vi "Text control 2 v5.5_pump-specific.vi"() -> ()   [LabVIEW 2016]
panel:
  in  "Tab Control":enum32{"Main", "Other parameters"}(tab)
  out "Line running":i32
  out "Total lines":i32
  out "Path":path=path "C:/users/rlp38/09Apr2009LTtesting/test2.txt"
  out "I vs Vg":cluster{"Y data in":dbl[], "X data in":dbl[]}[](graph)
  out "Is max":dbl format="%.2e"
  out "Id max":dbl format="%.2e"
  out "Ig max":dbl format="%.2e"
  out "Imax vs time":cluster{"Y data in":dbl[], "X data in":dbl[]}[](graph)
  out "Imin vs time":cluster{"Y data in":dbl[], "X data in":dbl[]}[](graph)
  out "I vs Vd":cluster{"Y data in":dbl[], "X data in":dbl[]}[](graph)
  in  "Script":string="#-------------------------------------------------------\n# SPM pump cleaning script\n#\n# Version 0.5\n# Author: Dimitrios Simatos\n# Last updated: 2018-01-05\n#-------------------------------------------------------\n# Description\n#\n# This script is designed to run the cleaning sequence of the SPM OEM pump.\n# This script needs to be run 4 times!\n#-------------------------------------------------------\n# Changes\n#\n# Placed initialization and hard stop commands in the beginning.\n#-------------------------------------------------------\n# Important points\n#\n# Never leave any liquid in the pump to dry after the experiments. If they dry, the residue may block the valve.\n# Always run the cleaning cycle after the experiments.\n# Use clockwise rotation when going up in valve port numbers and vice versa.\n#-------------------------------------------------------\n# Things to do before running the script\n#\n# Set time units to minutes.\n# Set filenames.\n# Replace the tubing, if necessary.\n#-------------------------------------------------------\n# Port connections\n#\n# Port 1: Waste\n# Port 2: Waste\n# Port 3: Various cleaning liquids\n# Port 4: Waste\n# Port 5: Waste\n# Port 6: Waste\n#\n# Between each of the 4 runs, the settings of Port 3 will change, according to the cleaning protocol.\n# The settings for Port 3 are:\n# 1st run: 1% v/v solution of sodium hypochlorite in ultrapure water\n# 2nd run: 0.1% w/v solution of sodium dodecyl sulfate in ultrapure water\n# 3rd run: Ultrapure water\n# 4th run: Waste (in air, not immersed in liquid)\n#-------------------------------------------------------\n# Cleaning protocol for the SPM OEM pump (from the manual)\n#\n# A cleaning procedure should be performed at the end of each day or in between two different experiments.\n# An effective cleaning can be performed in the following manner:\n# • Bleach solution to kill microorganisms\n# 1. Prepare a solution of 1% chlorine bleach and deionized water\n#    NOTE: Prepare a 1% v/v solution of sodium hypochlorite in deionized water\n# 2. Prepare a reservoir and place 1 tubing in the bleach solution and 5 tubings in a waste recipient\n# 3. Pick up the bleach solution through 1 port to entirely fill the syringe\n# 4. Sequentially output the syringe content through the remaining ports and throw it to the waste\n# 5. Repeat operation at least 2 times\n# • Detergent solution to remove debris\n# 1. Prepare a solution of 0.1% detergent and deionized water\n#    NOTE: Prepare a 0.1% w/v solution of sodium dodecyl sulfate in deionized water\n# 2. Move the tubing from the bleach solution reservoir and place it into a reservoir of detergent solution\n# 3. Pick up the detergent solution through 1 port to entirely fill the syringe\n# 4. Sequentially output the detergent solution through the remaining ports into the waste recipient\n# 5. Repeat operation at least 2 times\n# • Rinsing water to prepare the pump for your next experiment\n# 1. Move the tubing from the detergent solution reservoir and place it into a reservoir of deionized water\n# 2. Pick up the rinsing solution through 1 port to entirely fill the syringe\n# 3. Sequentially output the rinse water through the remaining ports into the waste recipient\n# 4. Repeat operation at least 2 times\n# • Replace the tubing, if necessary\n#-------------------------------------------------------\n# Pumping cycles and execution time\n#\n# Execution time for a single cycle: 6 x (1 min + 10 sec) = 7 minutes\n# Total execution time: 4 x 7 = 28 minutes\n# Since the script has to run 4 times, the cleaning lasts for: 4 x 28 = 112 minutes\n# Air must be the last to be pumped through the valve, to remove all liquids.\n# There are 4 pumping cycles. Each one draws a different liquid through port 3 and pumps it sequentially through ports 1,2,4,5,6.\n# During the sequential pumping, each port receives 200 ml of liquid (20% of the total syringe volume = 600 \"plunger units\")\n# The device must be disconnected from the port during the cleaning procedure.\n# All cycles are similar, except cycle 1 has the initialization command uncommented and the first report valve command commented.\n#-------------------------------------------------------\n# Volume of liquid needed\n#\n# Volume of liquid needed per cycle: 1 ml\n# Total volume of liquid needed per script run: 4 x 1 = 4 ml\n# Since the script has to run 4 times, the first 3 with different liquids, I need:\n# 4 ml of 1% v/v solution of sodium hypochlorite in ultrapure water\n# 4 ml of 0.1% w/v solution of sodium dodecyl sulfate in ultrapure water\n# 4 ml of ultrapure water\n#-------------------------------------------------------\n# Parameters\n#\n# Syringe size: 1 ml\n# Step resolution N = 0.01 mm\n# Drawing flow V = 300 pulses/second (6000 ul/min)\n# Pumping flow V = 300 pulses/second (6000 ul/min)\n#-------------------------------------------------------\n# Pump initialization\npump /1T #hard stop pump\npump /1ZR #initialize pump\n#-------------------------------------------------------\n# Cycle 1\n# Fill the syringe\npump /1Q #query pump\npump /1? #report absolute plunger position\n#pump /1?6 #report valve position\nwait-min 1 #wait 1 minute\npump /1N0R #set step resolution: 0.01 mm\npump /1Q #query pump\npump /1? #report absolute plunger position (the plunger should be at 0)\npump /1?6 #report valve position\nwait 1000 #wait 1 second\npump /1V300R #choose speed: 300 steps/s (6000 ul/min)\npump /1Q #query pump\nwait 1000 #wait 1 second\npump /1I3R #go to port 3, clockwise rotation\npump /1Q #query pump\npump /1?6 #report valve position\nwait 1000 #wait 1 second\npump /1A3000R #go to absolute position 3000 (= draw 1 ml)\nwait 30000 #wait 30 seconds\npump /1Q #query pump\npump /1? #report absolute plunger position (the plunger should have finished moving)\n#pump /1?6 #report valve position\n# The sequential pumping begins\n# Port 1\npump /1O1R #switch to port 1, counterclockwise rotation\npump /1Q #query pump\npump /1?6 #report valve position\npump /1A2400R #go to absolute position 2400 (= pump 200 ul)\npump /1Q #query pump\npump /1? #report absolute plunger position (the plunger should be moving to 0)\nwait-min 1 #wait 1 minute\npump /1? #report absolute plunger position (the plunger should have finished moving)\n# Port 2\npump /1I2R #switch to port 2, clockwise rotation\npump /1Q #query pump\npump /1?6 #report valve position\npump /1A1800R #go to absolute position 1800 (= pump 200 ul)\npump /1Q #query pump\npump /1? #report absolute plunger position (the plunger should be moving to 0)\nwait-min 1 #wait 1 minute\npump /1? #report absolute plunger position (the plunger should have finished moving)\n# Port 4\npump /1I4R #switch to port 4, clockwise rotation\npump /1Q #query pump\npump /1?6 #report valve position\npump /1A1200R #go to absolute position 1200 (= pump 200 ul)\npump /1Q #query pump\npump /1? #report absolute plunger position (the plunger should be moving to 0)\nwait-min 1 #wait 1 minute\npump /1? #report absolute plunger position (the plunger should have finished moving)\n# Port 5\npump /1I5R #switch to port 5, clockwise rotation\npump /1Q #query pump\npump /1?6 #report valve position\npump /1A600R #go to absolute position 600 (= pump 200 ul)\npump /1Q #query pump\npump /1? #report absolute plunger position (the plunger should be moving to 0)\nwait-min 1 #wait 1 minute\npump /1? #report absolute plunger position (the plunger should have finished moving)\n# Port 6\npump /1I6R #switch to port 6, clockwise rotation\npump /1Q #query pump\npump /1?6 #report valve position\npump /1A0R #go to absolute position 0 (= pump 200 ul)\npump /1Q #query pump\npump /1? #report absolute plunger position (the plunger should be moving to 0)\nwait-min 1 #wait 1 minute\npump /1? #report absolute plunger position (the plunger should have finished moving)\n#-------------------------------------------------------\n# Cycle 2\n# Fill the syringe\n#pump /1ZR #initialize pump\npump /1Q #query pump\npump /1? #report absolute plunger position\npump /1?6 #report valve position\nwait-min 1 #wait 1 minute\npump /1N0R #set step resolution: 0.01 mm\npump /1Q #query pump\npump /1? #report absolute plunger position (the plunger should be at 0)\npump /1?6 #report valve position\nwait 1000 #wait 1 second\npump /1V300R #choose speed: 300 steps/s (6000 ul/min)\npump /1Q #query pump\nwait 1000 #wait 1 second\npump /1O3R #go to port 3, counterclockwise rotation\npump /1Q #query pump\npump /1?6 #report valve position\nwait 1000 #wait 1 second\npump /1A3000R #go to absolute position 3000 (= draw 1 ml)\nwait 30000 #wait 30 seconds\npump /1Q #query pump\npump /1? #report absolute plunger position (the plunger should have finished moving)\n#pump /1?6 #report valve position\n# The sequential pumping begins\n# Port 1\npump /1O1R #switch to port 1, counterclockwise rotation\npump /1Q #query pump\npump /1?6 #report valve position\npump /1A2400R #go to absolute position 2400 (= pump 200 ul)\npump /1Q #query pump\npump /1? #report absolute plunger position (the plunger should be moving to 0)\nwait-min 1 #wait 1 minute\npump /1? #report absolute plunger position (the plunger should have finished moving)\n# Port 2\npump /1I2R #switch to port 2, clockwise rotation\npump /1Q #query pump\npump /1?6 #report valve position\npump /1A1800R #go to absolute position 1800 (= pump 200 ul)\npump /1Q #query pump\npump /1? #report absolute plunger position (the plunger should be moving to 0)\nwait-min 1 #wait 1 minute\npump /1? #report absolute plunger position (the plunger should have finished moving)\n# Port 4\npump /1I4R #switch to port 4, clockwise rotation\npump /1Q #query pump\npump /1?6 #report valve position\npump /1A1200R #go to absolute position 1200 (= pump 200 ul)\npump /1Q #query pump\npump /1? #report absolute plunger position (the plunger should be moving to 0)\nwait-min 1 #wait 1 minute\npump /1? #report absolute plunger position (the plunger should have finished moving)\n# Port 5\npump /1I5R #switch to port 5, clockwise rotation\npump /1Q #query pump\npump /1?6 #report valve position\npump /1A600R #go to absolute position 600 (= pump 200 ul)\npump /1Q #query pump\npump /1? #report absolute plunger position (the plunger should be moving to 0)\nwait-min 1 #wait 1 minute\npump /1? #report absolute plunger position (the plunger should have finished moving)\n# Port 6\npump /1I6R #switch to port 6, clockwise rotation\npump /1Q #query pump\npump /1?6 #report valve position\npump /1A0R #go to absolute position 0 (= pump 200 ul)\npump /1Q #query pump\npump /1? #report absolute plunger position (the plunger should be moving to 0)\nwait-min 1 #wait 1 minute\npump /1? #report absolute plunger position (the plunger should have finished moving)\n#-------------------------------------------------------\n# Cycle 3\n# Fill the syringe\n#pump /1ZR #initialize pump\npump /1Q #query pump\npump /1? #report absolute plunger position\npump /1?6 #report valve position\nwait-min 1 #wait 1 minute\npump /1N0R #set step resolution: 0.01 mm\npump /1Q #query pump\npump /1? #report absolute plunger position (the plunger should be at 0)\npump /1?6 #report valve position\nwait 1000 #wait 1 second\npump /1V300R #choose speed: 300 steps/s (6000 ul/min)\npump /1Q #query pump\nwait 1000 #wait 1 second\npump /1O3R #go to port 3, counterclockwise rotation\npump /1Q #query pump\npump /1?6 #report valve position\nwait 1000 #wait 1 second\npump /1A3000R #go to absolute position 3000 (= draw 1 ml)\nwait 30000 #wait 30 seconds\npump /1Q #query pump\npump /1? #report absolute plunger position (the plunger should have finished moving)\n#pump /1?6 #report valve position\n# The sequential pumping begins\n# Port 1\npump /1O1R #switch to port 1, counterclockwise rotation\npump /1Q #query pump\npump /1?6 #report valve position\npump /1A2400R #go to absolute position 2400 (= pump 200 ul)\npump /1Q #query pump\npump /1? #report absolute plunger position (the plunger should be moving to 0)\nwait-min 1 #wait 1 minute\npump /1? #report absolute plunger position (the plunger should have finished moving)\n# Port 2\npump /1I2R #switch to port 2, clockwise rotation\npump /1Q #query pump\npump /1?6 #report valve position\npump /1A1800R #go to absolute position 1800 (= pump 200 ul)\npump /1Q #query pump\npump /1? #report absolute plunger position (the plunger should be moving to 0)\nwait-min 1 #wait 1 minute\npump /1? #report absolute plunger position (the plunger should have finished moving)\n# Port 4\npump /1I4R #switch to port 4, clockwise rotation\npump /1Q #query pump\npump /1?6 #report valve position\npump /1A1200R #go to absolute position 1200 (= pump 200 ul)\npump /1Q #query pump\npump /1? #report absolute plunger position (the plunger should be moving to 0)\nwait-min 1 #wait 1 minute\npump /1? #report absolute plunger position (the plunger should have finished moving)\n# Port 5\npump /1I5R #switch to port 5, clockwise rotation\npump /1Q #query pump\npump /1?6 #report valve position\npump /1A600R #go to absolute position 600 (= pump 200 ul)\npump /1Q #query pump\npump /1? #report absolute plunger position (the plunger should be moving to 0)\nwait-min 1 #wait 1 minute\npump /1? #report absolute plunger position (the plunger should have finished moving)\n# Port 6\npump /1I6R #switch to port 6, clockwise rotation\npump /1Q #query pump\npump /1?6 #report valve position\npump /1A0R #go to absolute position 0 (= pump 200 ul)\npump /1Q #query pump\npump /1? #report absolute plunger position (the plunger should be moving to 0)\nwait-min 1 #wait 1 minute\npump /1? #report absolute plunger position (the plunger should have finished moving)\n#-------------------------------------------------------\n# Cycle 4\n# Fill the syringe\n#pump /1ZR #initialize pump\npump /1Q #query pump\npump /1? #report absolute plunger position\npump /1?6 #report valve position\nwait-min 1 #wait 1 minute\npump /1N0R #set step resolution: 0.01 mm\npump /1Q #query pump\npump /1? #report absolute plunger position (the plunger should be at 0)\npump /1?6 #report valve position\nwait 1000 #wait 1 second\npump /1V300R #choose speed: 300 steps/s (6000 ul/min)\npump /1Q #query pump\nwait 1000 #wait 1 second\npump /1O3R #go to port 3, counterclockwise rotation\npump /1Q #query pump\npump /1?6 #report valve position\nwait 1000 #wait 1 second\npump /1A3000R #go to absolute position 3000 (= draw 1 ml)\nwait 30000 #wait 30 seconds\npump /1Q #query pump\npump /1? #report absolute plunger position (the plunger should have finished moving)\n#pump /1?6 #report valve position\n# The sequential pumping begins\n# Port 1\npump /1O1R #switch to port 1, counterclockwise rotation\npump /1Q #query pump\npump /1?6 #report valve position\npump /1A2400R #go to absolute position 2400 (= pump 200 ul)\npump /1Q #query pump\npump /1? #report absolute plunger position (the plunger should be moving to 0)\nwait-min 1 #wait 1 minute\npump /1? #report absolute plunger position (the plunger should have finished moving)\n# Port 2\npump /1I2R #switch to port 2, clockwise rotation\npump /1Q #query pump\npump /1?6 #report valve position\npump /1A1800R #go to absolute position 1800 (= pump 200 ul)\npump /1Q #query pump\npump /1? #report absolute plunger position (the plunger should be moving to 0)\nwait-min 1 #wait 1 minute\npump /1? #report absolute plunger position (the plunger should have finished moving)\n# Port 4\npump /1I4R #switch to port 4, clockwise rotation\npump /1Q #query pump\npump /1?6 #report valve position\npump /1A1200R #go to absolute position 1200 (= pump 200 ul)\npump /1Q #query pump\npump /1? #report absolute plunger position (the plunger should be moving to 0)\nwait-min 1 #wait 1 minute\npump /1? #report absolute plunger position (the plunger should have finished moving)\n# Port 5\npump /1I5R #switch to port 5, clockwise rotation\npump /1Q #query pump\npump /1?6 #report valve position\npump /1A600R #go to absolute position 600 (= pump 200 ul)\npump /1Q #query pump\npump /1? #report absolute plunger position (the plunger should be moving to 0)\nwait-min 1 #wait 1 minute\npump /1? #report absolute plunger position (the plunger should have finished moving)\n# Port 6\npump /1I6R #switch to port 6, clockwise rotation\npump /1Q #query pump\npump /1?6 #report valve position\npump /1A0R #go to absolute position 0 (= pump 200 ul)\npump /1Q #query pump\npump /1? #report absolute plunger position (the plunger should be moving to 0)\nwait-min 1 #wait 1 minute\npump /1? #report absolute plunger position (the plunger should have finished moving)\n#-------------------------------------------------------"
  out "Command running:":string
  out "Serial port data":string
  out "Elapsed Time":dbl caption="Elapsed Time (s)"
  in  "Units":u16(ring)=1 items=["Seconds", "Minutes", "Hours"]
  in  "Time Offset":dbl caption="Set Start Time (s)"
  in  "Reset":bool
  in  "Auto Reset":bool
  in  "integration time":u32(slide) max=2 step=1 scale=0.0..2.0
  in  "Interrupt run":bool
  out "Absolute plunger position vs time":cluster{"Y data in":dbl[], "X data in":dbl[]}[](graph)
  out "Valve position vs time":cluster{"Y data in":dbl[], "X data in":dbl[]}[](graph)
  in  "Halt pump":bool
  in  "Hard stop pump":bool
  out "Is on":dbl format="%.2e"
  out "Id on":dbl format="%.2e"
  out "Ig on":dbl format="%.2e"
  out "Ion vs time":cluster{"Y data in":dbl[], "X data in":dbl[]}[](graph)
  out "Ioff vs time":cluster{"Y data in":dbl[], "X data in":dbl[]}[](graph)
  out "Ig min":dbl format="%.2e"
  out "Id min":dbl format="%.2e"
  out "Is min":dbl format="%.2e"
  out "Is off":dbl format="%.2e"
  out "Id off":dbl format="%.2e"
  out "Ig off":dbl format="%.2e"
  in  "Gate Range\nmode":u16(ring) items=["Auto", "Limited", "Fixed"]
  in  "Gate Range":u8(slide)=6 max=11 scale=0.0..11.0
  in  "Source/Drain\nRange mode":u16(ring) items=["Auto", "Limited", "Fixed"]
  in  "Source/Drain Range":u8(slide)=6 max=11 scale=0.0..11.0
  in  "Panel Controls":T1={"Emergency Stop"=refnum, "TransGraph Max"=1e-05, "Text/Graph (text=false)"=TRUE} {"TransGraph Max" format="%.2e"}
  in  "Panel Controls 2":T2={"Emergency Stop"=refnum, "TransGraph Max"=1e-05, "Text/Graph (text=false)"=TRUE, "TransGraph Min"=1e-11} {"TransGraph Min" format="%.2e"; "TransGraph Max" format="%.2e"}
  in  "SMU4":cluster{"on/off":bool, "Voltage":dbl} {"Voltage" min=-100.0 max=100.0 format="%.2f"}
  in  "Full Reset":bool
  in  "Standby":T3
  out "error out":errorcluster
  in  "Delay before read (ms)":u32=1000
  in  "byte count":u32=64
  in  "Serial End Mode for Reads":u16(ring)=2 items=["None", "LastBit", "TermChar"]
  in  "Timeout (ms)":u32=10000
  in  "Enable Termination\nChar (T)":bool=TRUE
  in  "Termination char\n(0xA = '\\n' = LF)\n(0xD = '\\r' = CR)":u8=13 format="%.0x"
  in  "flow control":u16(ring) items=["None"=0, "XON/XOFF"=1, "RTS/CTS"=2, "DTR/DSR"=4]
  in  "stop bits":u16(ring)=10 items=["1.0"=10, "1.5"=15, "2.0"=20]
  in  "parity":u16(ring) items=["None", "Odd", "Even", "Mark", "Space"]
  in  "data bits":u16=8 min=5 max=8 step=1
  in  "VISA resource name":refnum<visa-resource-name>="COM6"
  in  "baud rate":u32=9600
  in  "Drain: Compliance":dbl=0.001 format="%.8f"
  in  "Gate: Compliance":dbl=0.001 format="%.8f"
  in  "hold time /s":dbl format="%.2f"
  in  "delay time /s":dbl format="%.2f"
  in  "Integration time (short)":dbl=0.0019 min=8e-05 max=0.0019 step=8e-05 format="%^.0e"
  in  "Integration time (long)":dbl=0.32 min=0.04 max=2.0 step=0.02 format="%.2f"
  in  "Step delay /s":dbl format="%.2f"
  in  "Filename (variable part)":string="step_1_up-H2O_initial_"
  in  "Suffix (script)":string="step_1_up-H2O_initial_script.txt"
  in  "Gate":T4={"Gate Start"=0.0, "Gate Stop"=2.0, "Gate Step (linear only)"=1.0, "Gate Compliance"=0.0001, "Gate PComp"=0.0, "Range mode"=0, "Range"=6} {"Range" max=11 scale=0.0..11.0; "Range mode" items=["Auto", "Limited", "Fixed"]; "Gate PComp" format="%^.2e"; "Gate Compliance" format="%^.2e"; "Gate Step (linear only)" format="%^.4e"; "Gate Stop" format="%^.4e"; "Gate Start" format="%^.4e"}
  in  "Drain 2":T5={"Drain Start"=0.0, "Drain Stop"=2.0, "Drain Compliance"=0.0001, "Drain Step"=1.0, "Drain PComp"=0.0, "Range mode"=0, "Range"=6} {"Range" max=11 scale=0.0..11.0; "Range mode" items=["Auto", "Limited", "Fixed"]; "Drain PComp" format="%^.2e"; "Drain Step" format="%^.4e"; "Drain Compliance" format="%^.2e"; "Drain Stop" format="%^.4e"; "Drain Start" format="%^.4e"}
  in  "Timings 2":T6={"integration time"=0, "Short/Long integration time"=0.00064, "hold time (sec)"=0.0, "delay time (sec)"=0.0, "Step Time (0 disables)"=0.0, "sweep method"=0, "Pulse period"=0.005, "Base voltage"=0.0, "Pulse width"=0.0005} {"Pulse width" min=0.0005 max=0.1 step=0.0001 format="%.4f"; "Base voltage" format="%^.4e"; "Pulse period" min=0.005 max=1.0 step=0.0001 format="%.4f"; "sweep method" items=["Continuous", "Pulsed"]; "Step Time (0 disables)" format="%.2f"; "delay time (sec)" format="%.4f"; "hold time (sec)" format="%.4f"; "Short/Long integration time" format="%^.0e"; "integration time" scale=0.0..2.0}
  # "Syntax:\nitime [s|m|l]\ngaterangemode [a|l|f]\ndrainrangemode [a|l|f]\npulsed [on|off] PulsePeriod(sec) PulseBaseVoltage PulseONWidth(sec)\nstandby [on l off]\nwait NumMilliseconds\nwait-min NumMinutes\n# texthere = comment\ntransfer [s|d] VgStart VgStop VgStep VdStart VdStop VdStep\noutput [s|d] VgStart VgStop VgStep VdStart VdStop VdStep\nsample Vg Vd NumSamples Time(s) SampleInterval(s)\nsamplei Idg NumSamples Time(s) SampleInterval(s) VDGcompliance\n100 samples is approximately 13 seconds with medium integration\n# if in doubt use SampleInterval(s) = 0.004\nstressV VG VD IGcompliance IDcompliance Duration(sec)\nstressI IDG VDGcompliance Duration(sec)\nvsu2pulse Bias Duration(s)\npulsedstressV [s|d] VEstop VgON VgOFF Period(s) PulseONwidth(s) Vd\nsample-fpp Vg Vd NumSamples Time\nresample-fpp Vg Vd\ntransfer-fpp [s|d] VgStart VgStop VgStep VdStart VdStop VdStep\noutput-fpp [s|d] VgStart VgStop VgStep VdStart VdStop VdStep\nserial SerialPortCommand\npump SerialPortCommand for the SPM pump\n\nSPM Pump Syntax (<x>: pump number, use 1 if only one pump):\nif the command syntax contains [R], then append the letter R to the command\n/<x>Q: query (a query command should follow each command)\n/<x>Z[R] or /<x>Y[R]: initialize pump\n/<x>N<n>[R] (<n>=0,1): <0> (<1>) microstep 0.01 mm (0.00125 mm) resolution\n/<x>I<n> (<n>=0-6): turn to port number n (clockwise)\n/<x>O<n> (<n>=0-6): turn to port number n (counterclockwise)\n/<x>X: Re-execute last command string\n/<x>G<n>[R] (<n>=0-60000): repeat command sequence (default: 0, 0=loop forever)\n/<x>g: Mark the start of a repeat sequence (max = 10)\n/<x>M<n>[R] (<n>=0-86400000): delay command execution by n milliseconds\n/<x>H: Halt; Pause the sequence after finishing the current move\n/<x>T: Hardstop; Interrupt the current move and suppress it from the sequence\n/<x>A<n>[R] (<n>=0-3000 with N=0, 0-24000 with N=1): absolute position\n/<x>P<n>[R] (<n>=0-3000 with N=0, 0-24000 with N=1): relative pickup\n/<x>D<n>[R] (<n>=0-3000 with N=0, 0-24000 with N=1): relative dispense\n/<x>V<n>[R] (<n>=1-1600 default: 150): set peak speed (pulses/sec)\nNOTE: The lowest speed limit is 1 pulse/sec, not 5, as the manual states.\n/<x>S<n>[R] (<n>=10-40 default: 22): set speed (NOT in pulses/sec, look in manual)\nNOTE: When controlled with absolute position, one does not need to pay special attention to the syringe that is mounted on the pump.\nWithdraw from lower stage (ports 3, 5), dispense from higher stage (ports 2, 4, 6).\nConnect Port 1 to waste."
  # "Time"
  # "1\n2\n3\n4\n5\n6\n7\n8\n9\n10\n11\n12\n13\n14\n15\n16\n17\n18\n19\n20"
  # "Serial port settings"
  # "Filename settings"
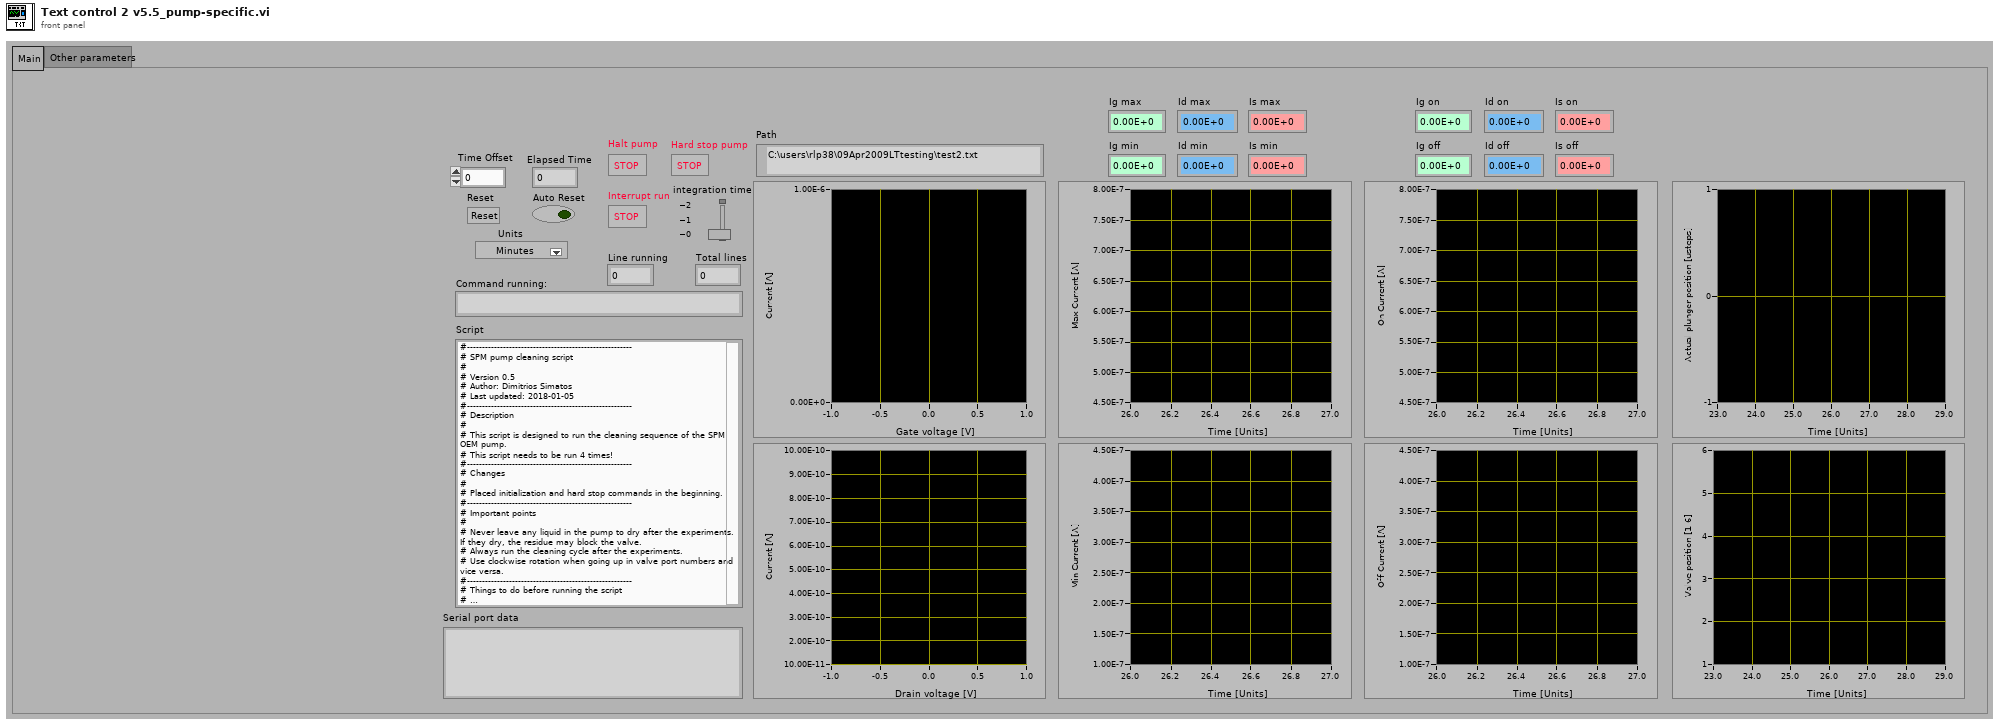
[diagram p1: front panel]
types:
  T1 = cluster{"Emergency Stop":refnum<vi>, "TransGraph Max":dbl, "Text/Graph (text=false)":bool}
  T2 = cluster{"Emergency Stop":refnum<vi>, "TransGraph Max":dbl, "Text/Graph (text=false)":bool, "TransGraph Min":dbl}
  T3 = cluster{"Gate Standby":bool, "Drain Standby":bool}
  T4 = cluster{"Gate Start":dbl, "Gate Stop":dbl, "Gate Step (linear only)":dbl, "Gate Compliance":dbl, "Gate PComp":dbl, "Range mode":u16, "Range":u8}
  T5 = cluster{"Drain Start":dbl, "Drain Stop":dbl, "Drain Compliance":dbl, "Drain Step":dbl, "Drain PComp":dbl, "Range mode":u16, "Range":u8}
  T6 = cluster{"integration time":u32, "Short/Long integration time":dbl, "hold time (sec)":dbl, "delay time (sec)":dbl, "Step Time (0 disables)":dbl, "sweep method":u16, "Pulse period":dbl, "Base voltage":dbl, "Pulse width":dbl}
  T7 = enum16{"open", "replace", "create", "open or create", "replace or create", "replace or create with confirmation"}
  T8 = cluster{"V2 Start":dbl, "V2 Step":dbl, "Number of points":i32}
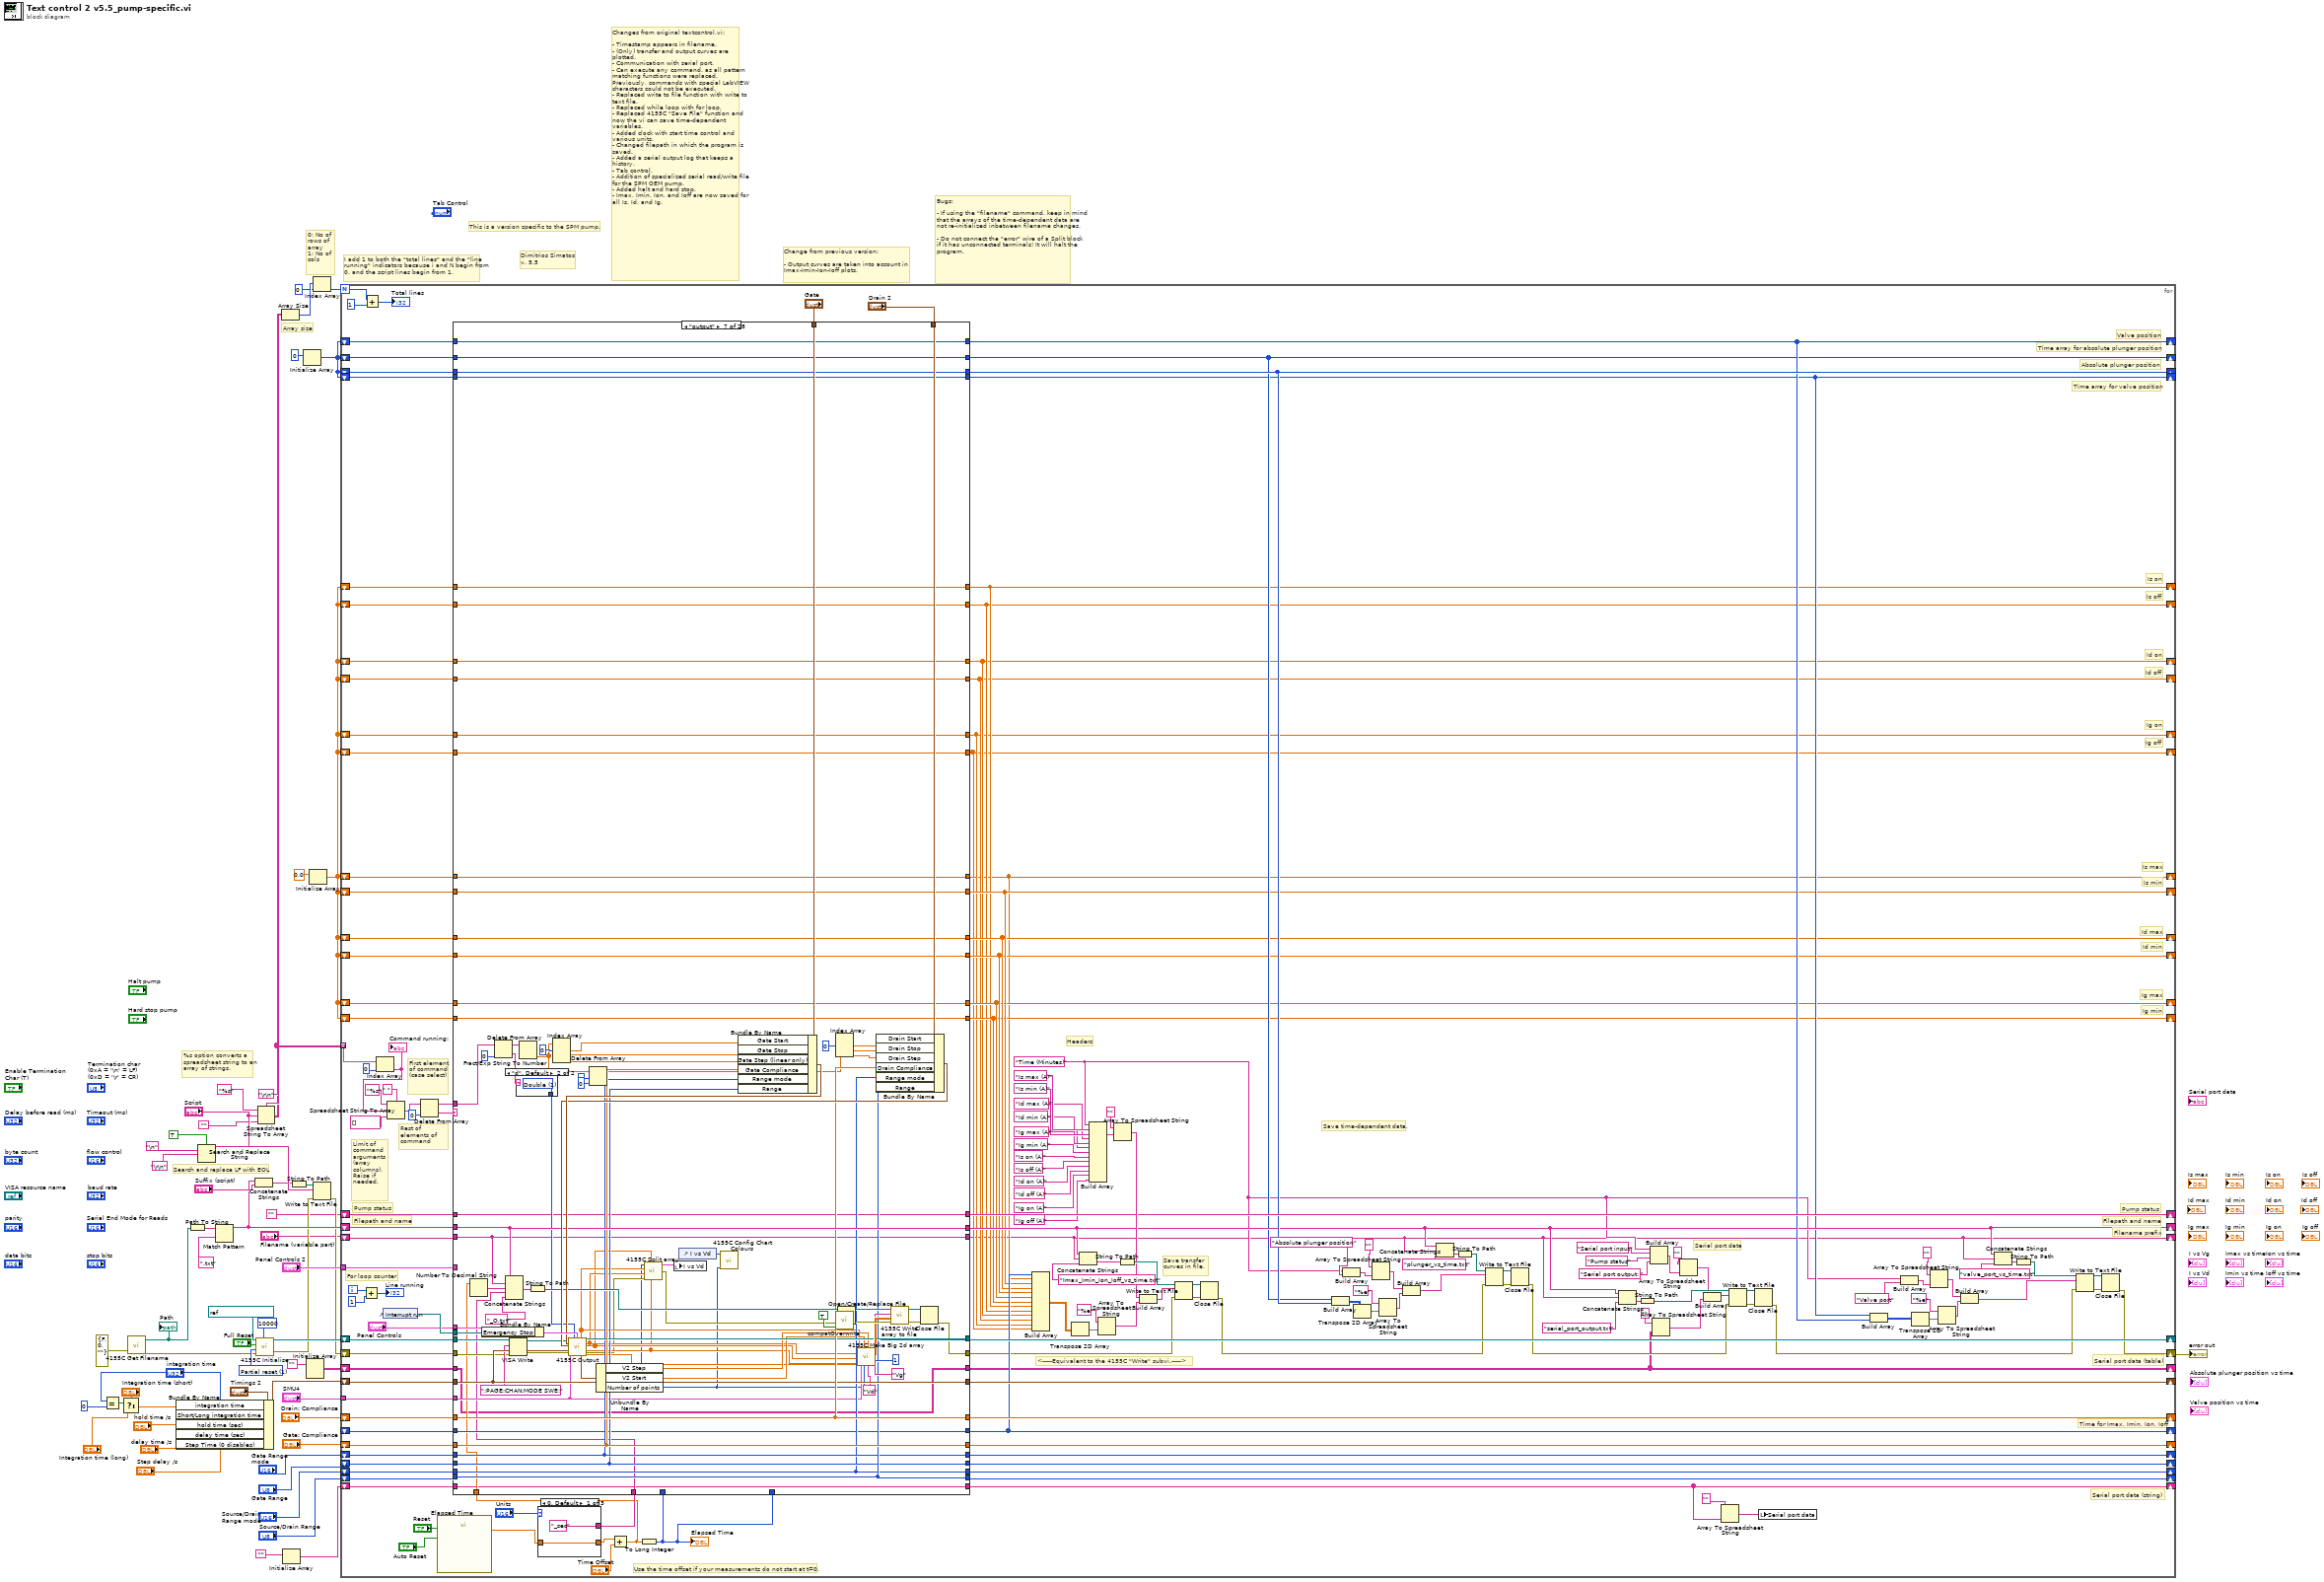
[diagram p0: block diagram]
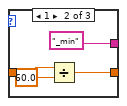
[diagram p2: hidden frame]
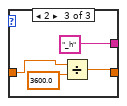
[diagram p3: hidden frame]
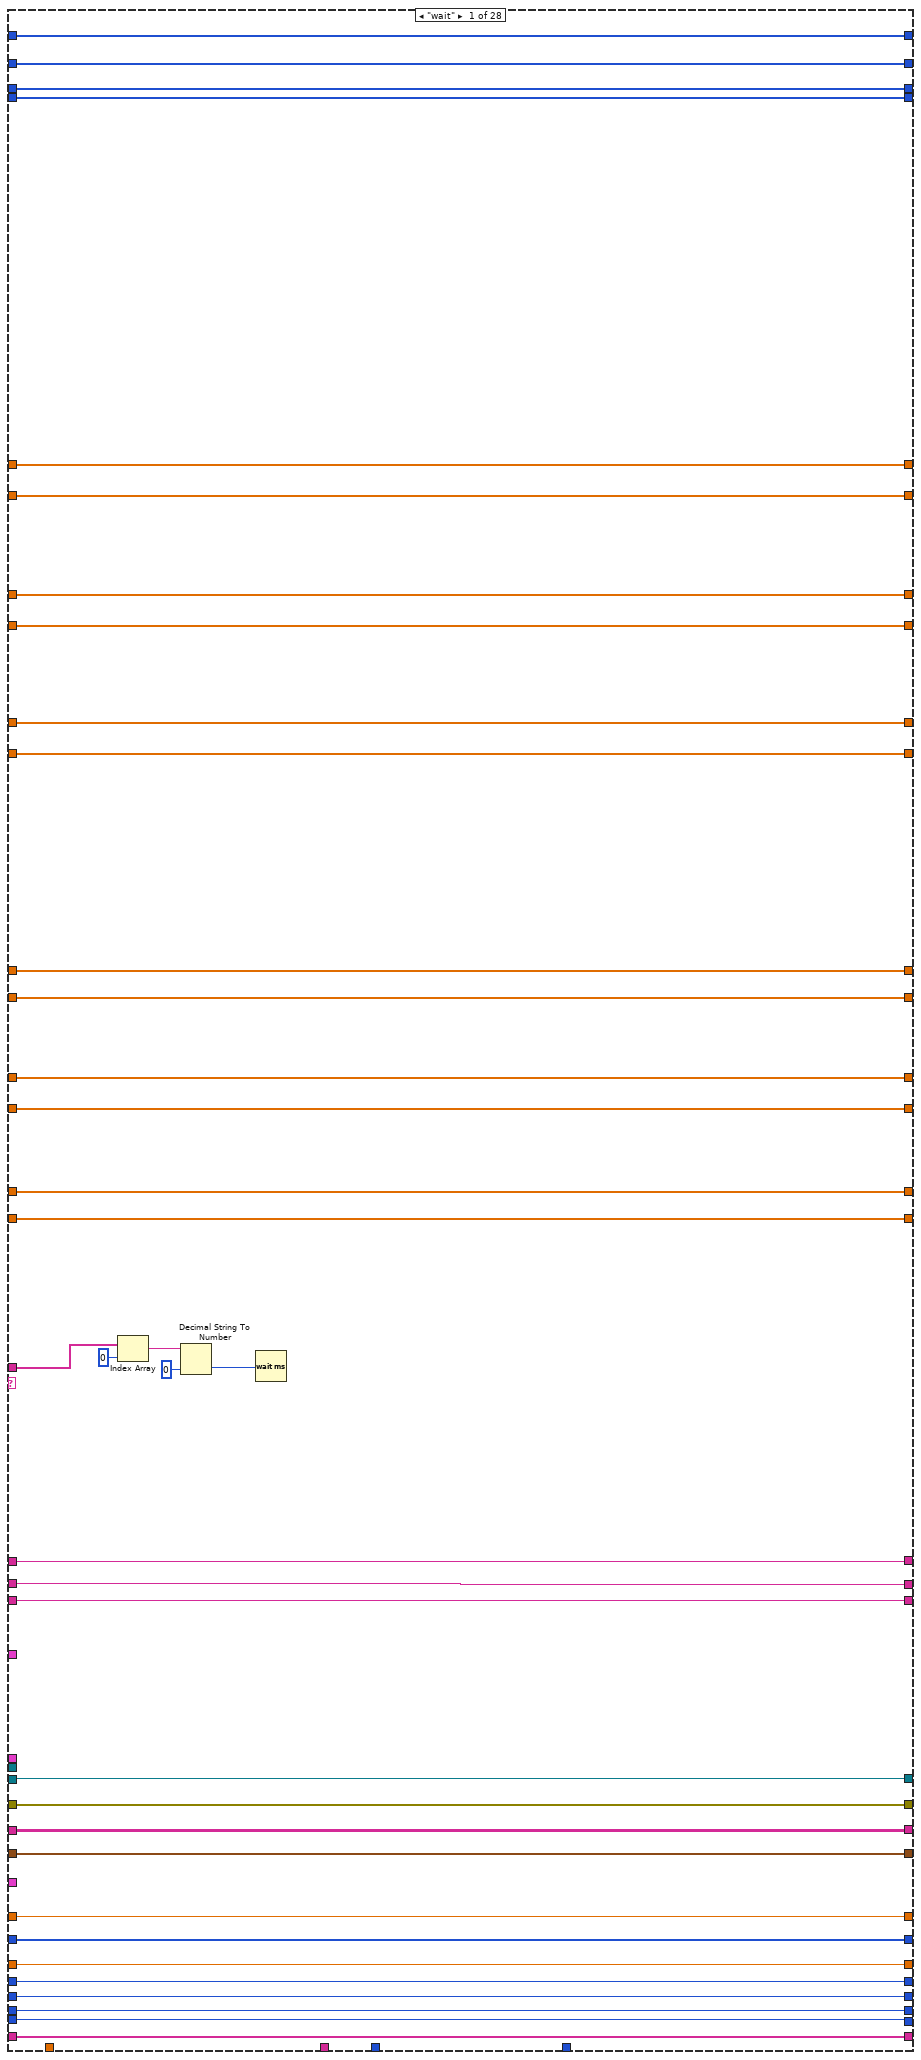
[diagram p4: hidden frame]
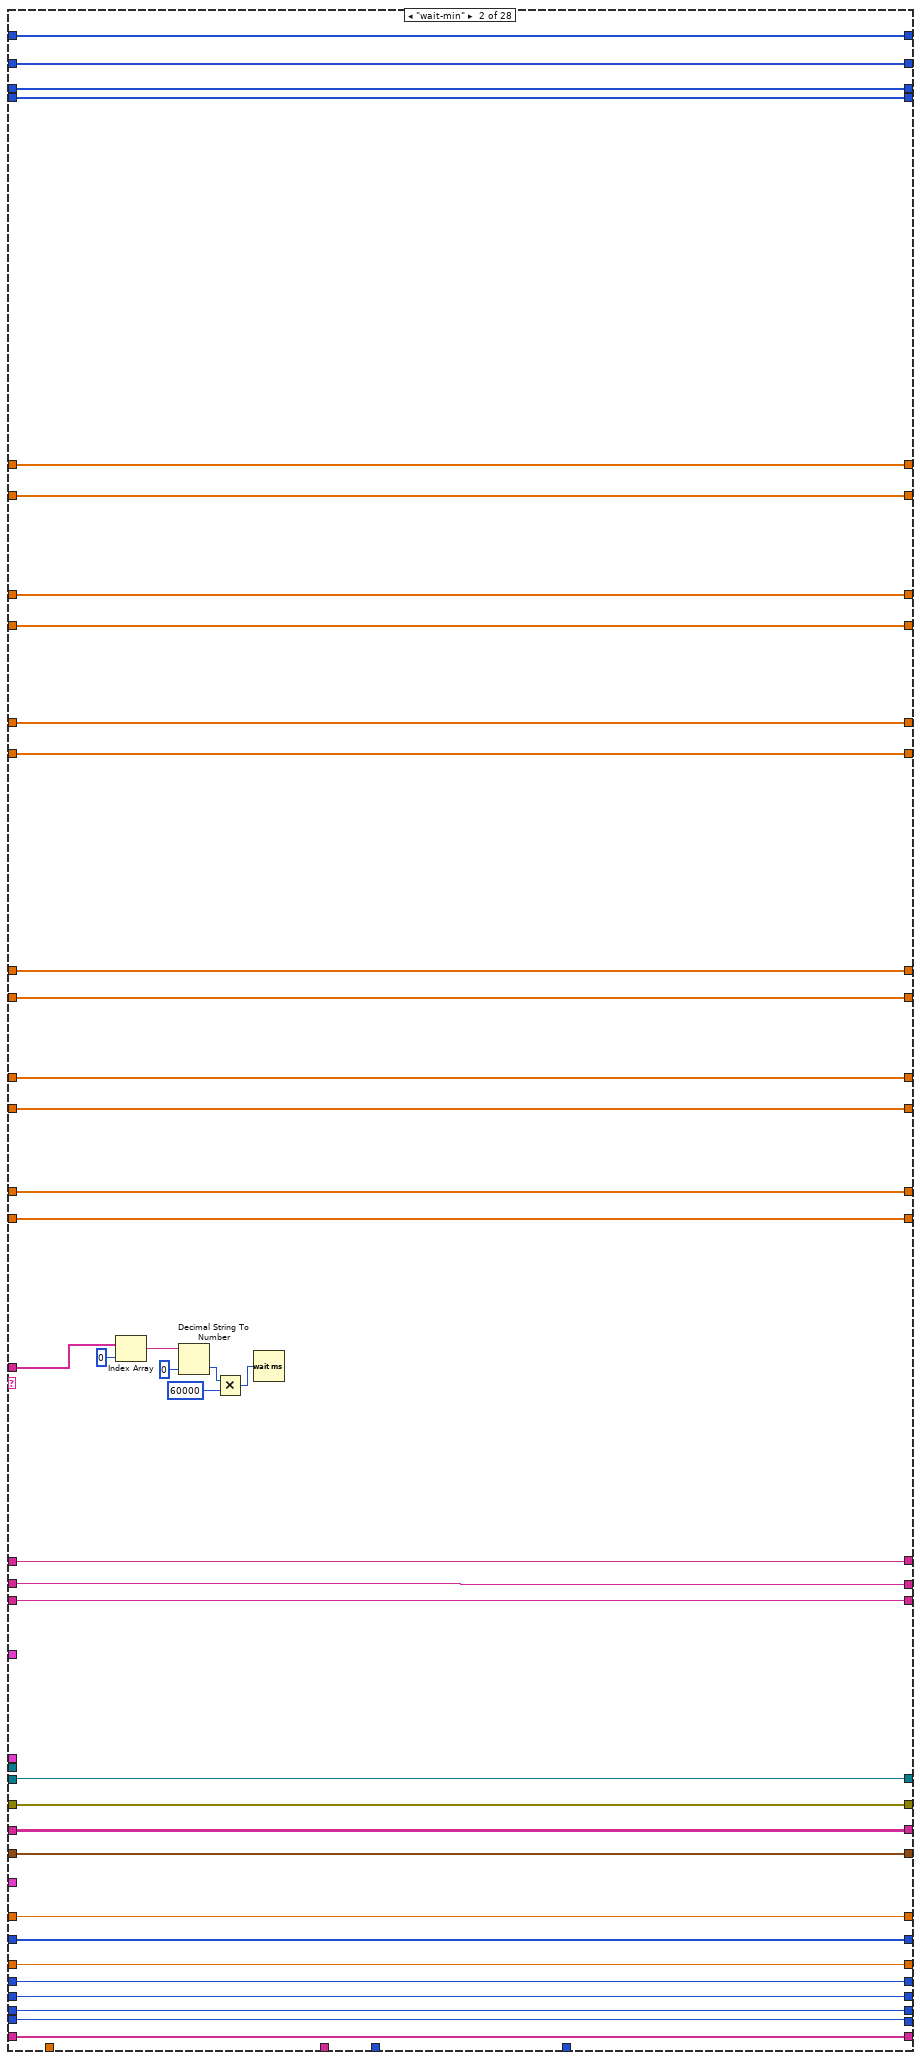
[diagram p5: hidden frame]
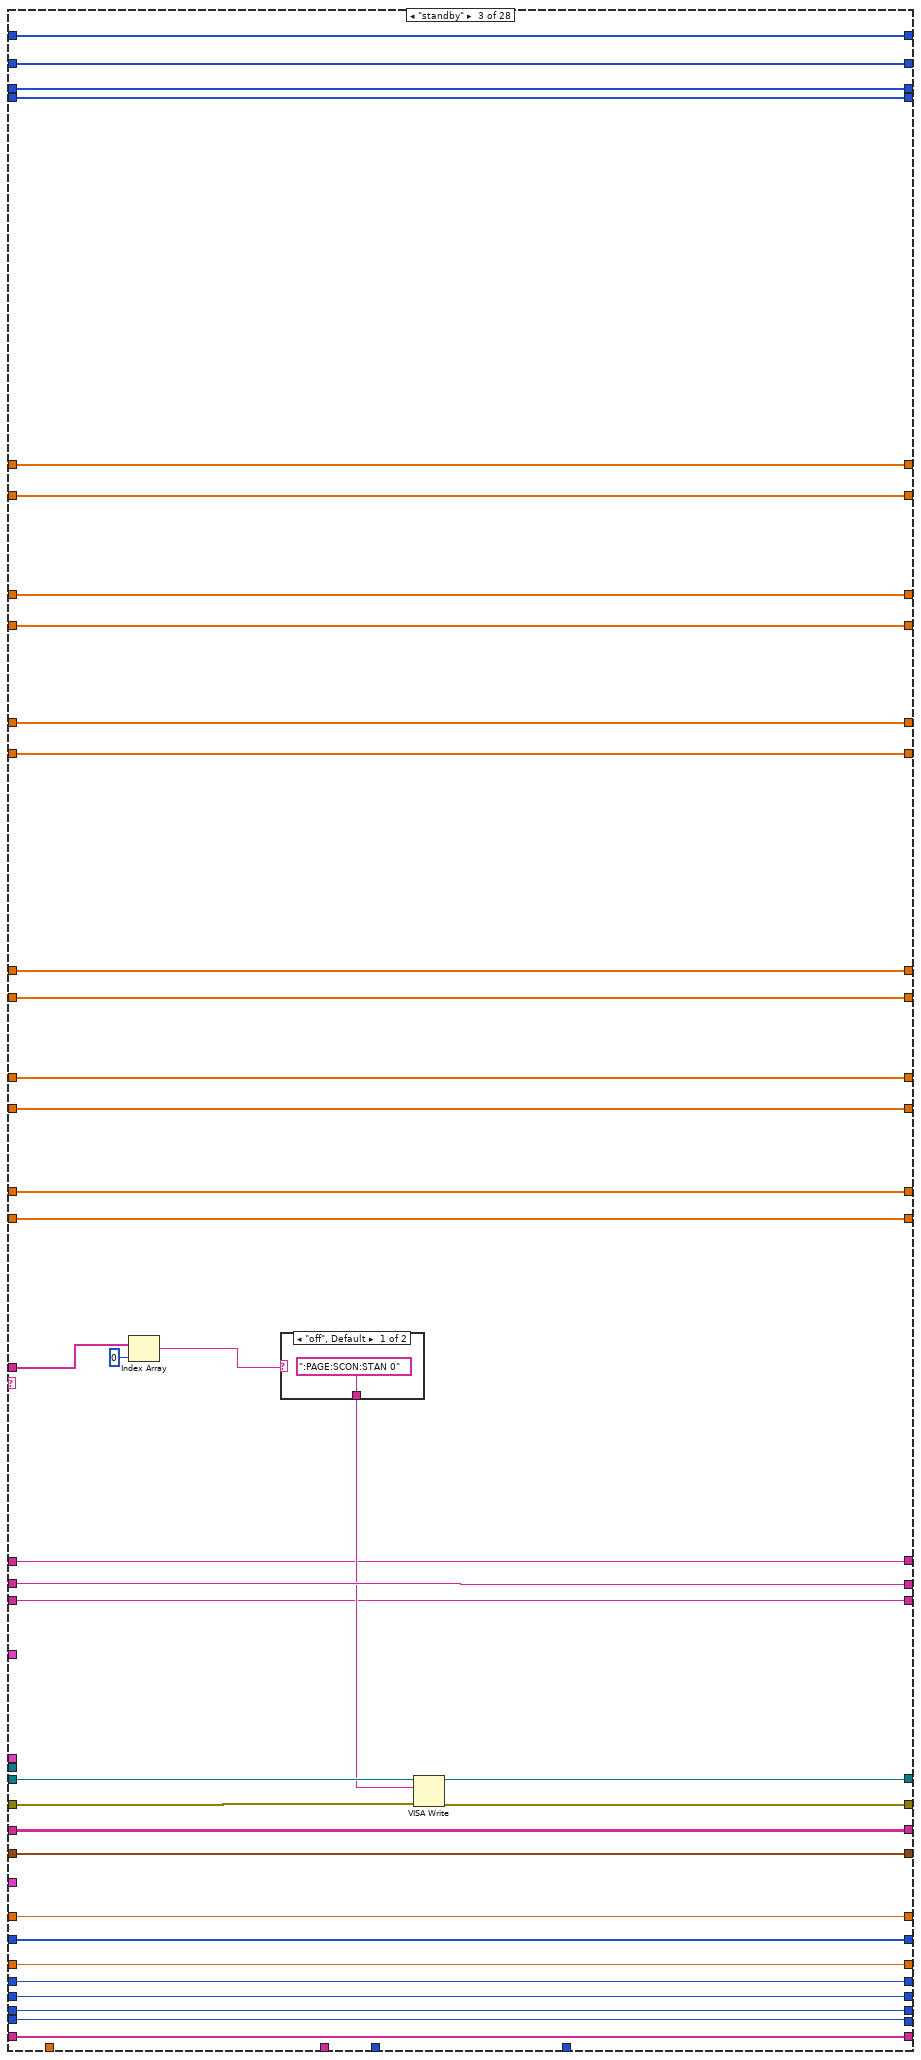
[diagram p6: hidden frame]
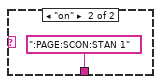
[diagram p7: hidden frame]
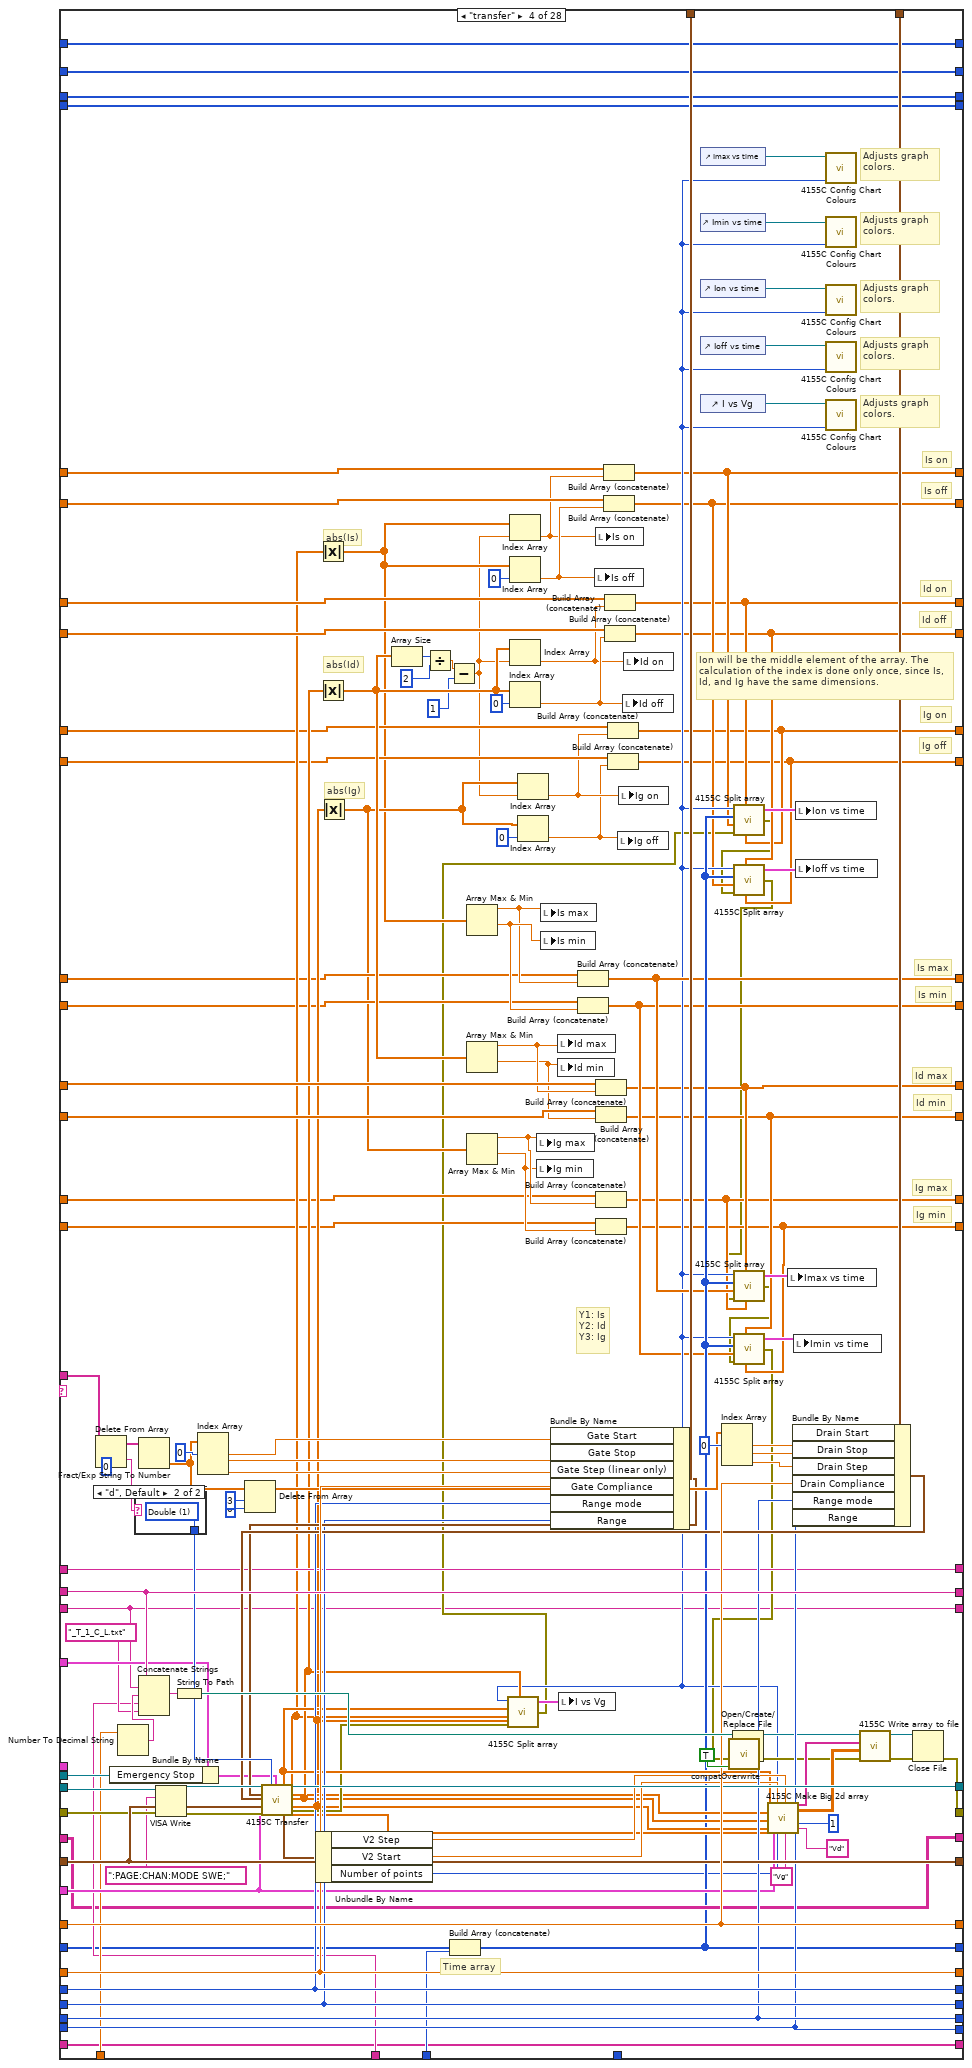
[diagram p8: hidden frame]
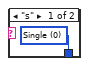
[diagram p9: hidden frame]
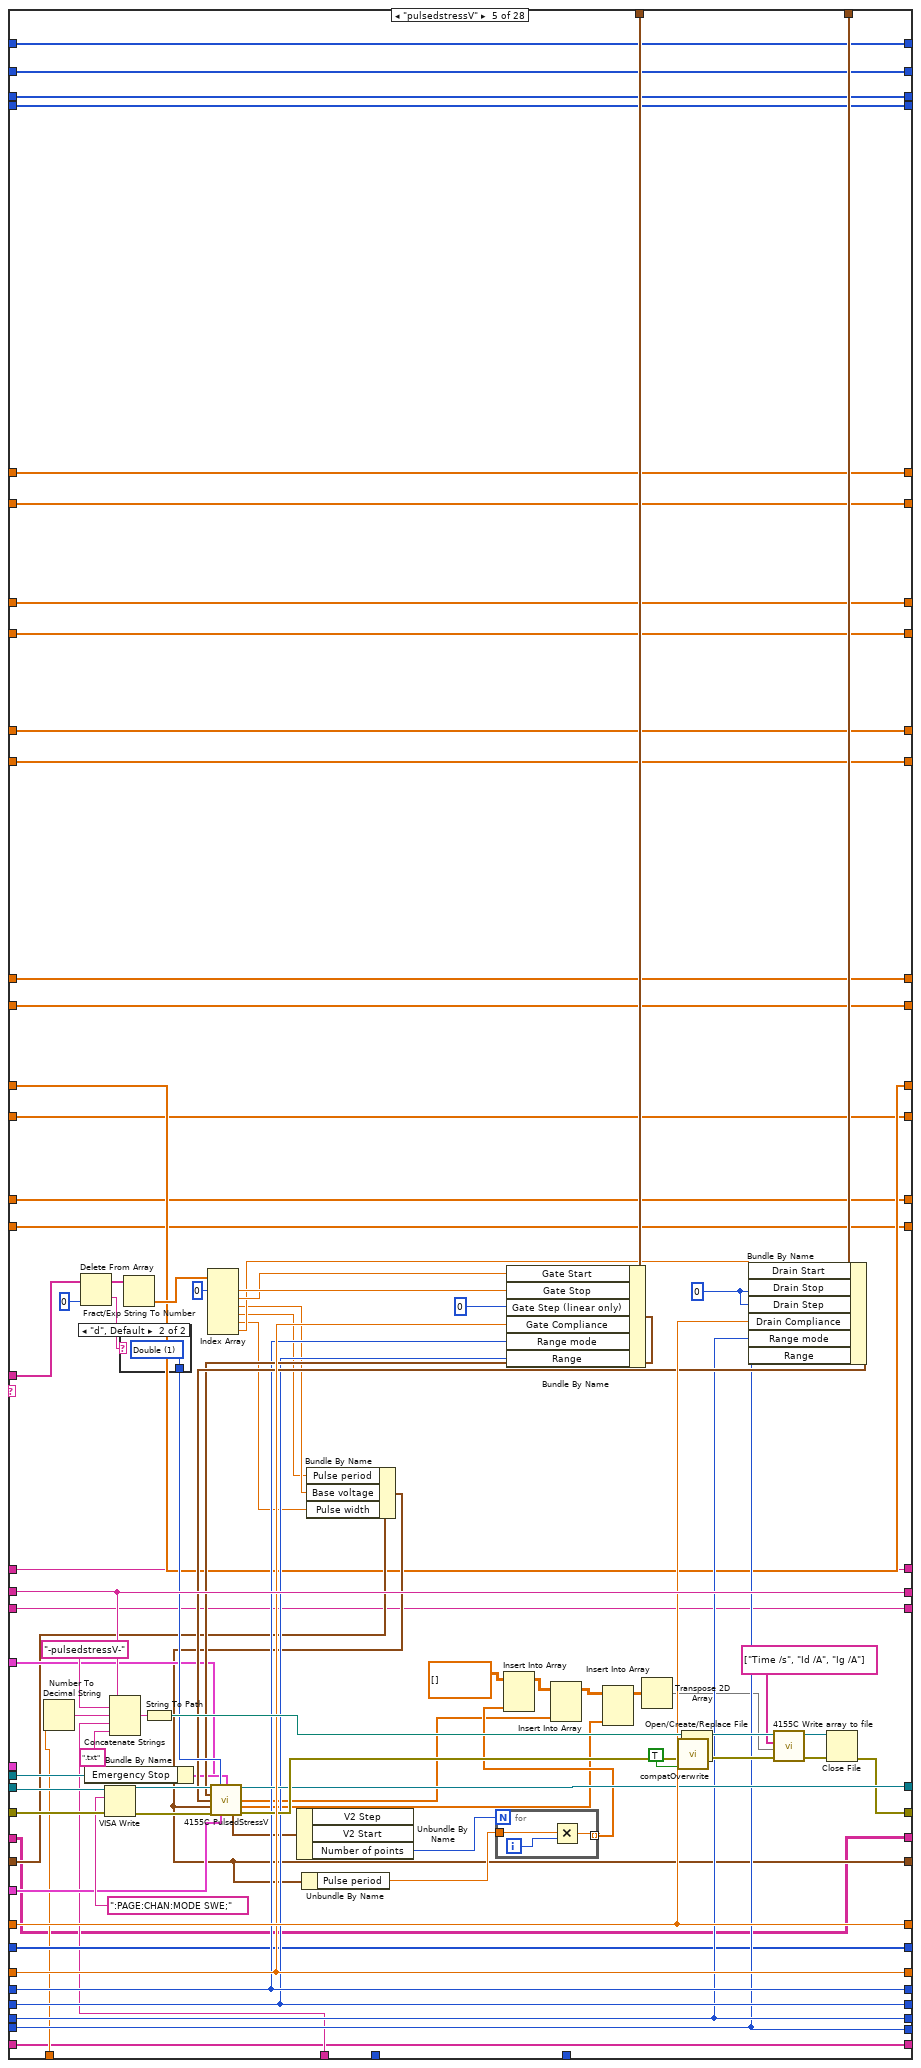
[diagram p10: hidden frame]
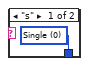
[diagram p11: hidden frame]
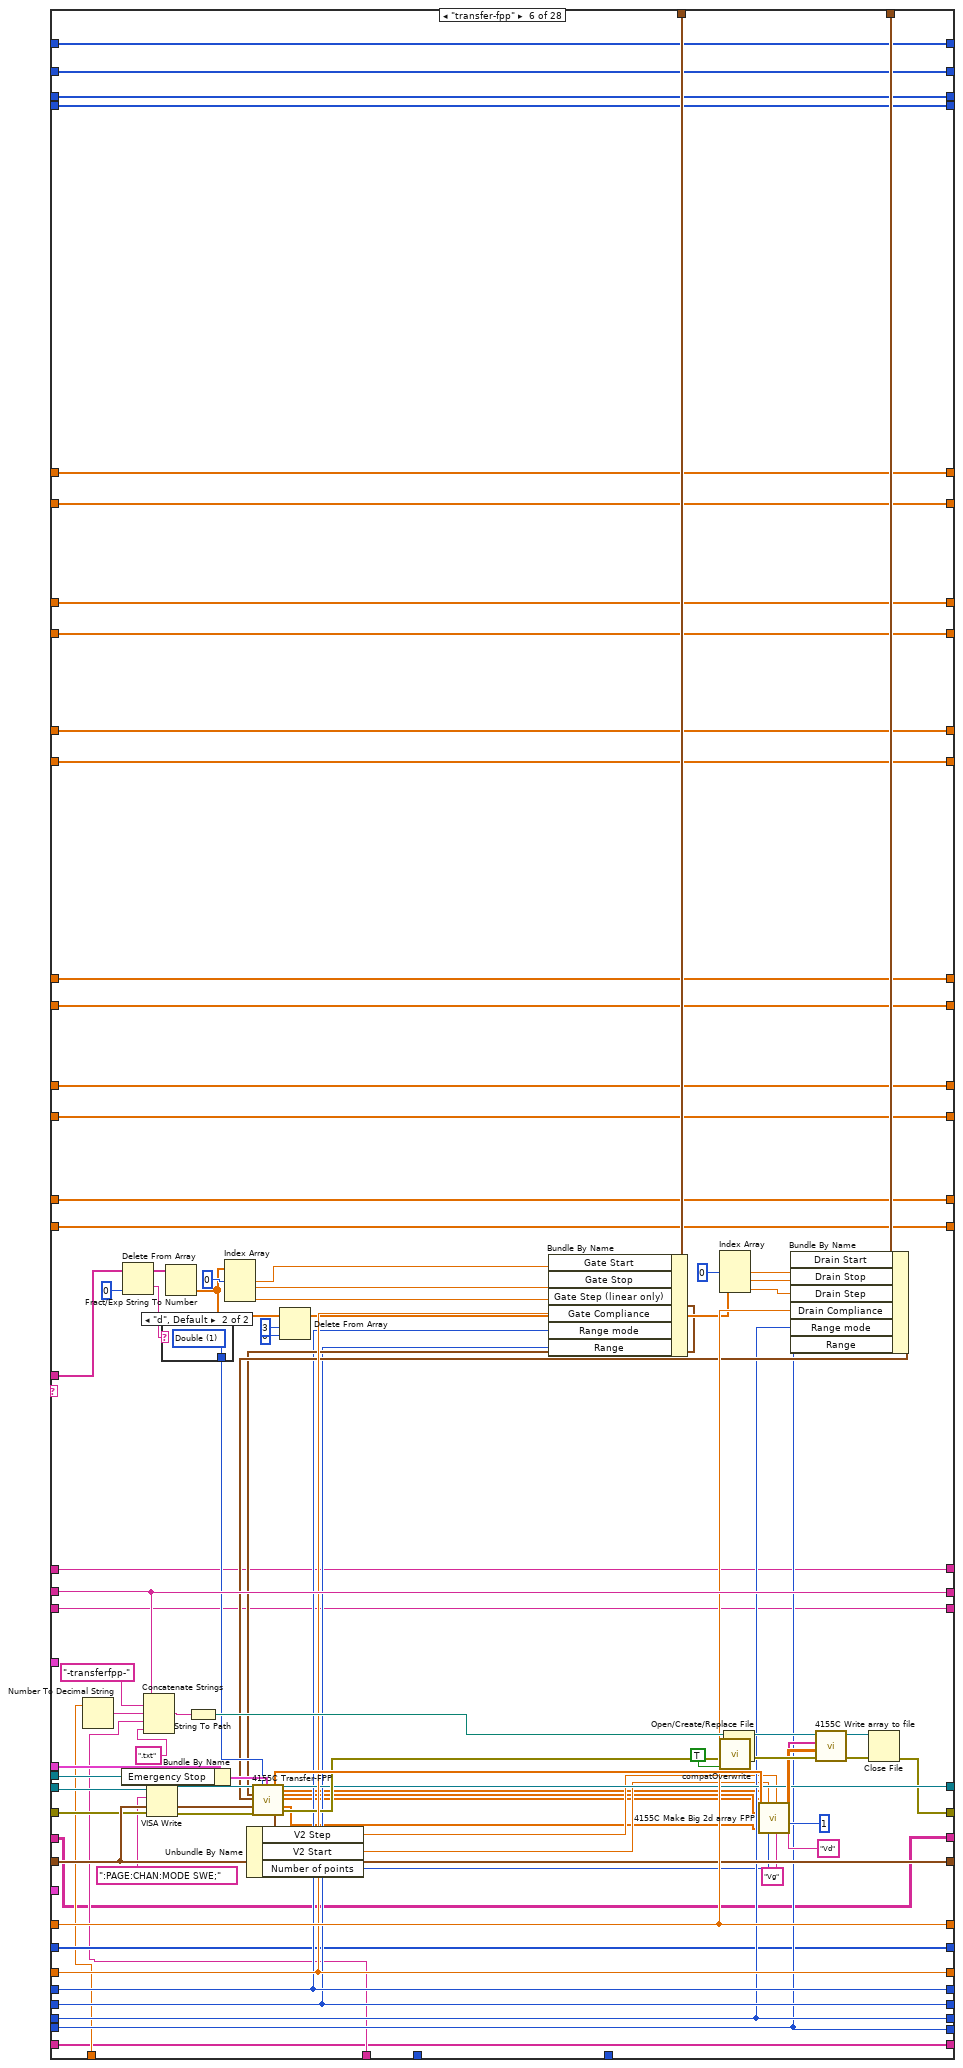
[diagram p12: hidden frame]
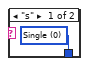
[diagram p13: hidden frame]
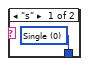
[diagram p14: hidden frame]
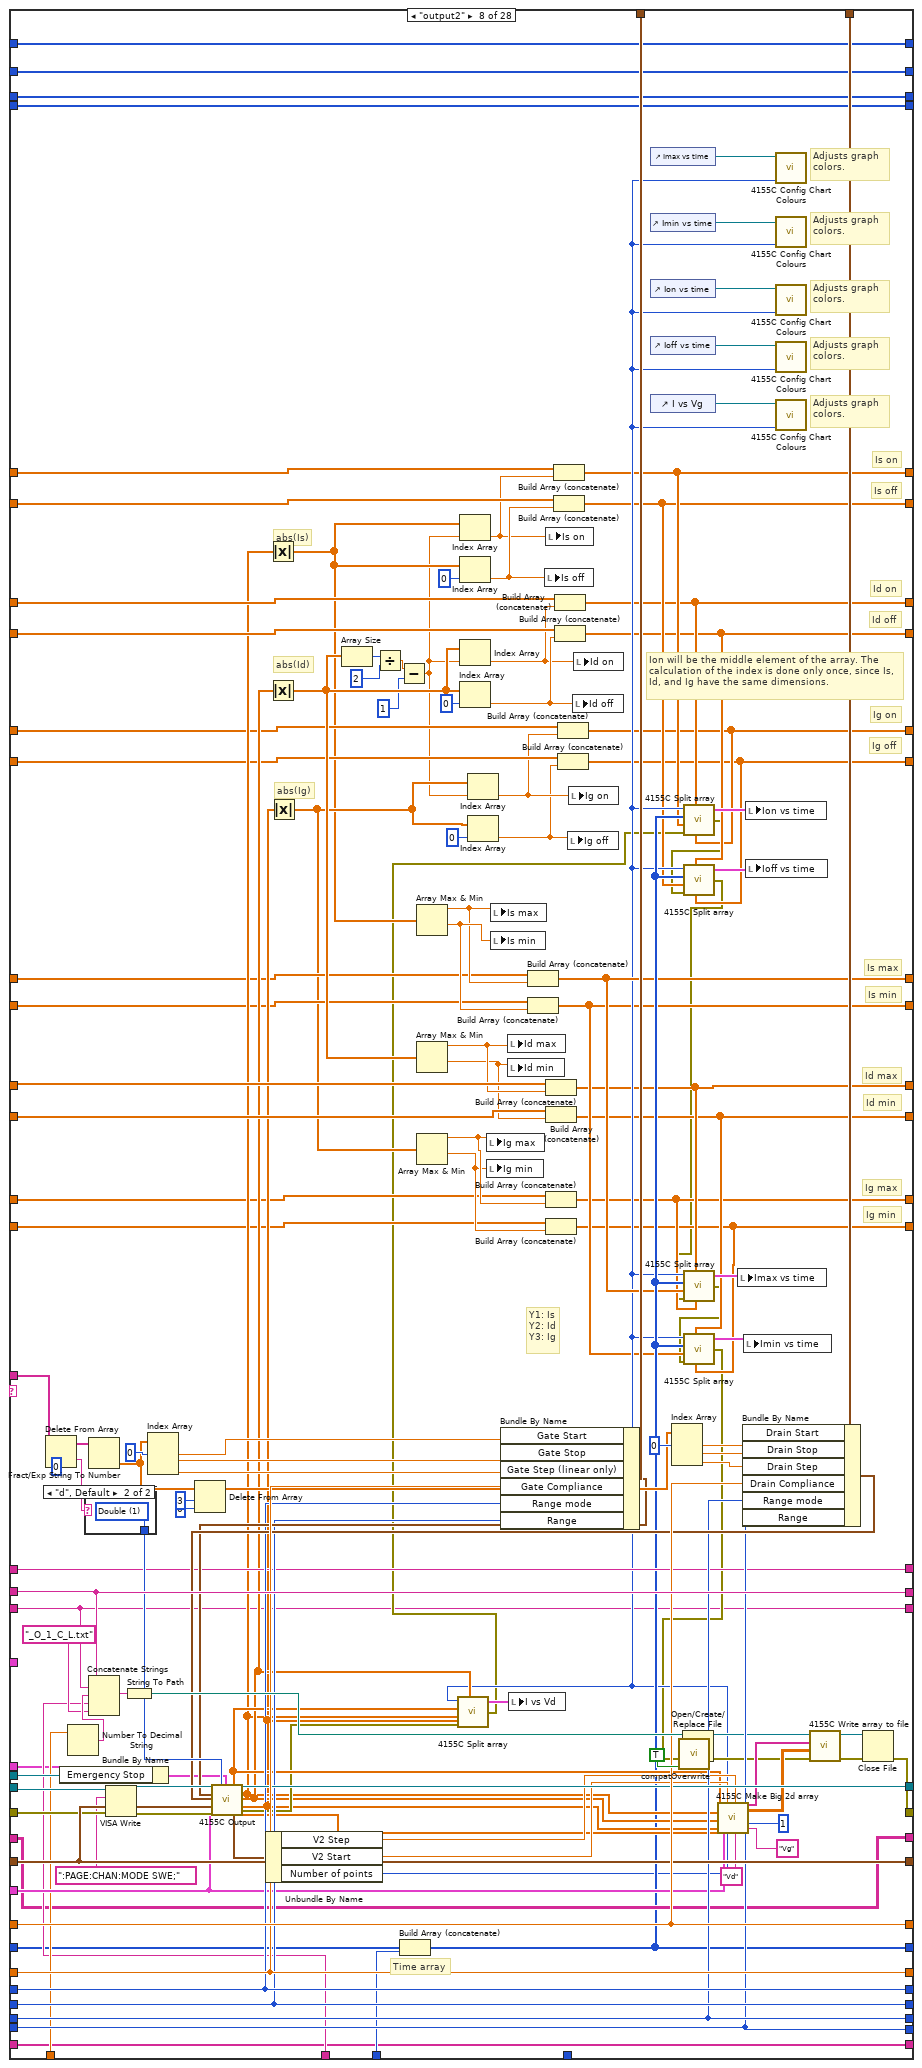
[diagram p15: hidden frame]
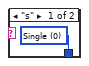
[diagram p16: hidden frame]
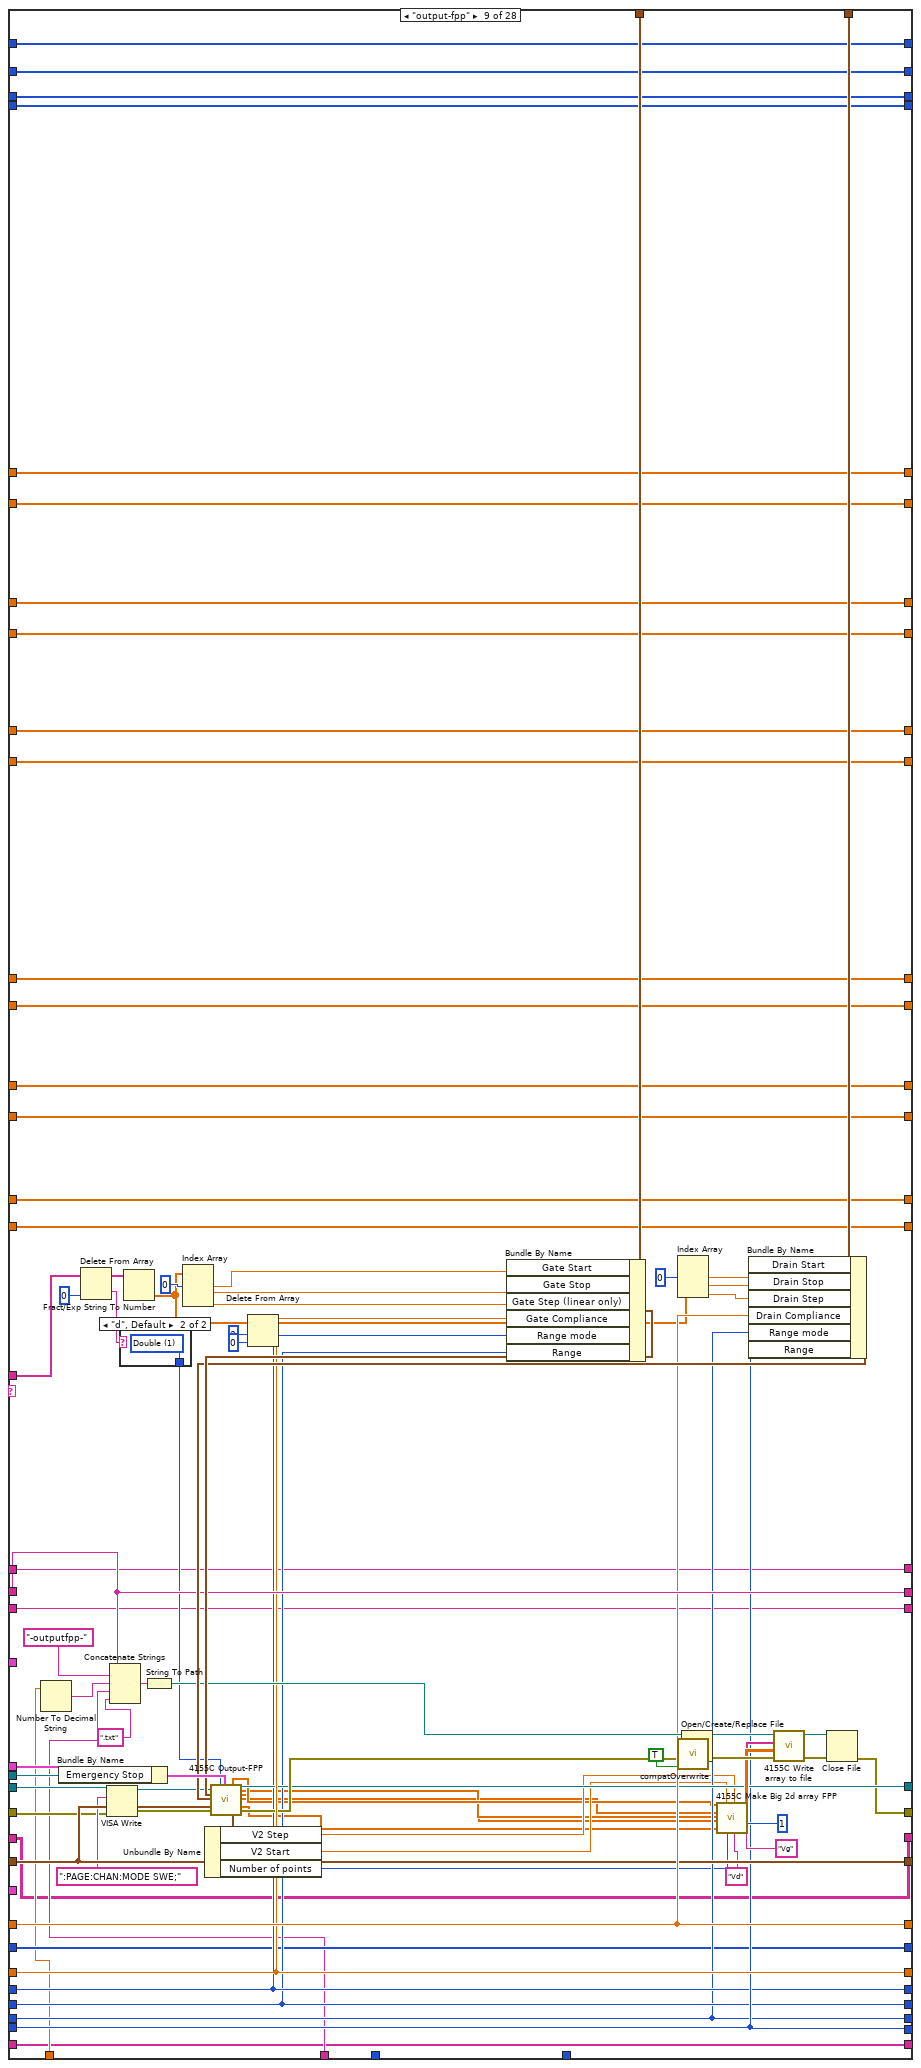
[diagram p17: hidden frame]
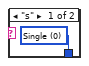
[diagram p18: hidden frame]
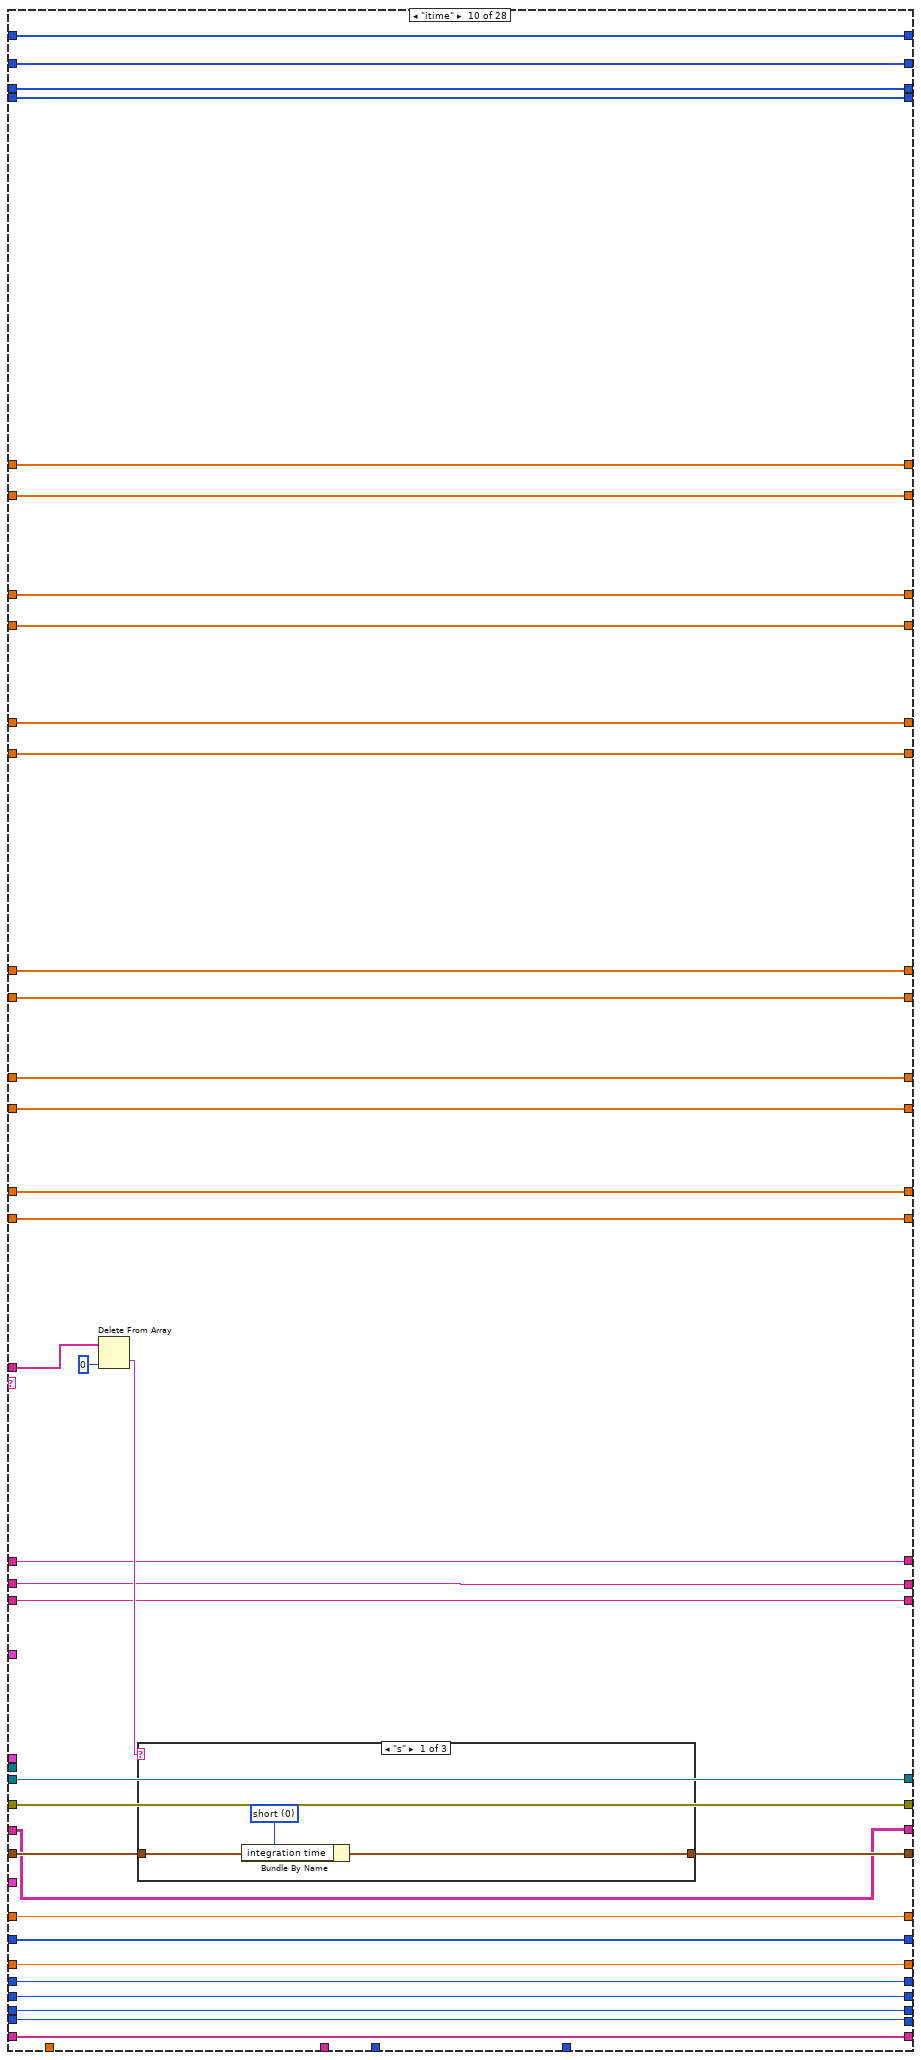
[diagram p19: hidden frame]
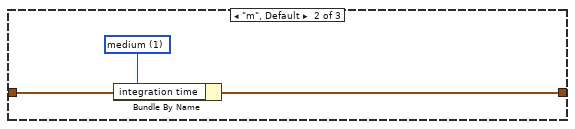
[diagram p20: hidden frame]
diagram:
  w49 = u16 1 items=["Reset All", "Partial reset"] ("Type of reset")
  # "Change from previous version:\n\n- Output curves are taken into account in Imax-Imin-Ion-Ioff plots."
  # "This is a version specific to the SPM pump."
  # "I add 1 to both the \"total lines\" and the \"line running\" indicators because i and N begin from 0, and the script lines begin from 1."
  # "Bugs:\n\n- If using the \"filename\" command, keep in mind that the arrays of the time-dependent data are not re-initialized inbetween filename changes. \n\n- Do not connect the \"error\" wire of a Split block if it has unconnected terminals! It will halt the program."
  # "Array size"
  # "%s option converts a spreadsheet string to an array of strings."
  # "0: No of rows of array\n1: No of cols"
  # "Dimitrios Simatos\nv. 5.5"
  # "Changes from original textcontrol.vi:\n\n- Timestamp appears in filename.\n- (Only) transfer and output curves are plotted.\n- Communication with serial port.\n- Can execute any command, as all pattern matching functions were replaced. Previously, commands with special LabVIEW characters could not be executed.\n- Replaced write to file function with write to text file.\n- Replaced while loop with for loop.\n- Replaced 4155C \"Save File\" function and now the vi can save time-dependent variables.\n- Added clock with start time control and various units.\n- Changed filepath in which the program is saved.\n- Added a serial output log that keeps a history.\n- Tab control.\n- Addition of specialized serial read/write file for the SPM OEM pump.\n- Added halt and hard stop.\n- Imax, Imin, Ion, and Ioff are now saved for all Is, Id, and Ig."
  # "Search and replace LF with EOL"
  n1 = Equal?(x="integration time", y=u32 0) -> (x = y?=w53:bool)
  n2 = Select(t="Integration time (short)", s=w53, f="Integration time (long)") -> (s? t:f=w57:dbl)
  n3 = call "4155C Get Filename.vi"("error in (no error)"=errorcluster {"status"=FALSE, "code"=0, "source"=""}) -> ("error out"=w44:errorcluster, "path"=w19:path)  [unwired: 2 in, 1 out]
  "Path" <- w19
  n4 = Bundle By Name(cluster="Timings 2", "integration time"="integration time", "Short/Long integration time"=w57, "hold time (sec)"="hold time /s", "delay time (sec)"="delay time /s", "Step Time (0 disables)"="Step delay /s") -> (w42:T6)
  n5 = Path To String(path=w19) -> (string=w20:string)
  n6 = Search and Replace String(replace all?=TRUE ("replace all? (F)"), input string="Script", search string="\n", replace string="\r\n") -> (result string=w32:string)  [unwired: 4 in, 3 out]
  n7 = Match Pattern(string=w20, regular expression=".txt") -> (before substring=w15:string)  [unwired: 1 in, 3 out]
  n8 = Concatenate Strings(w15, "Suffix (script)") -> (w14:string)
  n9 = call "4155C Initialise.vi"("VISA resource name in"=refnum<visa-resource-name> "GPIB0::14::INSTR", "Reset"="Full Reset", "Type of reset"=w49, "error in (no error)"=w44, "VISA Timeout Value"=u32 10000) -> ("VISA Resource Name out"=w43:refnum<visa-resource-name>, "error out"=w12:errorcluster)
  n10 = Spreadsheet String To Array(delimiter (Tab)="\r\n", format string="%s", spreadsheet string="Script", array type (2D Dbl)="") -> (array=w23:string[][])
  n11 = Array Size(array=w23) -> (size(s)=w27:i32[])
  n12 = Initialize Array("") -> (w4:string[])  [unwired: 1 in]
  n13 = String To Path(string=w14) -> (path=w13:path)
  n14 = Initialize Array(0 ("element")) -> (w6:i32[])  [unwired: 1 in]
  n15 = Initialize Array("") -> (w2:string[][])  [unwired: 2 in]
  n16 = Initialize Array(0.0 ("element")) -> (w8:dbl[])  [unwired: 1 in]
  n17 = Index Array(array=w27, index=0) -> (element=w25:i32)
  n18 = Write to Text File(file (use dialog)=w13, text=w32, error in=w12) -> (error out=w11:errorcluster)  [unwired: 1 in, 2 out]
  n19 = for {
    N: w25 -> [w167]
    tunnel: "SMU4" -> [w203]
    shift-left: "Source/Drain Range" -> [w208]
    shift-right: [w204] -> _
    shift-left: "Source/Drain\nRange mode" -> [w209]
    shift-right: [w205] -> _
    shift-left: "Gate Range" -> [w210]
    shift-right: [w206] -> _
    shift-left: "Gate Range\nmode" -> [w211]
    shift-right: [w207] -> _
    shift-left: "Gate: Compliance" -> [w220]
    shift-right: [w216] -> _
    shift-left: "Drain: Compliance" -> [w221]
    shift-right: [w217] -> _
    shift-left: w42 -> [w222]
    shift-right: [w218] -> _
    shift-left: w11 -> [w223]
    shift-right: [w113] -> w18
    shift-left: w43 -> [w224]
    shift-right: [w219] -> _
    shift-left: w15 -> [w225]
    shift-right: [w117] -> _
    tunnel: "Panel Controls 2" -> [w202]
    shift-right: [w75] -> _
    shift-left: w8 -> [w201]
    shift-right: [w137] -> _
    shift-left: _ -> [w197]
    tunnel: w23 -> [w196] mode=indexing
    shift-right: [w74] -> _
    shift-left: w8 -> [w173]
    shift-right: [w107] -> _
    shift-left: w4 -> [w159]
    shift-right: [w138] -> _
    shift-left: w6 -> [w154]
    shift-right: [w119] -> _
    shift-left: w6 -> [w153]
    shift-right: [w152] -> _
    shift-left: "" -> [w151]
    shift-right: [w112] -> _
    shift-left: w6 -> [w134]
    shift-right: [w111] -> _
    shift-left: w6 -> [w118]
    shift-right: [w108] -> _
    shift-left: w2 -> [w110]
    shift-right: [w68] -> _
    shift-left: w8 -> [w96]
    shift-right: [w69] -> _
    shift-left: w8 -> [w95]
    shift-right: [w73] -> _
    shift-left: w8 -> [w84]
    shift-right: [w72] -> _
    shift-left: w8 -> [w83]
    shift-right: [w66] -> _
    shift-left: w8 -> [w82]
    shift-right: [w76] -> _
    shift-left: w8 -> [w81]
    shift-right: [w67] -> _
    shift-left: w8 -> [w80]
    shift-right: [w65] -> _
    shift-left: w8 -> [w79]
    shift-right: [w71] -> _
    shift-left: w8 -> [w78]
    shift-right: [w70] -> _
    shift-left: w8 -> [w77]
    shift-right: [w60] -> _
    shift-left: "Filename (variable part)" -> [w59]
    i -> [w162]
    w98 = "Time (Minutes)" ("element")
    # "Filename prefix"
    # "Is off"
    # "Is on"
    # "Ig off"
    # "Ig on"
    # "Is min"
    # "Is max"
    # "Ig min"
    # "Ig max"
    # "Id min"
    # "Id max"
    # "Id off"
    # "Id on"
    # "Pump status"
    # "Filepath and name"
    # "Pump status"
    # "Limit of command arguments (array columns). Raise if needed."
    # "Serial port data (string)"
    # "Serial port data (table)"
    # "Time array for valve position"
    # "Time array for absolute plunger position"
    # "Valve position"
    # "Absolute plunger position"
    # "Serial port data"
    # "For loop counter"
    # "<-----Equivalent to the 4155C \"Write\" subvi.----->"
    # "Headers"
    # "Save transfer curves in file."
    # "Filepath and name"
    # "Save time-dependent data."
    # "Use the time offset if your measurements do not start at t=0."
    # "Time for Imax, Imin, Ion, Ioff"
    # "Rest of elements of command"
    # "First element of command\n(case select)"
    n20 = Add(x=w162, y=1) -> (x+y=→"Line running":i32)
    n21 = Add(x=w167, y=1) -> (x+y=→"Total lines":i32)
    n22 = Index Array(array=w196, index=0 ("line index")) -> (element=w191:string)
    "Command running:" <- w191
    n23 = control-ref of="Interrupt run"() -> (w215:refnum<vi>)
    n24 = Spreadsheet String To Array(delimiter (Tab)=" ", format string="%s", spreadsheet string=w191, array type (2D Dbl)=string[] []) -> (array=w189:string[])
    n25 = Delete From Array(array=w189, index=0) -> (deleted portion=w97:string, array with subset deleted=w188:string[])  [unwired: 1 in]
    n26 = call "Elapsed Time"("Reset"="Reset", "Auto Reset"="Auto Reset") -> ("Elapsed Time (s)"=w198:dbl)  [unwired: 10 in, 7 out]
    n27 = case shown="0, Default" "Units" {
      tunnel: ["_sec" "_min" "_h"] -> w199
      tunnel: [w226 w230 w233] -> w169
      tunnel: w198 -> [w226 w229 w234]
      frame 0, Default {
      }
      frame 1 {
        n28 = Divide(x=w229, y=60.0) -> (x/y=w230:dbl)
      }
      frame 2 {
        n29 = Divide(x=w234, y=3600.0) -> (x/y=w233:dbl)
      }
    }
    n30 = Add(x=w169, y="Time Offset") -> (x+y=w168:dbl)
    n31 = To Long Integer(number=w168) -> (32bit integer=w135:i32)
    "Elapsed Time" <- w135
    n32 = case shown="\"output\"" w97 {
      tunnel: w188 -> [w271 w309 w346 w478 w502 w648 w742 w894 w972 w1029 w1074 w1120 w1164 w1204 w1237 _ _ w1398 w1478 _ w1581 w1644 w1705 w1794 w1875 w1914 w1984 w2038]
      tunnel: w225 -> [w266 w305 w344 w485 w567 w656 w749 w901 w980 w1018 w1063 w1112 w1157 w1198 w1230 w1268 w1329 w1376 w1460 w1510 w1568 w1631 w1693 w1788 w1871 w1916 w1986 w2040]
      tunnel: w224 -> [w265 w304 w335 w456 w552 w625 w718 w872 w948 w1019 w1064 w1113 w1158 w1199 w1231 w1273 w1331 w1404 w1484 w1514 w1587 w1650 w1711 w1800 w1829 w1920 w1990 w2042]
      tunnel: w223 -> [w264 w303 w334 w455 w551 w624 w715 w871 w945 w1020 w1065 w1114 w1159 w1200 w1232 w1272 w1302 w1403 w1483 w1513 w1586 w1649 w1710 w1799 w1828 w1919 w1989 w2043]
      tunnel: w222 -> [w263 w302 w343 w481 w527 w652 w745 w897 w976 w1028 w1073 w1111 w1156 w1197 w1229 w1271 w1326 w1367 w1452 w1519 w1561 w1624 w1686 w1787 w1870 w1921 w1991 w2045]
      tunnel: w221 -> [w262 w301 w342 w483 w565 w654 w747 w899 w978 w1027 w1072 w1119 w1163 w1203 w1236 w1270 w1311 w1402 w1482 w1522 w1585 w1648 w1709 w1798 w1879 w1922 w1992 w2046]
      tunnel: w220 -> [w261 w300 w341 w482 w564 w653 w746 w898 w977 w1026 w1071 w1118 w1162 w1202 w1235 w1269 w1312 w1377 w1461 w1521 w1569 w1632 w1694 w1789 w1872 w1924 w1993 w2048]
      tunnel: [w265 w304 w333 w480 w562 w650 w744 w896 w974 w1019 w1064 w1113 w1158 w1199 w1231 w1273 w1331 w1368 w1434 w1512 w1562 w1625 w1687 w1740 w1831 w1920 w1990 w2042] -> w219
      tunnel: [w264 w303 w332 w479 w561 w649 w743 w895 w973 w1020 w1065 w1114 w1159 w1200 w1232 w1272 w1301 w1378 w1435 w1511 w1570 w1633 w1695 w1739 w1830 w1918 w1988 w2043] -> w133
      tunnel: [w263 w302 w343 w481 w523 w652 w745 w897 w976 w1021 w1066 w1111 w1156 w1197 w1229 w1271 w1326 w1367 w1452 w1519 w1561 w1624 w1686 w1787 w1870 w1921 w1991 w2045] -> w218
      tunnel: [w262 w301 w342 w483 w565 w654 w747 w899 w978 w1027 w1072 w1119 w1163 w1203 w1236 w1270 w1311 w1402 w1482 w1522 w1585 w1648 w1709 w1798 w1879 w1922 w1992 w2046] -> w217
      tunnel: [w261 w300 w341 w482 w564 w653 w746 w898 w977 w1026 w1071 w1118 w1162 w1202 w1235 w1269 w1312 w1377 w1461 w1521 w1569 w1632 w1694 w1789 w1872 w1924 w1993 w2048] -> w216
      tunnel: [w266 w305 w344 w485 w567 w656 w749 w901 w980 w1018 w1063 w1112 w1157 w1198 w1230 w1268 w1329 w1376 w1460 w1510 w1568 w1631 w1693 w1788 w1871 w1916 w1986 w2040] -> w117
      tunnel: w215 -> [_ _ _ w487 w571 w661 w752 w903 w984 _ _ _ _ _ _ _ _ w1373 w1457 _ w1567 w1630 w1692 w1760 w1847 _ _ _]
      tunnel: "Gate" -> [_ _ _ w465 w555 w635 w729 w881 w959 _ _ _ _ _ _ _ _ _ _ _ _ _ _ _ _ _ _ _]
      tunnel: "Drain 2" -> [_ _ _ w464 w554 w634 w728 w880 w958 _ _ _ _ _ _ _ _ _ _ _ _ _ _ _ _ _ _ _]
      tunnel: "Panel Controls" -> [_ _ _ _ _ w633 w727 w765 w957 _ _ _ _ _ _ _ _ _ _ _ _ _ _ _ _ _ _ _]
      tunnel: w211 -> [w260 w299 w340 w449 w545 w618 w713 w865 w943 w1025 w1070 _ w1155 w1196 w1228 w1267 w1313 w1363 w1448 w1515 w1557 w1620 w1682 w1783 w1866 w1925 w1994 w2049]
      tunnel: w210 -> [w259 w298 w339 w448 w544 w617 w712 w864 w942 w1024 w1069 w1117 _ w1187 w1234 w1266 w1314 w1364 w1449 w1516 w1558 w1621 w1683 w1784 w1867 w1926 w1995 w2050]
      tunnel: w209 -> [w258 w297 w338 w447 w543 w616 w711 w863 w941 w1023 w1068 w1116 w1161 w1201 _ w1265 w1315 w1365 w1450 w1517 w1559 w1622 w1684 w1785 w1868 w1927 w1996 w2051]
      tunnel: w208 -> [w257 w296 w337 w446 w542 w615 w714 w862 w944 w1022 w1067 w1115 w1160 _ w1233 w1264 w1316 w1366 w1451 w1518 w1560 w1623 w1685 w1786 w1869 w1928 w1997 w2052]
      tunnel: [w260 w299 w340 w449 w545 w618 w713 w865 w943 w1025 w1070 w1110 w1155 w1196 w1228 w1267 w1313 w1363 w1448 w1515 w1557 w1620 w1682 w1783 w1866 w1925 w1994 w2049] -> w207
      tunnel: [w259 w298 w339 w448 w544 w617 w712 w864 w942 w1024 w1069 w1117 w1147 w1187 w1234 w1266 w1314 w1364 w1449 w1516 w1558 w1621 w1683 w1784 w1867 w1926 w1995 w2050] -> w206
      tunnel: [w258 w297 w338 w447 w543 w616 w711 w863 w941 w1023 w1068 w1116 w1161 w1201 w1227 w1265 w1315 w1365 w1450 w1517 w1559 w1622 w1684 w1785 w1868 w1927 w1996 w2051] -> w205
      tunnel: [w257 w296 w337 w446 w542 w615 w714 w862 w944 w1022 w1067 w1115 w1160 w1188 w1233 w1264 w1316 w1366 w1451 w1518 w1560 w1623 w1685 w1786 w1869 w1928 w1997 w2052] -> w204
      tunnel: w203 -> [_ _ _ w441 w539 _ w707 w857 _ _ _ _ _ _ _ _ _ _ _ _ _ _ _ _ _ _ _ _]
      tunnel: w202 -> [_ _ _ w439 w538 _ _ _ _ _ _ _ _ _ _ _ _ _ _ _ _ _ _ _ _ _ _ _]
      tunnel: [w256 w292 w330 w367 w515 w605 w704 w784 w930 w1017 w1061 w1109 w1146 w1186 w1226 w1263 w1297 w1355 w1413 w1509 w1546 w1613 w1676 w1737 w1824 w1917 w1987 w2057] -> w75
      tunnel: w201 -> [w256 w292 w330 w436 w515 w605 w704 w853 w930 w1017 w1061 w1109 w1146 w1186 w1226 w1263 w1297 w1355 w1413 w1509 w1546 w1613 w1676 w1737 w1824 w1917 w1987 w2057]
      tunnel: w168 -> [_ _ _ w433 w512 w603 w701 w850 w927 _ _ _ _ _ _ _ w1295 w1353 w1430 _ w1543 w1610 w1673 w1734 w1820 _ _ _]
      tunnel: w199 -> [_ _ _ w430 w511 w601 w700 w847 w926 _ _ _ _ _ _ _ w1293 w1351 w1429 _ w1542 w1609 w1672 w1733 w1821 _ w1955 _]
      tunnel: w135 -> [_ _ _ w425 _ _ _ w842 _ _ _ _ _ _ _ _ _ _ _ _ _ _ _ _ _ _ w1958 _]
      tunnel: [w255 w291 w329 w375 w514 w604 w703 w792 w929 w1016 w1060 w1108 w1145 w1185 w1225 w1262 w1296 w1354 w1432 w1508 w1545 w1612 w1675 w1736 w1823 w1923 w1967 w2047] -> w137
      tunnel: w197 -> [w255 w291 w329 w429 w514 w604 w703 w846 w929 w1016 w1060 w1108 w1145 w1185 w1225 w1262 w1296 w1354 w1432 w1508 w1545 w1612 w1675 w1736 w1823 w1923 w1967 w2047]
      tunnel: [w254 w290 w328 w366 w510 w600 w699 w783 w925 w1015 w1059 w1107 w1144 w1184 w1224 w1261 w1292 w1350 w1412 w1507 w1541 w1608 w1671 w1732 w1819 w1912 w1983 w2056] -> w74
      tunnel: w173 -> [w254 w290 w328 w423 w510 w600 w699 w840 w925 w1015 w1059 w1107 w1144 w1184 w1224 w1261 w1292 w1350 w1412 w1507 w1541 w1608 w1671 w1732 w1819 w1912 w1983 w2056]
      tunnel: [w253 w289 w327 w416 w509 w599 w689 w833 w924 w1014 w1058 w1106 w1143 w1183 w1223 w1260 w1291 w1349 w1428 w1506 w1540 w1607 w1670 w1731 w1818 w1911 w1982 w2053] -> w107
      tunnel: w159 -> [w253 w289 w327 w416 w509 w599 w689 w833 w924 w1014 w1058 w1106 w1143 w1183 w1223 w1260 w1291 w1349 w1428 w1506 w1540 w1607 w1670 w1731 w1818 w1910 w1956 w2053]
      tunnel: [w252 w288 w326 w415 w508 w598 w688 w832 w923 w1013 w1057 w1105 w1142 w1182 w1222 w1259 w1290 w1348 w1427 w1505 w1539 w1606 w1669 w1730 w1817 w1896 w1969 w2067] -> w138
      tunnel: w154 -> [w252 w288 w326 w415 w508 w598 w688 w832 w923 w1013 w1057 w1105 w1142 w1182 w1222 w1259 w1290 w1348 w1427 w1505 w1539 w1606 w1669 w1730 w1817 w1896 w1968 w2067]
      tunnel: [w251 w287 w325 w414 w507 w597 w687 w831 w922 w1012 w1056 w1104 w1141 w1181 w1221 w1258 w1289 w1347 w1426 w1504 w1538 w1605 w1668 w1729 w1816 w1895 w1951 w2069] -> w119
      tunnel: w153 -> [w251 w287 w325 w414 w507 w597 w687 w831 w922 w1012 w1056 w1104 w1141 w1181 w1221 w1258 w1289 w1347 w1426 w1504 w1538 w1605 w1668 w1729 w1816 w1895 w1949 w2069]
      tunnel: [w250 w286 w324 w413 w506 w596 w686 w830 w921 w1011 w1055 w1103 w1140 w1180 w1220 w1257 w1288 w1346 w1425 w1503 w1537 w1604 w1667 w1728 w1815 w1894 w1948 w2041] -> w152
      tunnel: w151 -> [w250 w286 w324 w413 w506 w596 w686 w830 w921 w1011 w1055 w1103 w1140 w1180 w1220 w1257 w1288 w1346 w1425 w1503 w1537 w1604 w1667 w1728 w1815 w1894 w1959 w2041]
      tunnel: w135 -> [_ _ _ _ _ _ _ _ _ _ _ _ _ _ _ _ _ _ _ _ _ _ _ _ _ _ w1947 _]
      tunnel: w134 -> [w249 w285 w323 w412 w505 w595 w685 w829 w920 w1010 w1054 w1102 w1139 w1179 w1219 w1256 w1287 w1345 w1424 w1502 w1536 w1603 w1666 w1727 w1814 w1893 w1946 w2068]
      tunnel: [w249 w285 w323 w412 w505 w595 w685 w829 w920 w1010 w1054 w1102 w1139 w1179 w1219 w1256 w1287 w1345 w1424 w1502 w1536 w1603 w1666 w1727 w1814 w1893 w1945 w2068] -> w112
      tunnel: [w248 w284 w322 w411 w504 w594 w684 w828 w919 w1009 w1053 w1101 w1138 w1178 w1218 w1255 w1286 w1344 w1423 w1501 w1535 w1602 w1665 w1726 w1813 w1892 w1944 w2066] -> w111
      tunnel: w118 -> [w248 w284 w322 w411 w504 w594 w684 w828 w919 w1009 w1053 w1101 w1138 w1178 w1218 w1255 w1286 w1344 w1423 w1501 w1535 w1602 w1665 w1726 w1813 w1892 w1943 w2066]
      tunnel: [w247 w283 w321 w410 w503 w593 w683 w827 w918 w1008 w1052 w1100 w1137 w1177 w1217 w1254 w1285 w1343 w1422 w1500 w1534 w1601 w1664 w1725 w1812 w1891 w1941 w2044] -> w108
      tunnel: w110 -> [w247 w283 w321 w410 w503 w593 w683 w827 w918 w1008 w1052 w1100 w1137 w1177 w1217 w1254 w1285 w1343 w1422 w1500 w1534 w1601 w1664 w1725 w1812 w1891 w1940 w2044]
      tunnel: [w245 w281 w319 w360 w500 w591 w681 w777 w916 w1006 w1051 w1099 w1135 w1175 w1215 w1252 w1283 w1342 w1421 w1499 w1533 w1600 w1662 w1724 w1811 w1890 w1939 w2062] -> w68
      tunnel: w96 -> [w245 w281 w319 w406 w500 w591 w681 w823 w916 w1006 w1051 w1099 w1135 w1175 w1215 w1252 w1283 w1342 w1421 w1499 w1533 w1600 w1662 w1724 w1811 w1890 w1939 w2062]
      tunnel: [w246 w282 w320 w361 w501 w592 w682 w778 w917 w1007 w1050 w1098 w1136 w1176 w1216 w1253 w1284 w1341 w1420 w1498 w1532 w1599 w1663 w1723 w1810 w1889 w1938 w2063] -> w69
      tunnel: w95 -> [w246 w282 w320 w405 w501 w592 w682 w822 w917 w1007 w1050 w1098 w1136 w1176 w1216 w1253 w1284 w1341 w1420 w1498 w1532 w1599 w1663 w1723 w1810 w1889 w1938 w2063]
      tunnel: [w238 w274 w312 w365 w497 w589 w679 w782 w914 w999 w1048 w1096 w1133 w1173 w1213 w1250 w1276 w1334 w1411 w1497 w1525 w1592 w1655 w1716 w1805 w1882 w1937 w2055] -> w73
      tunnel: w84 -> [w238 w274 w312 w395 w497 w589 w679 w812 w914 w999 w1048 w1096 w1133 w1173 w1213 w1250 w1276 w1334 w1411 w1497 w1525 w1592 w1655 w1716 w1805 w1882 w1937 w2055]
      tunnel: [w237 w273 w311 w364 w498 w590 w680 w781 w915 w998 w1049 w1097 w1134 w1174 w1214 w1251 w1275 w1333 w1410 w1496 w1524 w1591 w1654 w1715 w1804 w1881 w1936 w2054] -> w72
      tunnel: w83 -> [w237 w273 w311 w394 w498 w590 w680 w811 w915 w998 w1049 w1097 w1134 w1174 w1214 w1251 w1275 w1333 w1410 w1496 w1524 w1591 w1654 w1715 w1804 w1881 w1936 w2054]
      tunnel: [w240 w276 w314 w370 w496 w587 w677 w787 w912 w1004 w1046 w1094 w1131 w1171 w1211 w1248 w1278 w1336 w1415 w1491 w1527 w1594 w1657 w1718 w1803 w1886 w1934 w2059] -> w66
      tunnel: w82 -> [w240 w276 w314 w391 w496 w587 w677 w808 w912 w1004 w1046 w1094 w1131 w1171 w1211 w1248 w1278 w1336 w1415 w1491 w1527 w1594 w1657 w1718 w1803 w1886 w1934 w2059]
      tunnel: [w239 w275 w313 w368 w499 w588 w678 w785 w913 w1005 w1047 w1095 w1132 w1172 w1212 w1249 w1277 w1335 w1414 w1490 w1526 w1593 w1656 w1717 w1802 w1885 w1935 w2058] -> w76
      tunnel: w81 -> [w239 w275 w313 w390 w499 w588 w678 w807 w913 w1005 w1047 w1095 w1132 w1172 w1212 w1249 w1277 w1335 w1414 w1490 w1526 w1593 w1656 w1717 w1802 w1885 w1935 w2058]
      tunnel: [w242 w278 w316 w359 w495 w585 w675 w776 w910 w1002 w1044 w1092 w1129 w1169 w1209 w1246 w1280 w1338 w1417 w1493 w1529 w1596 w1659 w1720 w1807 w1888 w1932 w2061] -> w67
      tunnel: w80 -> [w242 w278 w316 w387 w495 w585 w675 w804 w910 w1002 w1044 w1092 w1129 w1169 w1209 w1246 w1280 w1338 w1417 w1493 w1529 w1596 w1659 w1720 w1807 w1888 w1932 w2061]
      tunnel: [w241 w277 w315 w358 w494 w586 w676 w775 w911 w1003 w1045 w1093 w1130 w1170 w1210 w1247 w1279 w1337 w1416 w1492 w1528 w1595 w1658 w1719 w1806 w1887 w1933 w2060] -> w65
      tunnel: w79 -> [w241 w277 w315 w386 w494 w586 w676 w803 w911 w1003 w1045 w1093 w1130 w1170 w1210 w1247 w1279 w1337 w1416 w1492 w1528 w1595 w1658 w1719 w1806 w1887 w1933 w2060]
      tunnel: [w244 w280 w318 w363 w493 w583 w673 w780 w908 w1000 w1042 w1090 w1127 w1167 w1207 w1244 w1282 w1340 w1419 w1495 w1531 w1598 w1661 w1722 w1809 w1884 w1930 w2065] -> w71
      tunnel: w78 -> [w244 w280 w318 w383 w493 w583 w673 w800 w908 w1000 w1042 w1090 w1127 w1167 w1207 w1244 w1282 w1340 w1419 w1495 w1531 w1598 w1661 w1722 w1809 w1884 w1930 w2065]
      tunnel: [w243 w279 w317 w362 w492 w584 w674 w779 w909 w1001 w1043 w1091 w1128 w1168 w1208 w1245 w1281 w1339 w1418 w1494 w1530 w1597 w1660 w1721 w1808 w1883 w1931 w2064] -> w70
      tunnel: w77 -> [w243 w279 w317 w382 w492 w584 w674 w799 w909 w1001 w1043 w1091 w1128 w1168 w1208 w1245 w1281 w1339 w1418 w1494 w1530 w1597 w1660 w1721 w1808 w1883 w1931 w2064]
      tunnel: w59 -> [w236 w272 w310 w349 w491 w582 w672 w766 w907 w997 w1041 w1089 w1126 w1166 w1206 w1243 w1274 w1332 w1409 w1489 w1523 w1590 w1653 w1714 w1801 w1880 w1929 _]
      tunnel: [w236 w272 w310 w349 w491 w582 w672 w766 w907 w997 w1041 w1089 w1126 w1166 w1206 w1243 w1274 w1332 w1409 w1489 w1523 w1590 w1653 w1714 w1801 w1880 w1929 w2037] -> w60
      frame "wait" {
        n33 = Index Array(array=w271, index=0 ("Index")) -> (element=w269:string)
        n34 = Decimal String To Number(string=w269, default (0L)=u32 0) -> (number=w268:u32)  [unwired: 1 in, 1 out]
        n35 = Wait (ms)(milliseconds to wait=w268) -> ()  [unwired: 1 out]
      }
      frame "wait-min" {
        n36 = Index Array(array=w309, index=0 ("Index")) -> (element=w307:string)
        n37 = Decimal String To Number(string=w307, default (0L)=u32 0) -> (number=w295:u32)  [unwired: 1 in, 1 out]
        n38 = Multiply(x=w295, y=u32 60000) -> (x*y=w294:u32)
        n39 = Wait (ms)(milliseconds to wait=w294) -> ()  [unwired: 1 out]
      }
      frame "standby" {
        n40 = Index Array(array=w346, index=0 ("Index")) -> (element=w336:string)
        n41 = case shown="\"off\", Default" w336 {
          tunnel: [":PAGE:SCON:STAN 0" ":PAGE:SCON:STAN 1"] -> w331
          frame "off", Default {
          }
          frame "on" {
          }
        }
        n42 = VISA Write(VISA resource name=w335, write buffer=w331, error in (no error)=w334) -> (VISA resource name out=w333:refnum<visa-resource-name>, error out=w332:errorcluster)  [unwired: 1 out]
      }
      frame "transfer" {
        # "Adjusts graph colors."
        # "Adjusts graph colors."
        # "Is off"
        # "Is on"
        # "Ion will be the middle element of the array. The calculation of the index is done only once, since Is, Id, and Ig have the same dimensions."
        # "Ig off"
        # "Ig on"
        # "Is min"
        # "Is max"
        # "Ig min"
        # "Ig max"
        # "abs(Ig)"
        # "abs(Is)"
        # "Id min"
        # "Id max"
        # "Y1: Is\nY2: Id\nY3: Ig"
        # "abs(Id)"
        # "Adjusts graph colors."
        # "Adjusts graph colors."
        # "Id off"
        # "Id on"
        # "Adjusts graph colors."
        # "Time array"
        n43 = Delete From Array(array=w478, index=0 ("Index")) -> (deleted portion=w476:string, array with subset deleted=w475:string[])  [unwired: 1 in]
        n44 = Bundle By Name(cluster=w439, "Emergency Stop"=w487) -> (w440:T2)
        n45 = Number To Decimal String(number=w433) -> (decimal integer string=w432:string)  [unwired: 1 in]
        n46 = case shown="\"d\", Default" w476 {
          tunnel: [w489 w490] -> w474
          frame "s" {
            w489 = u16 0 items=["Single", "Double"] ("sweep mode")
          }
          frame "d", Default {
            w490 = u16 1 items=["Single", "Double"] ("sweep mode")
          }
        }
        n47 = Fract/Exp String To Number(string=w475) -> (number=w460:dbl[])  [unwired: 3 in, 1 out]
        n48 = Concatenate Strings(w485, w349, w432, w430, "_T_1_C_L.txt" ("Suffix (transfer)")) -> (w486:string)
        n49 = VISA Write(VISA resource name=w456, write buffer=":PAGE:CHAN:MODE SWE;" ("write buffer (\"\")"), error in (no error)=w455) -> (VISA resource name out=w453:refnum<visa-resource-name>, error out=w454:errorcluster)  [unwired: 1 out]
        n50 = String To Path(string=w486) -> (path=w484:path)
        n51 = Index Array(array=w460, index #1=0 ("Index")) -> (element #1=w473:dbl, element #2=w472:dbl, element #3=w471:dbl)  [unwired: 2 in]
        n52 = Delete From Array(array=w460, length=3 ("Length"), index=0 ("Index")) -> (array with subset deleted=w458:dbl[])  [unwired: 1 out]
        n53 = Build Array (concatenate)(w429, w425) -> (w375:i32[])
        n54 = Bundle By Name(cluster=w465, "Gate Start"=w473, "Gate Stop"=w472, "Gate Step (linear only)"=w471, "Gate Compliance"=w482, "Range mode"=w449, "Range"=w448) -> (w450:T4)
        n55 = control-ref of="Imax vs time"() -> (w404:refnum<vi>)
        n56 = control-ref of="Imin vs time"() -> (w403:refnum<vi>)
        n57 = control-ref of="Ion vs time"() -> (w372:refnum<vi>)
        n58 = control-ref of="Ioff vs time"() -> (w371:refnum<vi>)
        n59 = control-ref of="I vs Vg"() -> (w434:refnum<vi>)
        n60 = Index Array(array=w458, index #1=0 ("Index")) -> (element #1=w468:dbl, element #2=w467:dbl, element #3=w466:dbl)  [unwired: 2 in]
        n61 = call <vilib>:"compatOverwrite.vi"("overwrite (F)"=TRUE) -> ("overwrite?"=w438:T7)
        n62 = Bundle By Name(cluster=w464, "Drain Start"=w468, "Drain Stop"=w467, "Drain Step"=w466, "Drain Compliance"=w483, "Range mode"=w447, "Range"=w446) -> (w451:T5)
        n63 = call "4155C Transfer.vi"("VISA resource name in"=w453, "Gate"=w450, "Drain"=w451, "Timings"=w481, "error in (no error)"=w454, "SMU4"=w441, "sweep mode"=w474, "Panel Controls"=w440) -> ("VG"=w437:dbl[], "Outparams"=w445:T8, "VISA Resource Name out"=w480:refnum<visa-resource-name>, "IS"=w400:dbl[], "ID"=w402:dbl[], "IG"=w399:dbl[], "error out"=w426:errorcluster, "SMU4"=w442:dbl[])  [unwired: 12 in]
        n64 = Unbundle By Name(w445) -> ("V2 Step"=w444:dbl, "V2 Start"=w443:dbl, "Number of points"=w369:i32)
        n65 = Absolute Value(x=w400) -> (abs(x)=w385:dbl[])
        n66 = Absolute Value(x=w402) -> (abs(x)=w401:dbl[])
        n67 = Absolute Value(x=w399) -> (abs(x)=w388:dbl[])
        n68 = Array Size(array=w401) -> (size(s)=w409:i32)
        n69 = Divide(x=w409, y=2) -> (x/y=w352:dbl)
        n70 = Subtract(x=w352, y=1) -> (x-y=w351:dbl)
        n71 = Array Max & Min(array=w385) -> (max value=w392:dbl, min value=w393:dbl)  [unwired: 2 out]
        n72 = Array Max & Min(array=w401) -> (max value=w435:dbl, min value=w398:dbl)  [unwired: 2 out]
        n73 = Array Max & Min(array=w388) -> (max value=w397:dbl, min value=w396:dbl)  [unwired: 2 out]
        n74 = call "4155C Split array.vi"("Number of VAR2 steps"=w369, "Y2 data in"=w402, "X data in"=w437, "Y1 data in"=w400, "Y3 data in"=w399, "error in (no error)"=w426) -> ("Array of clusters"=w428:cluster{"Y data in":dbl[], "X data in":dbl[]}[], "error out"=w357:errorcluster)  [unwired: 1 in]
        n75 = Index Array(array=w385, index=w351) -> (element=w376:dbl)
        n76 = Index Array(array=w385, index=0) -> (element=w377:dbl)
        n77 = Index Array(array=w401, index=w351) -> (element=w378:dbl)
        n78 = Index Array(array=w401, index=0) -> (element=w379:dbl)
        n79 = Index Array(array=w388, index=w351) -> (element=w381:dbl)
        n80 = Index Array(array=w388, index=0) -> (element=w380:dbl)
        n81 = local write "Ig max"(w397) -> ()
        n82 = local write "Ig min"(w396) -> ()
        n83 = local write "Is max"(w392) -> ()
        n84 = local write "Is min"(w393) -> ()
        n85 = local write "Id max"(w435) -> ()
        n86 = local write "Id min"(w398) -> ()
        n87 = local write "I vs Vg"(w428) -> ()
        n88 = Build Array (concatenate)(w391, w392) -> (w370:dbl[])
        n89 = Build Array (concatenate)(w390, w393) -> (w368:dbl[])
        n90 = local write "Is off"(w377) -> ()
        n91 = local write "Is on"(w376) -> ()
        n92 = Build Array (concatenate)(w436, w435) -> (w367:dbl[])
        n93 = Build Array (concatenate)(w423, w398) -> (w366:dbl[])
        n94 = Build Array (concatenate)(w395, w397) -> (w365:dbl[])
        n95 = Build Array (concatenate)(w394, w396) -> (w364:dbl[])
        n96 = Build Array (concatenate)(w383, w376) -> (w363:dbl[])
        n97 = Build Array (concatenate)(w382, w377) -> (w362:dbl[])
        n98 = Build Array (concatenate)(w405, w378) -> (w361:dbl[])
        n99 = Build Array (concatenate)(w406, w379) -> (w360:dbl[])
        n100 = Build Array (concatenate)(w387, w381) -> (w359:dbl[])
        n101 = Build Array (concatenate)(w386, w380) -> (w358:dbl[])
        n102 = local write "Ig off"(w380) -> ()
        n103 = local write "Ig on"(w381) -> ()
        n104 = local write "Id off"(w379) -> ()
        n105 = local write "Id on"(w378) -> ()
        n106 = call "4155C Split array.vi"("Number of VAR2 steps"=w369, "Y2 data in"=w361, "X data in"=w375, "Y1 data in"=w363, "Y3 data in"=w359, "error in (no error)"=w357) -> ("Array of clusters"=w373:cluster{"Y data in":dbl[], "X data in":dbl[]}[], "error out"=w356:errorcluster)  [unwired: 1 in]
        n107 = call "4155C Split array.vi"("Number of VAR2 steps"=w369, "Y2 data in"=w360, "X data in"=w375, "Y1 data in"=w362, "Y3 data in"=w358, "error in (no error)"=w356) -> ("Array of clusters"=w374:cluster{"Y data in":dbl[], "X data in":dbl[]}[], "error out"=w355:errorcluster)  [unwired: 1 in]
        n108 = call "4155C Split array.vi"("Number of VAR2 steps"=w369, "Y2 data in"=w367, "X data in"=w375, "Y1 data in"=w370, "Y3 data in"=w365, "error in (no error)"=w355) -> ("Array of clusters"=w427:cluster{"Y data in":dbl[], "X data in":dbl[]}[], "error out"=w354:errorcluster)  [unwired: 1 in]
        n109 = call "4155C Split array.vi"("Number of VAR2 steps"=w369, "Y2 data in"=w366, "X data in"=w375, "Y1 data in"=w368, "Y3 data in"=w364, "error in (no error)"=w354) -> ("Array of clusters"=w424:cluster{"Y data in":dbl[], "X data in":dbl[]}[], "error out"=w353:errorcluster)  [unwired: 1 in]
        n110 = Open/Create/Replace File(file path (use dialog)=w484, error in=w353, operation (0:open)=w438) -> (refnum out=w421:refnum<file>, error out=w419:errorcluster)  [unwired: 3 in, 1 out]
        n111 = call "4155C Make Big 2d array.vi"("1D Var1"=w437, "1d IS"=w400, "1d ID"=w402, "1d IG"=w399, "1d SMU4"=w442, "SMU4"=w441, "VAR2 START"=w443, "Number of VAR2 steps"=w369, "VAR2 STEP"=w444, "VAR1 Name"="Vg", "Decimal places in header"=i8 1, "VAR2 Name"="Vd") -> ("Header array"=w422:string[], "Data array"=w420:dbl[][])  [unwired: 14 in]
        n112 = local write "Imax vs time"(w427) -> ()
        n113 = local write "Imin vs time"(w424) -> ()
        n114 = local write "Ion vs time"(w373) -> ()
        n115 = local write "Ioff vs time"(w374) -> ()
        n116 = call "4155C Config Chart Colours.vi"("Numeric"=w369, "XY Graph 2"=w404) -> ()  [unwired: 6 in]
        n117 = call "4155C Config Chart Colours.vi"("Numeric"=w369, "XY Graph 2"=w403) -> ()  [unwired: 6 in]
        n118 = call "4155C Config Chart Colours.vi"("Numeric"=w369, "XY Graph 2"=w372) -> ()  [unwired: 6 in]
        n119 = call "4155C Config Chart Colours.vi"("Numeric"=w369, "XY Graph 2"=w371) -> ()  [unwired: 6 in]
        n120 = call "4155C Config Chart Colours.vi"("Numeric"=w369, "XY Graph 2"=w434) -> ()  [unwired: 6 in]
        n121 = call "4155C Write array to file.vi"("Byte Stream File Refnum"=w421, "Header"=w422, "Data Array"=w420, "error in (no error)"=w419) -> ("dup refnum"=w418:refnum<file>, "error out"=w417:errorcluster)  [unwired: 1 in]
        n122 = Close File(refnum=w418, error in=w417) -> (error out=w479:errorcluster)  [unwired: 1 out]
      }
      frame "pulsedstressV" {
        w521 = 0
        n123 = Number To Decimal String(number=w512) -> (decimal integer string=w568:string)  [unwired: 1 in]
        n124 = Delete From Array(array=w502, index=0 ("Index")) -> (deleted portion=w559:string, array with subset deleted=w558:string[])  [unwired: 1 in]
        n125 = Bundle By Name(cluster=w538, "Emergency Stop"=w571) -> (w540:T2)
        n126 = VISA Write(VISA resource name=w552, write buffer=":PAGE:CHAN:MODE SWE;" ("write buffer (\"\")"), error in (no error)=w551) -> (VISA resource name out=w549:refnum<visa-resource-name>, error out=w550:errorcluster)  [unwired: 1 out]
        n127 = Concatenate Strings(w567, "-pulsedstressV-" ("Substring"), w568, w511, ".txt" ("Substring")) -> (w570:string)
        n128 = case shown="\"d\", Default" w559 {
          tunnel: [w580 w581] -> w557
          frame "s" {
            w580 = u16 0 items=["Single", "Double"] ("sweep mode")
          }
          frame "d", Default {
            w581 = u16 1 items=["Single", "Double"] ("sweep mode")
          }
        }
        n129 = Fract/Exp String To Number(string=w558) -> (number=w553:dbl[])  [unwired: 3 in, 1 out]
        n130 = String To Path(string=w570) -> (path=w566:path)
        n131 = Index Array(array=w553, index #1=0 ("Index")) -> (element #1=w530:dbl, element #2=w529:dbl, element #3=w526:dbl, element #4=w525:dbl, element #5=w524:dbl, element #6=w528:dbl)  [unwired: 5 in]
        n132 = Bundle By Name(cluster=w527, "Pulse period"=w525, "Base voltage"=w526, "Pulse width"=w524) -> (w523:T6)
        n133 = Unbundle By Name(w523) -> ("Pulse period"=w531:dbl)
        n134 = Bundle By Name(cluster=w555, "Gate Start"=w529, "Gate Stop"=w530, "Gate Step (linear only)"=0, "Gate Compliance"=w564, "Range mode"=w545, "Range"=w544) -> (w546:T4)
        n135 = call <vilib>:"compatOverwrite.vi"("overwrite (F)"=TRUE) -> ("overwrite?"=w516:T7)
        n136 = Bundle By Name(cluster=w554, "Drain Start"=w528, "Drain Stop"=w521, "Drain Step"=w521, "Drain Compliance"=w565, "Range mode"=w543, "Range"=w542) -> (w547:T5)
        n137 = call "4155C PulsedStressV.vi"("VISA resource name in"=w549, "sweep mode"=w557, "Panel Controls"=w540, "Gate"=w546, "Drain"=w547, "Timings"=w523, "error in (no error)"=w550, "SMU4"=w539) -> ("VISA Resource Name out"=w562:refnum<visa-resource-name>, "ID"=w519:dbl[], "IG"=w517:dbl[], "Outparams"=w541:T8, "error out"=w563:errorcluster)  [unwired: 3 in]
        n138 = Unbundle By Name(w541) -> ("Number of points"=w518:i32)  [unwired: 2 out]
        n139 = for {
          N: w518 -> [_]
          tunnel: [w577] -> w520 mode=indexing
          tunnel: w531 -> [w579]
          i -> [w578]
          n140 = Multiply(x=w579, y=w578) -> (x*y=w577:dbl)
        }
        n141 = Insert Into Array(array=dbl[][] [] ("Input Array"), new element=w520) -> (w532:dbl[][])  [unwired: 2 in]
        n142 = Insert Into Array(array=w532, new element=w519) -> (w537:dbl[][])  [unwired: 2 in]
        n143 = Insert Into Array(array=w537, new element=w517) -> (w536:dbl[][])  [unwired: 2 in]
        n144 = Transpose 2D Array(2D array=w536) -> (transposed array=w535:dbl[][])
        n145 = Open/Create/Replace File(file path (use dialog)=w566, error in=w563, operation (0:open)=w516) -> (refnum out=w574:refnum<file>, error out=w575:errorcluster)  [unwired: 3 in, 1 out]
        n146 = call "4155C Write array to file.vi"("Byte Stream File Refnum"=w574, "Header"=string[] ["Time /s", "Id /A", "Ig /A"], "Data Array"=w535, "error in (no error)"=w575) -> ("dup refnum"=w572:refnum<file>, "error out"=w573:errorcluster)  [unwired: 1 in]
        n147 = Close File(refnum=w572, error in=w573) -> (error out=w561:errorcluster)  [unwired: 1 out]
      }
      frame "transfer-fpp" {
        n148 = Number To Decimal String(number=w603) -> (decimal integer string=w657:string)  [unwired: 1 in]
        n149 = Bundle By Name(cluster=w633, "Emergency Stop"=w661) -> (w669:T1)
        n150 = Delete From Array(array=w648, index=0 ("Index")) -> (deleted portion=w646:string, array with subset deleted=w645:string[])  [unwired: 1 in]
        n151 = Concatenate Strings(w656, "-transferfpp-" ("Substring"), w657, w601, ".txt" ("Substring")) -> (w659:string)
        n152 = VISA Write(VISA resource name=w625, write buffer=":PAGE:CHAN:MODE SWE;" ("write buffer (\"\")"), error in (no error)=w624) -> (VISA resource name out=w622:refnum<visa-resource-name>, error out=w623:errorcluster)  [unwired: 1 out]
        n153 = case shown="\"d\", Default" w646 {
          tunnel: [w670 w671] -> w644
          frame "s" {
            w670 = u16 0 items=["Single", "Double"] ("sweep mode")
          }
          frame "d", Default {
            w671 = u16 1 items=["Single", "Double"] ("sweep mode")
          }
        }
        n154 = Fract/Exp String To Number(string=w645) -> (number=w629:dbl[])  [unwired: 3 in, 1 out]
        n155 = String To Path(string=w659) -> (path=w655:path)
        n156 = Index Array(array=w629, index #1=0 ("Index")) -> (element #1=w643:dbl, element #2=w642:dbl, element #3=w641:dbl)  [unwired: 2 in]
        n157 = Delete From Array(array=w629, length=3 ("Length"), index=0 ("Index")) -> (array with subset deleted=w627:dbl[])  [unwired: 1 out]
        n158 = Bundle By Name(cluster=w635, "Gate Start"=w643, "Gate Stop"=w642, "Gate Step (linear only)"=w641, "Gate Compliance"=w653, "Range mode"=w618, "Range"=w617) -> (w619:T4)
        n159 = Index Array(array=w627, index #1=0 ("Index")) -> (element #1=w638:dbl, element #2=w637:dbl, element #3=w636:dbl)  [unwired: 2 in]
        n160 = call <vilib>:"compatOverwrite.vi"("overwrite (F)"=TRUE) -> ("overwrite?"=w606:T7)
        n161 = Bundle By Name(cluster=w634, "Drain Start"=w638, "Drain Stop"=w637, "Drain Step"=w636, "Drain Compliance"=w654, "Range mode"=w616, "Range"=w615) -> (w620:T5)
        n162 = call "4155C Transfer-FPP.vi"("VISA resource name in"=w622, "Gate"=w619, "Drain"=w620, "Timings"=w652, "error in (no error)"=w623, "sweep mode"=w644, "Panel Controls"=w669) -> ("VG"=w660:dbl[], "Outparams"=w614:T8, "VISA Resource Name out"=w650:refnum<visa-resource-name>, "Vprobe2"=w610:dbl[], "ID"=w609:dbl[], "IG"=w608:dbl[], "Vprobe1"=w607:dbl[], "error out"=w651:errorcluster)  [unwired: 13 in]
        n163 = Unbundle By Name(w614) -> ("V2 Step"=w613:dbl, "V2 Start"=w612:dbl, "Number of points"=w611:i32)
        n164 = Open/Create/Replace File(file path (use dialog)=w655, error in=w651, operation (0:open)=w606) -> (refnum out=w666:refnum<file>, error out=w667:errorcluster)  [unwired: 3 in, 1 out]
        n165 = call "4155C Make Big 2d array FPP.vi"("1D Var1"=w660, "1d ID"=w609, "1d Vp2"=w610, "1d IG"=w608, "1d Vp1"=w607, "VAR2 START"=w612, "Number of VAR2 steps"=w611, "VAR2 STEP"=w613, "VAR1 Name"="Vg", "Decimal places in header"=i8 1, "VAR2 Name"="Vd") -> ("Header array"=w662:string[], "Data array"=w663:dbl[][])  [unwired: 15 in]
        n166 = call "4155C Write array to file.vi"("Byte Stream File Refnum"=w666, "Header"=w662, "Data Array"=w663, "error in (no error)"=w667) -> ("dup refnum"=w664:refnum<file>, "error out"=w665:errorcluster)  [unwired: 1 in]
        n167 = Close File(refnum=w664, error in=w665) -> (error out=w649:errorcluster)  [unwired: 1 out]
      }
      frame "output" {
        n168 = Number To Decimal String(number=w701) -> (decimal integer string=w750:string)  [unwired: 1 in]
        n169 = Bundle By Name(cluster=w727, "Emergency Stop"=w752) -> (w762:T1)
        n170 = Delete From Array(array=w742, index=0 ("Index")) -> (deleted portion=w740:string, array with subset deleted=w739:string[])  [unwired: 1 in]
        n171 = Concatenate Strings(w749, w672, w750, w700, "_O.txt" ("Suffix (output)")) -> (w751:string)
        n172 = VISA Write(VISA resource name=w718, write buffer=":PAGE:CHAN:MODE SWE;" ("write buffer (\"\")"), error in (no error)=w715) -> (VISA resource name out=w717:refnum<visa-resource-name>, error out=w716:errorcluster)  [unwired: 1 out]
        n173 = case shown="\"d\", Default" w740 {
          tunnel: [w763 w764] -> w738
          frame "s" {
            w763 = u16 0 items=["Single", "Double"] ("sweep mode")
          }
          frame "d", Default {
            w764 = u16 1 items=["Single", "Double"] ("sweep mode")
          }
        }
        n174 = Fract/Exp String To Number(string=w739) -> (number=w721:dbl[])  [unwired: 3 in, 1 out]
        n175 = String To Path(string=w751) -> (path=w748:path)
        n176 = Index Array(array=w721, index #1=0 ("Index")) -> (element #1=w737:dbl, element #2=w736:dbl, element #3=w735:dbl)  [unwired: 2 in]
        n177 = Delete From Array(array=w721, length=3 ("Length"), index=0 ("Index")) -> (array with subset deleted=w720:dbl[])  [unwired: 1 out]
        n178 = control-ref of="I vs Vd"() -> (w691:refnum<vi>)
        n179 = Bundle By Name(cluster=w729, "Gate Start"=w737, "Gate Stop"=w736, "Gate Step (linear only)"=w735, "Gate Compliance"=w746, "Range mode"=w713, "Range"=w712) -> (w761:T4)
        n180 = Index Array(array=w720, index #1=0 ("Index")) -> (element #1=w732:dbl, element #2=w731:dbl, element #3=w730:dbl)  [unwired: 2 in]
        n181 = call <vilib>:"compatOverwrite.vi"("overwrite (F)"=TRUE) -> ("overwrite?"=w705:T7)
        n182 = Bundle By Name(cluster=w728, "Drain Start"=w732, "Drain Stop"=w731, "Drain Step"=w730, "Drain Compliance"=w747, "Range mode"=w711, "Range"=w714) -> (w760:T5)
        n183 = call "4155C Output.vi"("VISA resource name in"=w717, "Gate"=w761, "Drain"=w760, "Timings"=w745, "error in (no error)"=w716, "SMU4"=w707, "sweep mode"=w738, "Panel controls"=w762) -> ("VD"=w698:dbl[], "Outparams"=w709:T8, "VISA Resource Name out"=w744:refnum<visa-resource-name>, "IS"=w697:dbl[], "ID"=w696:dbl[], "IG"=w695:dbl[], "error out"=w693:errorcluster, "SMU4"=w706:dbl[])  [unwired: 12 in]
        n184 = Unbundle By Name(w709) -> ("V2 Step"=w710:dbl, "V2 Start"=w708:dbl, "Number of points"=w690:i32)
        n185 = call "4155C Split array.vi"("Number of VAR2 steps"=w690, "Y2 data in"=w696, "X data in"=w698, "Y1 data in"=w697, "Y3 data in"=w695, "error in (no error)"=w693) -> ("Array of clusters"=w694:cluster{"Y data in":dbl[], "X data in":dbl[]}[], "error out"=w692:errorcluster)  [unwired: 1 in]
        n186 = local write "I vs Vd"(w694) -> ()
        n187 = call "4155C Config Chart Colours.vi"("Numeric"=w690, "XY Graph 2"=w691) -> ()  [unwired: 6 in]
        n188 = Open/Create/Replace File(file path (use dialog)=w748, error in=w692, operation (0:open)=w705) -> (refnum out=w757:refnum<file>, error out=w758:errorcluster)  [unwired: 3 in, 1 out]
        n189 = call "4155C Make Big 2d array.vi"("1D Var1"=w698, "1d IS"=w697, "1d ID"=w696, "1d IG"=w695, "1d SMU4"=w706, "SMU4"=w707, "VAR2 START"=w708, "Number of VAR2 steps"=w690, "VAR2 STEP"=w710, "VAR1 Name"="Vd", "Decimal places in header"=i8 1, "VAR2 Name"="Vg") -> ("Header array"=w753:string[], "Data array"=w754:dbl[][])  [unwired: 14 in]
        n190 = call "4155C Write array to file.vi"("Byte Stream File Refnum"=w757, "Header"=w753, "Data Array"=w754, "error in (no error)"=w758) -> ("dup refnum"=w755:refnum<file>, "error out"=w756:errorcluster)  [unwired: 1 in]
        n191 = Close File(refnum=w755, error in=w756) -> (error out=w743:errorcluster)  [unwired: 1 out]
      }
      frame "output2" {
        # "Adjusts graph colors."
        # "Adjusts graph colors."
        # "Is off"
        # "Is on"
        # "Ion will be the middle element of the array. The calculation of the index is done only once, since Is, Id, and Ig have the same dimensions."
        # "Ig off"
        # "Ig on"
        # "Is min"
        # "Is max"
        # "Ig min"
        # "Ig max"
        # "abs(Ig)"
        # "abs(Is)"
        # "Id min"
        # "Id max"
        # "Y1: Is\nY2: Id\nY3: Ig"
        # "abs(Id)"
        # "Adjusts graph colors."
        # "Adjusts graph colors."
        # "Id off"
        # "Id on"
        # "Adjusts graph colors."
        # "Time array"
        n192 = Delete From Array(array=w894, index=0 ("Index")) -> (deleted portion=w892:string, array with subset deleted=w891:string[])  [unwired: 1 in]
        n193 = Bundle By Name(cluster=w765, "Emergency Stop"=w903) -> (w856:T1)
        n194 = Number To Decimal String(number=w850) -> (decimal integer string=w849:string)  [unwired: 1 in]
        n195 = case shown="\"d\", Default" w892 {
          tunnel: [w905 w906] -> w890
          frame "s" {
            w905 = u16 0 items=["Single", "Double"] ("sweep mode")
          }
          frame "d", Default {
            w906 = u16 1 items=["Single", "Double"] ("sweep mode")
          }
        }
        n196 = Fract/Exp String To Number(string=w891) -> (number=w876:dbl[])  [unwired: 3 in, 1 out]
        n197 = Concatenate Strings(w901, w766, w849, w847, "_O_1_C_L.txt" ("Suffix (transfer)")) -> (w902:string)
        n198 = VISA Write(VISA resource name=w872, write buffer=":PAGE:CHAN:MODE SWE;" ("write buffer (\"\")"), error in (no error)=w871) -> (VISA resource name out=w869:refnum<visa-resource-name>, error out=w870:errorcluster)  [unwired: 1 out]
        n199 = String To Path(string=w902) -> (path=w900:path)
        n200 = Index Array(array=w876, index #1=0 ("Index")) -> (element #1=w889:dbl, element #2=w888:dbl, element #3=w887:dbl)  [unwired: 2 in]
        n201 = Delete From Array(array=w876, length=3 ("Length"), index=0 ("Index")) -> (array with subset deleted=w874:dbl[])  [unwired: 1 out]
        n202 = Build Array (concatenate)(w846, w842) -> (w792:i32[])
        n203 = Bundle By Name(cluster=w881, "Gate Start"=w889, "Gate Stop"=w888, "Gate Step (linear only)"=w887, "Gate Compliance"=w898, "Range mode"=w865, "Range"=w864) -> (w866:T4)
        n204 = control-ref of="Imax vs time"() -> (w821:refnum<vi>)
        n205 = control-ref of="Imin vs time"() -> (w820:refnum<vi>)
        n206 = control-ref of="Ion vs time"() -> (w789:refnum<vi>)
        n207 = control-ref of="Ioff vs time"() -> (w788:refnum<vi>)
        n208 = control-ref of="I vs Vg"() -> (w851:refnum<vi>)
        n209 = Index Array(array=w874, index #1=0 ("Index")) -> (element #1=w884:dbl, element #2=w883:dbl, element #3=w882:dbl)  [unwired: 2 in]
        n210 = call <vilib>:"compatOverwrite.vi"("overwrite (F)"=TRUE) -> ("overwrite?"=w855:T7)
        n211 = Bundle By Name(cluster=w880, "Drain Start"=w884, "Drain Stop"=w883, "Drain Step"=w882, "Drain Compliance"=w899, "Range mode"=w863, "Range"=w862) -> (w867:T5)
        n212 = call "4155C Output.vi"("VISA resource name in"=w869, "Gate"=w866, "Drain"=w867, "Timings"=w897, "error in (no error)"=w870, "SMU4"=w857, "sweep mode"=w890, "Panel controls"=w856) -> ("VD"=w854:dbl[], "Outparams"=w861:T8, "VISA Resource Name out"=w896:refnum<visa-resource-name>, "IS"=w817:dbl[], "ID"=w819:dbl[], "IG"=w816:dbl[], "error out"=w843:errorcluster, "SMU4"=w858:dbl[])  [unwired: 12 in]
        n213 = Unbundle By Name(w861) -> ("V2 Step"=w860:dbl, "V2 Start"=w859:dbl, "Number of points"=w786:i32)
        n214 = Absolute Value(x=w817) -> (abs(x)=w802:dbl[])
        n215 = Absolute Value(x=w819) -> (abs(x)=w818:dbl[])
        n216 = Absolute Value(x=w816) -> (abs(x)=w805:dbl[])
        n217 = Array Size(array=w818) -> (size(s)=w826:i32)
        n218 = Divide(x=w826, y=2) -> (x/y=w769:dbl)
        n219 = Subtract(x=w769, y=1) -> (x-y=w768:dbl)
        n220 = Array Max & Min(array=w802) -> (max value=w809:dbl, min value=w810:dbl)  [unwired: 2 out]
        n221 = Array Max & Min(array=w818) -> (max value=w852:dbl, min value=w815:dbl)  [unwired: 2 out]
        n222 = Array Max & Min(array=w805) -> (max value=w814:dbl, min value=w813:dbl)  [unwired: 2 out]
        n223 = call "4155C Split array.vi"("Number of VAR2 steps"=w786, "Y2 data in"=w819, "X data in"=w854, "Y1 data in"=w817, "Y3 data in"=w816, "error in (no error)"=w843) -> ("Array of clusters"=w845:cluster{"Y data in":dbl[], "X data in":dbl[]}[], "error out"=w774:errorcluster)  [unwired: 1 in]
        n224 = Index Array(array=w802, index=w768) -> (element=w793:dbl)
        n225 = Index Array(array=w802, index=0) -> (element=w794:dbl)
        n226 = Index Array(array=w818, index=w768) -> (element=w795:dbl)
        n227 = Index Array(array=w818, index=0) -> (element=w796:dbl)
        n228 = Index Array(array=w805, index=w768) -> (element=w798:dbl)
        n229 = Index Array(array=w805, index=0) -> (element=w797:dbl)
        n230 = local write "Ig max"(w814) -> ()
        n231 = local write "Ig min"(w813) -> ()
        n232 = local write "Is max"(w809) -> ()
        n233 = local write "Is min"(w810) -> ()
        n234 = local write "Id max"(w852) -> ()
        n235 = local write "Id min"(w815) -> ()
        n236 = local write "I vs Vd"(w845) -> ()
        n237 = Build Array (concatenate)(w808, w809) -> (w787:dbl[])
        n238 = Build Array (concatenate)(w807, w810) -> (w785:dbl[])
        n239 = local write "Is off"(w794) -> ()
        n240 = local write "Is on"(w793) -> ()
        n241 = Build Array (concatenate)(w853, w852) -> (w784:dbl[])
        n242 = Build Array (concatenate)(w840, w815) -> (w783:dbl[])
        n243 = Build Array (concatenate)(w812, w814) -> (w782:dbl[])
        n244 = Build Array (concatenate)(w811, w813) -> (w781:dbl[])
        n245 = Build Array (concatenate)(w800, w793) -> (w780:dbl[])
        n246 = Build Array (concatenate)(w799, w794) -> (w779:dbl[])
        n247 = Build Array (concatenate)(w822, w795) -> (w778:dbl[])
        n248 = Build Array (concatenate)(w823, w796) -> (w777:dbl[])
        n249 = Build Array (concatenate)(w804, w798) -> (w776:dbl[])
        n250 = Build Array (concatenate)(w803, w797) -> (w775:dbl[])
        n251 = local write "Ig off"(w797) -> ()
        n252 = local write "Ig on"(w798) -> ()
        n253 = local write "Id off"(w796) -> ()
        n254 = local write "Id on"(w795) -> ()
        n255 = call "4155C Split array.vi"("Number of VAR2 steps"=w786, "Y2 data in"=w778, "X data in"=w792, "Y1 data in"=w780, "Y3 data in"=w776, "error in (no error)"=w774) -> ("Array of clusters"=w790:cluster{"Y data in":dbl[], "X data in":dbl[]}[], "error out"=w773:errorcluster)  [unwired: 1 in]
        n256 = call "4155C Split array.vi"("Number of VAR2 steps"=w786, "Y2 data in"=w777, "X data in"=w792, "Y1 data in"=w779, "Y3 data in"=w775, "error in (no error)"=w773) -> ("Array of clusters"=w791:cluster{"Y data in":dbl[], "X data in":dbl[]}[], "error out"=w772:errorcluster)  [unwired: 1 in]
        n257 = call "4155C Split array.vi"("Number of VAR2 steps"=w786, "Y2 data in"=w784, "X data in"=w792, "Y1 data in"=w787, "Y3 data in"=w782, "error in (no error)"=w772) -> ("Array of clusters"=w844:cluster{"Y data in":dbl[], "X data in":dbl[]}[], "error out"=w771:errorcluster)  [unwired: 1 in]
        n258 = call "4155C Split array.vi"("Number of VAR2 steps"=w786, "Y2 data in"=w783, "X data in"=w792, "Y1 data in"=w785, "Y3 data in"=w781, "error in (no error)"=w771) -> ("Array of clusters"=w841:cluster{"Y data in":dbl[], "X data in":dbl[]}[], "error out"=w770:errorcluster)  [unwired: 1 in]
        n259 = Open/Create/Replace File(file path (use dialog)=w900, error in=w770, operation (0:open)=w855) -> (refnum out=w838:refnum<file>, error out=w836:errorcluster)  [unwired: 3 in, 1 out]
        n260 = call "4155C Make Big 2d array.vi"("1D Var1"=w854, "1d IS"=w817, "1d ID"=w819, "1d IG"=w816, "1d SMU4"=w858, "SMU4"=w857, "VAR2 START"=w859, "Number of VAR2 steps"=w786, "VAR2 STEP"=w860, "VAR1 Name"="Vd", "Decimal places in header"=i8 1, "VAR2 Name"="Vg") -> ("Header array"=w839:string[], "Data array"=w837:dbl[][])  [unwired: 14 in]
        n261 = local write "Imax vs time"(w844) -> ()
        n262 = local write "Imin vs time"(w841) -> ()
        n263 = local write "Ion vs time"(w790) -> ()
        n264 = local write "Ioff vs time"(w791) -> ()
        n265 = call "4155C Config Chart Colours.vi"("Numeric"=w786, "XY Graph 2"=w821) -> ()  [unwired: 6 in]
        n266 = call "4155C Config Chart Colours.vi"("Numeric"=w786, "XY Graph 2"=w820) -> ()  [unwired: 6 in]
        n267 = call "4155C Config Chart Colours.vi"("Numeric"=w786, "XY Graph 2"=w789) -> ()  [unwired: 6 in]
        n268 = call "4155C Config Chart Colours.vi"("Numeric"=w786, "XY Graph 2"=w788) -> ()  [unwired: 6 in]
        n269 = call "4155C Config Chart Colours.vi"("Numeric"=w786, "XY Graph 2"=w851) -> ()  [unwired: 6 in]
        n270 = call "4155C Write array to file.vi"("Byte Stream File Refnum"=w838, "Header"=w839, "Data Array"=w837, "error in (no error)"=w836) -> ("dup refnum"=w835:refnum<file>, "error out"=w834:errorcluster)  [unwired: 1 in]
        n271 = Close File(refnum=w835, error in=w834) -> (error out=w895:errorcluster)  [unwired: 1 out]
      }
      frame "output-fpp" {
        n272 = Number To Decimal String(number=w927) -> (decimal integer string=w981:string)  [unwired: 1 in]
        n273 = Bundle By Name(cluster=w957, "Emergency Stop"=w984) -> (w994:T1)
        n274 = Delete From Array(array=w972, index=0 ("Index")) -> (deleted portion=w970:string, array with subset deleted=w969:string[])  [unwired: 1 in]
        n275 = VISA Write(VISA resource name=w948, write buffer=":PAGE:CHAN:MODE SWE;" ("write buffer (\"\")"), error in (no error)=w945) -> (VISA resource name out=w947:refnum<visa-resource-name>, error out=w946:errorcluster)  [unwired: 1 out]
        n276 = Concatenate Strings(w980, "-outputfpp-" ("Substring"), w981, w926, ".txt" ("Substring")) -> (w983:string)
        n277 = case shown="\"d\", Default" w970 {
          tunnel: [w995 w996] -> w968
          frame "s" {
            w995 = u16 0 items=["Single", "Double"] ("sweep mode")
          }
          frame "d", Default {
            w996 = u16 1 items=["Single", "Double"] ("sweep mode")
          }
        }
        n278 = Fract/Exp String To Number(string=w969) -> (number=w951:dbl[])  [unwired: 3 in, 1 out]
        n279 = String To Path(string=w983) -> (path=w979:path)
        n280 = Index Array(array=w951, index #1=0 ("Index")) -> (element #1=w967:dbl, element #2=w966:dbl, element #3=w965:dbl)  [unwired: 2 in]
        n281 = Delete From Array(array=w951, length=3 ("Length"), index=0 ("Index")) -> (array with subset deleted=w950:dbl[])  [unwired: 1 out]
        n282 = Bundle By Name(cluster=w959, "Gate Start"=w967, "Gate Stop"=w966, "Gate Step (linear only)"=w965, "Gate Compliance"=w977, "Range mode"=w943, "Range"=w942) -> (w993:T4)
        n283 = Index Array(array=w950, index #1=0 ("Index")) -> (element #1=w962:dbl, element #2=w961:dbl, element #3=w960:dbl)  [unwired: 2 in]
        n284 = call <vilib>:"compatOverwrite.vi"("overwrite (F)"=TRUE) -> ("overwrite?"=w931:T7)
        n285 = Bundle By Name(cluster=w958, "Drain Start"=w962, "Drain Stop"=w961, "Drain Step"=w960, "Drain Compliance"=w978, "Range mode"=w941, "Range"=w944) -> (w992:T5)
        n286 = call "4155C Output-FPP.vi"("VISA resource name in"=w947, "Gate"=w993, "Drain"=w992, "Timings"=w976, "error in (no error)"=w946, "sweep mode"=w968, "Panel controls"=w994) -> ("VD"=w936:dbl[], "Outparams"=w939:T8, "VISA Resource Name out"=w974:refnum<visa-resource-name>, "Vprobe2"=w935:dbl[], "ID"=w934:dbl[], "IG"=w933:dbl[], "Vprobe1"=w932:dbl[], "error out"=w975:errorcluster)  [unwired: 13 in]
        n287 = Unbundle By Name(w939) -> ("V2 Step"=w940:dbl, "V2 Start"=w938:dbl, "Number of points"=w937:i32)
        n288 = Open/Create/Replace File(file path (use dialog)=w979, error in=w975, operation (0:open)=w931) -> (refnum out=w989:refnum<file>, error out=w990:errorcluster)  [unwired: 3 in, 1 out]
        n289 = call "4155C Make Big 2d array FPP.vi"("1D Var1"=w936, "1d ID"=w934, "1d Vp2"=w935, "1d IG"=w933, "1d Vp1"=w932, "VAR2 START"=w938, "Number of VAR2 steps"=w937, "VAR2 STEP"=w940, "VAR1 Name"="Vd", "Decimal places in header"=i8 1, "VAR2 Name"="Vg") -> ("Header array"=w985:string[], "Data array"=w986:dbl[][])  [unwired: 15 in]
        n290 = call "4155C Write array to file.vi"("Byte Stream File Refnum"=w989, "Header"=w985, "Data Array"=w986, "error in (no error)"=w990) -> ("dup refnum"=w987:refnum<file>, "error out"=w988:errorcluster)  [unwired: 1 in]
        n291 = Close File(refnum=w987, error in=w988) -> (error out=w973:errorcluster)  [unwired: 1 out]
      }
      frame "itime" {
        n292 = Delete From Array(array=w1029, index=0 ("Index")) -> (deleted portion=w1030:string)  [unwired: 1 in, 1 out]
        n293 = case shown="\"s\"" w1030 {
          tunnel: w1028 -> [w1034 w1036 w1039]
          tunnel: [w1033 w1035 w1038] -> w1021
          frame "s" {
            w1032 = u32 0 items=["short  ", "medium  ", "long  "] ("integration time 2")
            n294 = Bundle By Name(cluster=w1034, "integration time"=w1032) -> (w1033:T6)
          }
          frame "m", Default {
            w1037 = u32 1 items=["short  ", "medium  ", "long  "] ("integration time 2")
            n295 = Bundle By Name(cluster=w1036, "integration time"=w1037) -> (w1035:T6)
          }
          frame "l" {
            w1040 = u32 2 items=["short  ", "medium  ", "long  "] ("integration time 2")
            n296 = Bundle By Name(cluster=w1039, "integration time"=w1040) -> (w1038:T6)
          }
        }
      }
      frame "pulsed" {
        n297 = Delete From Array(array=w1074, index=0 ("Index")) -> (deleted portion=w1075:string, array with subset deleted=w1062:string[])  [unwired: 1 in]
        n298 = case shown="\"on\", Default" w1075 {
          tunnel: w1073 -> [w1085 w1088]
          tunnel: [w1084 w1087] -> w1066
          tunnel: w1062 -> [w1082 _]
          frame "on", Default {
            w1083 = u16 1 items=["Continuous", "Pulsed"] ("sweep method")
            n299 = Fract/Exp String To Number(string=w1082) -> (number=w1080:dbl[])  [unwired: 3 in, 1 out]
            n300 = Index Array(array=w1080, index #1=0 ("Index")) -> (element #1=w1079:dbl, element #2=w1078:dbl, element #3=w1077:dbl)  [unwired: 2 in]
            n301 = Bundle By Name(cluster=w1085, "sweep method"=w1083, "Pulse period"=w1079, "Base voltage"=w1078, "Pulse width"=w1077) -> (w1084:T6)
          }
          frame "off" {
            w1086 = u16 0 items=["Continuous", "Pulsed"] ("sweep method")
            n302 = Bundle By Name(cluster=w1088, "sweep method"=w1086) -> (w1087:T6)
          }
        }
      }
      frame "gaterangemode" {
        n303 = Delete From Array(array=w1120, index=0 ("Index")) -> (deleted portion=w1121:string)  [unwired: 1 in, 1 out]
        n304 = case shown="\"f\"" w1121 {
          tunnel: [w1123 w1124 w1125] -> w1110
          frame "a", Default {
            w1123 = u16 0 items=["Auto", "Limited", "Fixed"] ("Gate Range\nmode 2")
          }
          frame "f" {
            w1124 = u16 2 items=["Auto", "Limited", "Fixed"] ("Gate Range\nmode 2")
          }
          frame "l" {
            w1125 = u16 1 items=["Auto", "Limited", "Fixed"] ("Gate Range\nmode 2")
          }
        }
      }
      frame "gaterange" {
        (unwired) u8 11 items=["10fA  ", "100fA  ", "1nA  ", "10nA", "100nA", "1uA", "10uA", "100uA", "1mA", "10mA", "100mA", "1A"] ("Gate Range 2")
        n305 = Delete From Array(array=w1164, index=0 ("Index")) -> (deleted portion=w1154:string)  [unwired: 1 in, 1 out]
        n306 = Scan Value(string=w1154, format string="") -> (value=w1152:dbl)  [unwired: 1 in, 1 out]
        n307 = Logarithm Base 10(1:w1152) -> (0:w1151:dbl)
        n308 = Round To Nearest(number=w1151) -> (nearest integer value=w1150:dbl)
        n309 = Add(x=w1150, y=11.0) -> (x+y=w1148:dbl)
        n310 = To Unsigned Byte Integer(number=w1148) -> (unsigned 8bit integer=w1147:u8)
      }
      frame "drainrange" {
        (unwired) u8 11 items=["10fA  ", "100fA  ", "1nA  ", "10nA", "100nA", "1uA", "10uA", "100uA", "1mA", "10mA", "100mA", "1A"] ("Gate Range 2")
        n311 = Delete From Array(array=w1204, index=0 ("Index")) -> (deleted portion=w1195:string)  [unwired: 1 in, 1 out]
        n312 = Scan Value(string=w1195, format string="") -> (value=w1193:dbl)  [unwired: 1 in, 1 out]
        n313 = Logarithm Base 10(1:w1193) -> (0:w1192:dbl)
        n314 = Round To Nearest(number=w1192) -> (nearest integer value=w1191:dbl)
        n315 = Add(x=w1191, y=11.0) -> (x+y=w1189:dbl)
        n316 = To Unsigned Byte Integer(number=w1189) -> (unsigned 8bit integer=w1188:u8)
      }
      frame "drainrangemode" {
        n317 = Delete From Array(array=w1237, index=0 ("Index")) -> (deleted portion=w1238:string)  [unwired: 1 in, 1 out]
        n318 = case shown="\"f\"" w1238 {
          tunnel: [w1240 w1241 w1242] -> w1227
          frame "a", Default {
            w1240 = u16 0 items=["Auto", "Limited", "Fixed"] ("Gate Range\nmode 2")
          }
          frame "f" {
            w1241 = u16 2 items=["Auto", "Limited", "Fixed"] ("Gate Range\nmode 2")
          }
          frame "l" {
            w1242 = u16 1 items=["Auto", "Limited", "Fixed"] ("Gate Range\nmode 2")
          }
        }
      }
      frame "Error", Default {
      }
      frame "logfile" {
        n319 = Number To Decimal String(number=w1295) -> (decimal integer string=w1330:string)  [unwired: 1 in]
        n320 = Concatenate Strings(w1329, "logfile" ("Substring"), w1330, w1293, ".txt" ("Substring")) -> (w1327:string)
        n321 = String To Path(string=w1327) -> (path=w1300:path)
        n322 = Unbundle(w1326) -> ("integration time"=w1325:u32, "Short/Long integration time"=w1324:dbl, "hold time (sec)"=w1323:dbl, "delay time (sec)"=w1322:dbl, "Step Time (0 disables)"=w1321:dbl, "sweep method"=w1320:u16, "Pulse period"=w1319:dbl, "Base voltage"=w1318:dbl, "Pulse width"=w1317:dbl)
        n323 = Build Array(w1325, w1324, w1323, w1322, w1321, w1320, w1319, w1318, w1317, w1311, w1312, w1313, w1314, w1315, w1316) -> (w1304:dbl[])
        n324 = Insert Into Array(array=dbl[][] [] ("Input Array"), new element=w1304) -> (w1303:dbl[][])  [unwired: 2 in]
        n325 = call <vilib>:"compatOverwrite.vi"("overwrite (F)"=TRUE) -> ("overwrite?"=w1298:T7)
        n326 = Open/Create/Replace File(file path (use dialog)=w1300, error in=w1302, operation (0:open)=w1298) -> (refnum out=w1308:refnum<file>, error out=w1307:errorcluster)  [unwired: 3 in, 1 out]
        n327 = call "4155C Write array to file.vi"("Byte Stream File Refnum"=w1308, "Header"=string[] ["Int Time", "Short/Long Itime", "Hold time", "Delay time", "Step time", "Sweep method", "Pulse period", "Base Voltage", "Pulse width", "Drain compliance", "Gate compliance", "Gate range mode", "Gate range", "S/D range mode", "S/D range"], "Data Array"=w1303, "error in (no error)"=w1307) -> ("dup refnum"=w1310:refnum<file>, "error out"=w1309:errorcluster)  [unwired: 1 in]
        n328 = Close File(refnum=w1310, error in=w1309) -> (error out=w1301:errorcluster)  [unwired: 1 out]
      }
      frame "sample" {
        n329 = Number To Decimal String(number=w1353) -> (decimal integer string=w1401:string)  [unwired: 1 in]
        n330 = Fract/Exp String To Number(string=w1398) -> (number=w1359:dbl[])  [unwired: 3 in, 1 out]
        n331 = Concatenate Strings(w1376, "-sample-" ("Substring"), w1401, w1351, ".txt" ("Substring")) -> (w1399:string)
        n332 = Index Array(array=w1359, index=0 ("Index")) -> (element=w1396:dbl)
        n333 = String To Path(string=w1399) -> (path=w1380:path)
        n334 = Index Array(array=w1359, index=2 ("Index")) -> (element=w1392:dbl)
        n335 = Index Array(array=w1359, index=3 ("Index")) -> (element=w1361:dbl)
        n336 = Index Array(array=w1359, index=4 ("Index")) -> (element=w1358:dbl)
        n337 = call "4155C Config Sampling Measurements.vi"("Sampling interval"=w1358, "Sample time"=w1361, "Display on/off"=TRUE, "Timings"=w1367, "Num Points"=w1392, "error in (no error)"=w1403, "Drain Compliance"=w1402, "Gate Compliance"=w1377, "VISA session"=w1404) -> ("error out"=w1405:errorcluster, "dup VISA resource name"=w1406:refnum<visa-resource-name>)  [unwired: 1 in]
        n338 = Index Array(array=w1359, index=1 ("Index")) -> (element=w1393:dbl)
        n339 = call "4155C Take Sample.vi"("Emergency Stop"=w1373, "error in (no error)"=w1405, "Vd"=w1393, "Vg"=w1396, "VISA resource name in"=w1406) -> ("error out"=w1371:errorcluster, "Id"=w1408:dbl[], "Ig"=w1382:dbl[], "VISA Resource Name out"=w1369:refnum<visa-resource-name>, "Is"=w1407:dbl[], "Time"=w1386:dbl[])  [unwired: 1 in]
        n340 = Insert Into Array(array=dbl[][] [] ("Input Array"), new element=w1386) -> (w1385:dbl[][])  [unwired: 2 in]
        n341 = Insert Into Array(array=w1385, new element=w1382) -> (w1384:dbl[][])  [unwired: 2 in]
        n342 = Insert Into Array(array=w1384, new element=w1408) -> (w1383:dbl[][])  [unwired: 2 in]
        n343 = VISA Write(VISA resource name=w1369, write buffer=":DISP ON" ("write buffer (\"\")"), error in (no error)=w1371) -> (VISA resource name out=w1368:refnum<visa-resource-name>, error out=w1370:errorcluster)  [unwired: 1 out]
        n344 = Insert Into Array(array=w1383, new element=w1407) -> (w1375:dbl[][])  [unwired: 2 in]
        n345 = Transpose 2D Array(2D array=w1375) -> (transposed array=w1374:dbl[][])
        n346 = call <vilib>:"compatOverwrite.vi"("overwrite (F)"=TRUE) -> ("overwrite?"=w1356:T7)
        n347 = Open/Create/Replace File(file path (use dialog)=w1380, error in=w1370, operation (0:open)=w1356) -> (refnum out=w1389:refnum<file>, error out=w1388:errorcluster)  [unwired: 3 in, 1 out]
        n348 = call "4155C Write array to file.vi"("Byte Stream File Refnum"=w1389, "Header"=string[] ["Time /s", "Ig /A", "Id /A", "Is /A"], "Data Array"=w1374, "error in (no error)"=w1388) -> ("dup refnum"=w1391:refnum<file>, "error out"=w1390:errorcluster)  [unwired: 1 in]
        n349 = Close File(refnum=w1391, error in=w1390) -> (error out=w1378:errorcluster)  [unwired: 1 out]
      }
      frame "samplei" {
        n350 = Number To Decimal String(number=w1430) -> (decimal integer string=w1481:string)  [unwired: 1 in]
        n351 = Concatenate Strings(w1460, "-samplei-" ("Substring"), w1481, w1429, ".txt" ("Substring")) -> (w1479:string)
        n352 = Fract/Exp String To Number(string=w1478) -> (number=w1445:dbl[])  [unwired: 3 in, 1 out]
        n353 = String To Path(string=w1479) -> (path=w1463:path)
        n354 = Index Array(array=w1445, index=4 ("Index")) -> (element=w1439:dbl)
        n355 = Index Array(array=w1445, index=3 ("Index")) -> (element=w1440:dbl)
        n356 = Index Array(array=w1445, index=1 ("Index")) -> (element=w1442:dbl)
        n357 = Index Array(array=w1445, index=0 ("Index")) -> (element=w1443:dbl)
        n358 = Index Array(array=w1445, index=2 ("Index")) -> (element=w1441:dbl)
        n359 = call "4155C Config SamplingI Measurements.vi"("Sample time"=w1441, "Display on/off"=TRUE, "Timings"=w1452, "Num Points"=w1442, "error in (no error)"=w1483, "Sampling interval"=w1440, "VISA session"=w1484) -> ("error out"=w1485:errorcluster, "dup VISA resource name"=w1486:refnum<visa-resource-name>)  [unwired: 3 in]
        n360 = call "4155C Take SampleI.vi"("Emergency Stop"=w1457, "error in (no error)"=w1485, "Idg 2"=w1443, "Vdg compliance 2"=w1439, "VISA resource name in"=w1486) -> ("error out"=w1455:errorcluster, "Idg"=w1488:dbl[], "Vdg"=w1465:dbl[], "VISA Resource Name out"=w1453:refnum<visa-resource-name>, "Is"=w1487:dbl[], "Time"=w1469:dbl[])  [unwired: 1 in]
        n361 = Insert Into Array(array=dbl[][] [] ("Input Array"), new element=w1469) -> (w1468:dbl[][])  [unwired: 2 in]
        n362 = Insert Into Array(array=w1468, new element=w1465) -> (w1467:dbl[][])  [unwired: 2 in]
        n363 = Insert Into Array(array=w1467, new element=w1488) -> (w1466:dbl[][])  [unwired: 2 in]
        n364 = VISA Write(VISA resource name=w1453, write buffer=":DISP ON" ("write buffer (\"\")"), error in (no error)=w1455) -> (VISA resource name out=w1438:refnum<visa-resource-name>, error out=w1454:errorcluster)  [unwired: 1 out]
        n365 = Insert Into Array(array=w1466, new element=w1487) -> (w1459:dbl[][])  [unwired: 2 in]
        n366 = call <vilib>:"compatOverwrite.vi"("overwrite (F)"=TRUE) -> ("overwrite?"=w1433:T7)
        n367 = Open/Create/Replace File(file path (use dialog)=w1463, error in=w1454, operation (0:open)=w1433) -> (refnum out=w1472:refnum<file>, error out=w1471:errorcluster)  [unwired: 3 in, 1 out]
        n368 = Transpose 2D Array(2D array=w1459) -> (transposed array=w1458:dbl[][])
        n369 = call "4155C Write array to file.vi"("Byte Stream File Refnum"=w1472, "Header"=string[] ["Time /s", "Vdg /V", "Idg /A", "Is /A"], "Data Array"=w1458, "error in (no error)"=w1471) -> ("dup refnum"=w1474:refnum<file>, "error out"=w1473:errorcluster)  [unwired: 1 in]
        n370 = Close File(refnum=w1474, error in=w1473) -> (error out=w1436:errorcluster)  [unwired: 1 out]
        n371 = VISA Write(VISA resource name=w1438, write buffer=";:PAGE:SCON:STAN OFF;:PAGE:CHAN:VSU2:DIS;" ("write buffer (\"\")"), error in (no error)=w1436) -> (VISA resource name out=w1434:refnum<visa-resource-name>, error out=w1435:errorcluster)  [unwired: 1 out]
      }
      frame "#" {
        n372 = VISA Write(VISA resource name=w1514, write buffer=":DISP ON" ("write buffer (\"\")"), error in (no error)=w1513) -> (VISA resource name out=w1512:refnum<visa-resource-name>, error out=w1511:errorcluster)  [unwired: 1 out]
      }
      frame "stressV" {
        n373 = Number To Decimal String(number=w1543) -> (decimal integer string=w1584:string)  [unwired: 1 in]
        n374 = Concatenate Strings(w1568, "-stressV-" ("Substring"), w1584, w1542, ".txt" ("Substring")) -> (w1582:string)
        n375 = Fract/Exp String To Number(string=w1581) -> (number=w1554:dbl[])  [unwired: 3 in, 1 out]
        n376 = String To Path(string=w1582) -> (path=w1572:path)
        n377 = Index Array(array=w1554, index=3 ("Index")) -> (element=w1551:dbl)
        n378 = Index Array(array=w1554, index=1 ("Index")) -> (element=w1549:dbl)
        n379 = Index Array(array=w1554, index=0 ("Index")) -> (element=w1548:dbl)
        n380 = Index Array(array=w1554, index=4 ("Index")) -> (element=w1553:dbl)
        n381 = Index Array(array=w1554, index=2 ("Index")) -> (element=w1550:dbl)
        n382 = call "4155C Config V Stress.vi"("VISA session"=w1587, "ID compliance"=w1551, "VD"=w1549, "VG"=w1548, "IG compliance"=w1550, "error in (no error)"=w1586, "Display on/off"=TRUE) -> ("dup VISA resource name"=w1589:refnum<visa-resource-name>, "error out"=w1588:errorcluster)
        n383 = call "4155C Apply Stress.vi"("error in (no error)"=w1588, "Duration"=w1553, "Emergency Stop"=w1567, "VISA resource name in"=w1589) -> ("error out"=w1565:errorcluster, "VISA Resource Name out"=w1563:refnum<visa-resource-name>)
        n384 = VISA Write(VISA resource name=w1563, write buffer=":DISP ON" ("write buffer (\"\")"), error in (no error)=w1565) -> (VISA resource name out=w1562:refnum<visa-resource-name>, error out=w1564:errorcluster)  [unwired: 1 out]
        n385 = call <vilib>:"compatOverwrite.vi"("overwrite (F)"=TRUE) -> ("overwrite?"=w1547:T7)
        n386 = Open/Create/Replace File(file path (use dialog)=w1572, error in=w1564, operation (0:open)=w1547) -> (refnum out=w1575:refnum<file>, error out=w1574:errorcluster)  [unwired: 3 in, 1 out]
        n387 = call "4155C Write array to file.vi"("Byte Stream File Refnum"=w1575, "Header"=string[] ["V stress completed successfully", ""], "error in (no error)"=w1574) -> ("dup refnum"=w1577:refnum<file>, "error out"=w1576:errorcluster)  [unwired: 2 in]
        n388 = Close File(refnum=w1577, error in=w1576) -> (error out=w1570:errorcluster)  [unwired: 1 out]
      }
      frame "stressI" {
        n389 = Number To Decimal String(number=w1610) -> (decimal integer string=w1647:string)  [unwired: 1 in]
        n390 = Concatenate Strings(w1631, "-stressI-" ("Substring"), w1647, w1609, ".txt" ("Substring")) -> (w1645:string)
        n391 = Fract/Exp String To Number(string=w1644) -> (number=w1619:dbl[])  [unwired: 3 in, 1 out]
        n392 = Index Array(array=w1619, index=1 ("Index")) -> (element=w1615:dbl)
        n393 = Index Array(array=w1619, index=0 ("Index")) -> (element=w1616:dbl)
        n394 = call "4155C Config I Stress.vi"("VISA session"=w1650, "IDG"=w1616, "VDG compliance"=w1615, "error in (no error)"=w1649, "Display on/off"=TRUE) -> ("dup VISA resource name"=w1652:refnum<visa-resource-name>, "error out"=w1651:errorcluster)
        n395 = Index Array(array=w1619, index=2 ("Index")) -> (element=w1617:dbl)
        n396 = String To Path(string=w1645) -> (path=w1635:path)
        n397 = call "4155C Apply Stress.vi"("error in (no error)"=w1651, "Duration"=w1617, "Emergency Stop"=w1630, "VISA resource name in"=w1652) -> ("error out"=w1628:errorcluster, "VISA Resource Name out"=w1626:refnum<visa-resource-name>)
        n398 = VISA Write(VISA resource name=w1626, write buffer=":DISP ON" ("write buffer (\"\")"), error in (no error)=w1628) -> (VISA resource name out=w1625:refnum<visa-resource-name>, error out=w1627:errorcluster)  [unwired: 1 out]
        n399 = call <vilib>:"compatOverwrite.vi"("overwrite (F)"=TRUE) -> ("overwrite?"=w1614:T7)
        n400 = Open/Create/Replace File(file path (use dialog)=w1635, error in=w1627, operation (0:open)=w1614) -> (refnum out=w1638:refnum<file>, error out=w1637:errorcluster)  [unwired: 3 in, 1 out]
        n401 = call "4155C Write array to file.vi"("Byte Stream File Refnum"=w1638, "Header"=string[] ["I stress completed successfully", ""], "error in (no error)"=w1637) -> ("dup refnum"=w1640:refnum<file>, "error out"=w1639:errorcluster)  [unwired: 2 in]
        n402 = Close File(refnum=w1640, error in=w1639) -> (error out=w1633:errorcluster)  [unwired: 1 out]
      }
      frame "vsu2pulse" {
        n403 = Number To Decimal String(number=w1673) -> (decimal integer string=w1708:string)  [unwired: 1 in]
        n404 = Concatenate Strings(w1693, "-vsu2-" ("Substring"), w1708, w1672, ".txt" ("Substring")) -> (w1706:string)
        n405 = Fract/Exp String To Number(string=w1705) -> (number=w1681:dbl[])  [unwired: 3 in, 1 out]
        n406 = String To Path(string=w1706) -> (path=w1697:path)
        n407 = Index Array(array=w1681, index=1 ("Index")) -> (element=w1680:dbl)
        n408 = Index Array(array=w1681, index=0 ("Index")) -> (element=w1678:dbl)
        n409 = call "4155C Config VSU2 Stress.vi"("error in (no error)"=w1710, "VSU2"=w1678, "Display on/off"=TRUE, "VISA session"=w1711) -> ("error out"=w1712:errorcluster, "dup VISA resource name"=w1713:refnum<visa-resource-name>)
        n410 = call "4155C Apply Stress.vi"("error in (no error)"=w1712, "Duration"=w1680, "Emergency Stop"=w1692, "VISA resource name in"=w1713) -> ("error out"=w1690:errorcluster, "VISA Resource Name out"=w1688:refnum<visa-resource-name>)
        n411 = VISA Write(VISA resource name=w1688, write buffer=":DISP ON" ("write buffer (\"\")"), error in (no error)=w1690) -> (VISA resource name out=w1687:refnum<visa-resource-name>, error out=w1689:errorcluster)  [unwired: 1 out]
        n412 = call <vilib>:"compatOverwrite.vi"("overwrite (F)"=TRUE) -> ("overwrite?"=w1677:T7)
        n413 = Open/Create/Replace File(file path (use dialog)=w1697, error in=w1689, operation (0:open)=w1677) -> (refnum out=w1700:refnum<file>, error out=w1699:errorcluster)  [unwired: 3 in, 1 out]
        n414 = call "4155C Write array to file.vi"("Byte Stream File Refnum"=w1700, "Header"=string[] ["VSU2 pulse completed successfully", ""], "error in (no error)"=w1699) -> ("dup refnum"=w1702:refnum<file>, "error out"=w1701:errorcluster)  [unwired: 2 in]
        n415 = Close File(refnum=w1702, error in=w1701) -> (error out=w1695:errorcluster)  [unwired: 1 out]
      }
      frame "sample-fpp" {
        w1745 = string[] ["Time /s", "Id VgVd /A", "Ig VgVd /A", "Vp1 VgVd /V", "Vp2 VgVd /V"] ("Header")
        w1749 = "%d" ("format string")
        n416 = Number To Decimal String(number=w1734) -> (decimal integer string=w1797:string)  [unwired: 1 in]
        n417 = Fract/Exp String To Number(string=w1794) -> (number=w1782:dbl[])  [unwired: 3 in, 1 out]
        n418 = Concatenate Strings(w1788, "-samplefpp-" ("Substring"), w1797, w1733, ".txt" ("Substring")) -> (w1795:string)
        n419 = String To Path(string=w1795) -> (path=w1757:path)
        n420 = Index Array(array=w1782, index=0 ("Index")) -> (element=w1743:dbl)
        n421 = Index Array(array=w1782, index=1 ("Index")) -> (element=w1742:dbl)
        n422 = Index Array(array=w1782, index=2 ("Index")) -> (element=w1790:dbl)
        n423 = Index Array(array=w1782, index=3 ("Index")) -> (element=w1780:dbl)
        n424 = call "4155C Config Sampling Measurements FPP.vi"("VISA session"=w1800, "Num Points"=w1790, "Vg"=w1743, "Display on/off"=TRUE, "Gate Compliance"=w1789, "Drain Compliance"=w1798, "Standby"="Standby", "error in (no error)"=w1799, "Timings"=w1787, "Vd"=w1742, "Sample time"=w1780) -> ("dup VISA resource name"=w1759:refnum<visa-resource-name>, "error out"=w1758:errorcluster)  [unwired: 3 in]
        n425 = Number To Decimal String(number=w1743) -> (decimal integer string=w1769:string)  [unwired: 1 in]
        n426 = call "4155C Take Sample FPP.vi"("VISA resource name in"=w1759, "error in (no error)"=w1758, "Emergency Stop"=w1760) -> ("Time"=w1764:dbl[], "Vp1"=w1774:dbl[], "VISA Resource Name out"=w1740:refnum<visa-resource-name>, "Ig"=w1762:dbl[], "Id"=w1763:dbl[], "Vp2"=w1772:dbl[], "error out"=w1761:errorcluster)  [unwired: 10 in]
        n427 = Insert Into Array(array=dbl[][] [] ("Input Array"), new element=w1764) -> (w1778:dbl[][])  [unwired: 2 in]
        n428 = Number To Decimal String(number=w1742) -> (decimal integer string=w1767:string)  [unwired: 1 in]
        n429 = Insert Into Array(array=w1778, new element=w1763) -> (w1777:dbl[][])  [unwired: 2 in]
        n430 = Concatenate Strings("(Vg = " ("Substring"), w1769, "V, Vd = " ("Substring"), w1767, "V)" ("Substring")) -> (w1765:string)
        n431 = Insert Into Array(array=w1777, new element=w1762) -> (w1776:dbl[][])  [unwired: 2 in]
        n432 = Insert Into Array(array=w1776, new element=w1774) -> (w1773:dbl[][])  [unwired: 2 in]
        n433 = Insert Into Array(array=w1773, new element=w1772) -> (w1741:dbl[][])  [unwired: 2 in]
        n434 = Transpose 2D Array(2D array=w1741) -> (transposed array=w1771:dbl[][])
        n435 = call <vilib>:"compatOverwrite.vi"("overwrite (F)"=TRUE) -> ("overwrite?"=w1738:T7)
        n436 = Open/Create/Replace File(file path (use dialog)=w1757, error in=w1761, operation (0:open)=w1738) -> (refnum out=w1754:refnum<file>, error out=w1755:errorcluster)  [unwired: 3 in, 1 out]
        n437 = Array To Spreadsheet String(array=w1745, 3:w1749) -> (spreadsheet string=w1751:string)  [unwired: 1 in]
        n438 = Search and Replace String(replace all?=TRUE ("replace all? (F)"), input string=w1751, search string="VgVd", replace string=w1765) -> (result string=w1747:string)  [unwired: 4 in, 3 out]
        n439 = Spreadsheet String To Array(format string=w1749, spreadsheet string=w1747, array type (2D Dbl)=w1745) -> (array=w1746:string[])  [unwired: 1 in]
        n440 = call "4155C Write array to file.vi"("Byte Stream File Refnum"=w1754, "Header"=w1746, "Data Array"=w1771, "error in (no error)"=w1755) -> ("dup refnum"=w1752:refnum<file>, "error out"=w1753:errorcluster)  [unwired: 1 in]
        n441 = Close File(refnum=w1752, error in=w1753) -> (error out=w1739:errorcluster)  [unwired: 1 out]
      }
      frame "resample-fpp" {
        w1834 = string[] ["Time /s", "Id VgVd /A", "Ig VgVd /A", "Vp1 VgVd /V", "Vp2 VgVd /V"] ("Header")
        w1838 = "%d" ("format string")
        n442 = Number To Decimal String(number=w1820) -> (decimal integer string=w1878:string)  [unwired: 1 in]
        n443 = Fract/Exp String To Number(string=w1875) -> (number=w1827:dbl[])  [unwired: 3 in, 1 out]
        n444 = Concatenate Strings(w1871, "-resamplefpp-" ("Substring"), w1878, w1821, ".txt" ("Substring")) -> (w1876:string)
        n445 = String To Path(string=w1876) -> (path=w1846:path)
        n446 = Index Array(array=w1827, index=0 ("Index")) -> (element=w1833:dbl)
        n447 = Index Array(array=w1827, index=1 ("Index")) -> (element=w1832:dbl)
        n448 = Number To Decimal String(number=w1833) -> (decimal integer string=w1856:string)  [unwired: 1 in]
        n449 = call "4155C Take Sample FPP.vi"("VISA resource name in"=w1829, "error in (no error)"=w1828, "Emergency Stop"=w1847) -> ("Time"=w1851:dbl[], "Vp1"=w1861:dbl[], "VISA Resource Name out"=w1831:refnum<visa-resource-name>, "Ig"=w1849:dbl[], "Id"=w1850:dbl[], "Vp2"=w1859:dbl[], "error out"=w1848:errorcluster)  [unwired: 10 in]
        n450 = Insert Into Array(array=dbl[][] [] ("Input Array"), new element=w1851) -> (w1865:dbl[][])  [unwired: 2 in]
        n451 = Number To Decimal String(number=w1832) -> (decimal integer string=w1854:string)  [unwired: 1 in]
        n452 = Insert Into Array(array=w1865, new element=w1850) -> (w1864:dbl[][])  [unwired: 2 in]
        n453 = Concatenate Strings("(Vg = " ("Substring"), w1856, "V, Vd = " ("Substring"), w1854, "V)" ("Substring")) -> (w1852:string)
        n454 = Insert Into Array(array=w1864, new element=w1849) -> (w1863:dbl[][])  [unwired: 2 in]
        n455 = Insert Into Array(array=w1863, new element=w1861) -> (w1860:dbl[][])  [unwired: 2 in]
        n456 = Insert Into Array(array=w1860, new element=w1859) -> (w1826:dbl[][])  [unwired: 2 in]
        n457 = call <vilib>:"compatOverwrite.vi"("overwrite (F)"=TRUE) -> ("overwrite?"=w1825:T7)
        n458 = Open/Create/Replace File(file path (use dialog)=w1846, error in=w1848, operation (0:open)=w1825) -> (refnum out=w1843:refnum<file>, error out=w1844:errorcluster)  [unwired: 3 in, 1 out]
        n459 = Array To Spreadsheet String(array=w1834, 3:w1838) -> (spreadsheet string=w1840:string)  [unwired: 1 in]
        n460 = Transpose 2D Array(2D array=w1826) -> (transposed array=w1858:dbl[][])
        n461 = Search and Replace String(replace all?=TRUE ("replace all? (F)"), input string=w1840, search string="VgVd", replace string=w1852) -> (result string=w1836:string)  [unwired: 4 in, 3 out]
        n462 = Spreadsheet String To Array(format string=w1838, spreadsheet string=w1836, array type (2D Dbl)=w1834) -> (array=w1835:string[])  [unwired: 1 in]
        n463 = call "4155C Write array to file.vi"("Byte Stream File Refnum"=w1843, "Header"=w1835, "Data Array"=w1858, "error in (no error)"=w1844) -> ("dup refnum"=w1841:refnum<file>, "error out"=w1842:errorcluster)  [unwired: 1 in]
        n464 = Close File(refnum=w1841, error in=w1842) -> (error out=w1830:errorcluster)  [unwired: 1 out]
      }
      frame "serial" {
        n465 = local read "Termination char\n(0xA = '\\n' = LF)\n(0xD = '\\r' = CR)"() -> (w1906:u8)
        n466 = local read "Enable Termination\nChar (T)"() -> (w1907:bool)
        n467 = Index Array(array=w1914, index=0 ("Index")) -> (element=w1913:string)
        n468 = local read "parity"() -> (w1897:u16)
        n469 = local read "Delay before read (ms)"() -> (w1908:u32)
        n470 = local read "byte count"() -> (w1905:u32)
        n471 = local read "Timeout (ms)"() -> (w1904:u32)
        n472 = local read "VISA resource name"() -> (w1901:refnum<visa-resource-name>)
        n473 = local read "baud rate"() -> (w1900:u32)
        n474 = local read "Serial End Mode for Reads"() -> (w1899:u16)
        n475 = local read "data bits"() -> (w1898:u16)
        n476 = local read "stop bits"() -> (w1903:u16)
        n477 = local read "flow control"() -> (w1902:u16)
        n478 = call "Serial write and read v0.5.vi"("Delay before read (ms)"=w1908, "Termination char\n(0xA = '\\n' = LF)\n(0xD = '\\r' = CR)"=w1906, "Enable Termination\nChar (T)"=w1907, "parity"=w1897, "stop bits"=w1903, "string to write"=w1913, "flow control"=w1902, "byte count"=w1905, "Serial Settings:Serial End Mode for Reads"=w1899, "Timeout (ms)"=w1904, "error in (no error)"=w1919, "VISA resource name"=w1901, "baud rate"=w1900, "data bits"=w1898) -> ("Serial port output"=w1909:string, "error out"=w1918:errorcluster)
        n479 = Build Array (concatenate)(w1909, w1910) -> (w1911:string[])
      }
      frame "pump" {
        # "Time array for valve position"
        # "Time array for absolute plunger position"
        # "Valve position"
        # "Absolute plunger position"
        # "Remove \"_\""
        # "Check if hard stop is pressed."
        # "Check if halt is pressed."
        # "Check if pump is idle. Else halt."
        n480 = Index Array(array=w1984, index=0 ("Index")) -> (element=w1961:string)
        n481 = case shown="\"No error\", Default" w1959 {
          tunnel: w1961 -> [w2020 _ w2022 w2023 w2024 w2025 _ _ w2028 w2029 _]
          tunnel: [w2020 "/1H" w2022 w2023 w2024 w2025 "/1H" "/1H" w2028 w2029 "/1H"] -> w1960
          frame "No error", Default {
          }
          frame "Initialization" {
          }
          frame "Invalid command" {
          }
          frame "Invalid operand" {
          }
          frame "Device not initialized" {
          }
          frame "Internal failure" {
          }
          frame "Plunger overload" {
          }
          frame "Valve overload" {
          }
          frame "Plunger move not allowed" {
          }
          frame "A/D converter failure" {
          }
          frame "Command overflow" {
          }
        }
        n482 = local read "Hard stop pump"() -> (w1963:bool)
        n483 = local read "Halt pump"() -> (w1966:bool)
        n484 = local read "Serial End Mode for Reads"() -> (w1972:u16)
        n485 = local read "flow control"() -> (w1975:u16)
        n486 = local read "stop bits"() -> (w1976:u16)
        n487 = local read "parity"() -> (w1970:u16)
        n488 = local read "Delay before read (ms)"() -> (w1981:u32)
        n489 = local read "byte count"() -> (w1978:u32)
        n490 = local read "Timeout (ms)"() -> (w1977:u32)
        n491 = local read "VISA resource name"() -> (w1974:refnum<visa-resource-name>)
        n492 = local read "baud rate"() -> (w1973:u32)
        n493 = local read "Enable Termination\nChar (T)"() -> (w1980:bool)
        n494 = local read "Termination char\n(0xA = '\\n' = LF)\n(0xD = '\\r' = CR)"() -> (w1979:u8)
        n495 = case shown="True" w1966 {
          tunnel: [w2034 "/1H"] -> w1965
          tunnel: w1960 -> [w2034 _]
          frame False {
          }
          frame True {
            n496 = local write "Halt pump"(FALSE) -> ()
          }
        }
        n497 = case shown="True" w1963 {
          tunnel: [w2031 "/1T"] -> w1964
          tunnel: w1965 -> [w2031 _]
          frame False {
          }
          frame True {
            n498 = local write "Hard stop pump"(FALSE) -> ()
          }
        }
        n499 = local read "data bits"() -> (w1971:u16)
        n500 = String Subset(string=w1955, offset (0)=1) -> (substring=w1953:string)  [unwired: 1 in]
        n501 = call "SPM Pump v0.6.vi"("Termination char\n(0xA = '\\n' = LF)\n(0xD = '\\r' = CR)"=w1979, "Enable Termination\nChar (T)"=w1980, "Timeout (ms)"=w1977, "Serial Settings:Serial End Mode for Reads"=w1972, "byte count"=w1978, "Delay before read (ms)"=w1981, "Time <input>"=w1958, "error in (no error)"=w1989, "Serial port input"=w1964, "VISA resource name"=w1974, "parity"=w1970, "baud rate"=w1973, "stop bits"=w1976, "data bits"=w1971, "flow control"=w1975, "Time units <input>"=w1953) -> ("Input command"=w1952:string, "Serial port data"=w1942:string[], "Pump status"=w1948:string, "Valve position"=w1950:i32, "Absolute plunger position"=w1962:i32, "Serial port"=w1957:string, "error out"=w1988:errorcluster)  [unwired: 1 in, 4 out]
        n502 = case shown="\"?6\"" w1952 {
          tunnel: [w2001 w2009 w2015] -> w1969
          tunnel: w1968 -> [w2001 w2008 w2015]
          tunnel: w1962 -> [_ w2007 _]
          tunnel: w1949 -> [w2000 w2006 w2016]
          tunnel: [w2000 w2006 w2018] -> w1951
          tunnel: w1950 -> [_ _ w2017]
          tunnel: w1947 -> [_ w2005 w2013]
          tunnel: w1946 -> [w1999 w2004 w2014]
          tunnel: [w1999 w2003 w2014] -> w1945
          tunnel: [w1998 w2002 w2012] -> w1944
          tunnel: w1943 -> [w1998 w2002 w2011]
          frame "Q", Default {
          }
          frame "?" {
            n503 = Build Array (concatenate)(w2008, w2007) -> (w2009:i32[])
            n504 = Build Array (concatenate)(w2004, w2005) -> (w2003:i32[])
            n505 = call "4155C Split array.vi"("X data in"=w2003, "Y1 data in"=w2009) -> ("Array of clusters"=w2010:cluster{"Y data in":dbl[], "X data in":dbl[]}[])  [unwired: 5 in, 1 out]
            n506 = local write "Absolute plunger position vs time"(w2010) -> ()
          }
          frame "?6" {
            n507 = Build Array (concatenate)(w2016, w2017) -> (w2018:i32[])
            n508 = Build Array (concatenate)(w2011, w2013) -> (w2012:i32[])
            n509 = call "4155C Split array.vi"("X data in"=w2012, "Y1 data in"=w2018) -> ("Array of clusters"=w2019:cluster{"Y data in":dbl[], "X data in":dbl[]}[])  [unwired: 5 in, 1 out]
            n510 = local write "Valve position vs time"(w2019) -> ()
          }
        }
        n511 = Build Array (concatenate)(w1940, w1942) -> (w1941:string[][])
        n512 = Build Array (concatenate)(w1956, w1957) -> (w1982:string[])
      }
      frame "filename" {
        n513 = Index Array(array=w2038, index=0 ("Index")) -> (element=w2037:string)
      }
    }
    n514 = Build Array(w137, w66, w76, w75, w74, w73, w72, w71, w70, w69, w68, w67, w65) -> (w176:dbl[][])
    n515 = Transpose 2D Array(2D array=w176) -> (transposed array=w175:dbl[][])
    n516 = Concatenate Strings(w117, w60, "Imax_Imin_Ion_Ioff_vs_time.txt" ("Suffix (Imax,Imin,Ion,Ioff)")) -> (w186:string)
    n517 = Build Array(w98, "Is max (A)" ("VAR2 Name"), "Is min (A)" ("VAR2 Name"), "Id max (A)" ("VAR2 Name"), "Id min (A)" ("VAR2 Name"), "Ig max (A)" ("VAR2 Name"), "Ig min (A)" ("VAR2 Name"), "Is on (A)" ("VAR2 Name"), "Is off (A)" ("VAR2 Name"), "Id on (A)" ("VAR2 Name"), "Id off (A)" ("VAR2 Name"), "Ig on (A)" ("VAR2 Name"), "Ig off (A)" ("VAR2 Name")) -> (w181:string[])
    n518 = Array To Spreadsheet String(array=w175, 3:"%e" ("format string")) -> (spreadsheet string=w179:string)  [unwired: 1 in]
    n519 = Array To Spreadsheet String(array=w181, 3:"" ("format string")) -> (spreadsheet string=w180:string)  [unwired: 1 in]
    n520 = String To Path(string=w186) -> (path=w185:path)
    n521 = Build Array(w180, w179) -> (w178:string[])
    n522 = Write to Text File(file (use dialog)=w185, text=w178, error in=w133) -> (refnum out=w187:refnum<file>, error out=w177:errorcluster)  [unwired: 1 in, 1 out]
    n523 = Close File(refnum=w187, error in=w177) -> (error out=w116:errorcluster)  [unwired: 1 out]
    n524 = Build Array(w112, w138) -> (w143:i32[][])
    n525 = Build Array(w98, "Absolute plunger position" ("VAR2 Name")) -> (w146:string[])
    n526 = Transpose 2D Array(2D array=w143) -> (transposed array=w136:i32[][])
    n527 = Array To Spreadsheet String(array=w146, 3:"" ("format string")) -> (spreadsheet string=w145:string)  [unwired: 1 in]
    n528 = Array To Spreadsheet String(array=w136, 3:"%e" ("format string")) -> (spreadsheet string=w142:string)  [unwired: 1 in]
    n529 = Build Array(w145, w142) -> (w148:string[])
    n530 = Concatenate Strings(w117, w60, "plunger_vs_time.txt" ("Suffix (plunger)")) -> (w140:string)
    n531 = String To Path(string=w140) -> (path=w139:path)
    n532 = Write to Text File(file (use dialog)=w139, text=w148, error in=w116) -> (refnum out=w141:refnum<file>, error out=w150:errorcluster)  [unwired: 1 in, 1 out]
    n533 = Close File(refnum=w141, error in=w150) -> (error out=w115:errorcluster)  [unwired: 1 out]
    n534 = Concatenate Strings(w117, w60, "serial_port_output.txt" ("Suffix (serial port log)")) -> (w156:string)
    n535 = String To Path(string=w156) -> (path=w155:path)
    n536 = Build Array(w98, "Serial port input" ("VAR2 Name"), "Pump status" ("VAR2 Name"), "Serial port output: ") -> (w102:string[])
    n537 = Array To Spreadsheet String(array=w108, 3:"" ("format string")) -> (spreadsheet string=w99:string)  [unwired: 1 in]
    n538 = Array To Spreadsheet String(array=w102, 3:"" ("format string")) -> (spreadsheet string=w100:string)  [unwired: 1 in]
    n539 = Build Array(w100, w99) -> (w101:string[])
    n540 = Array To Spreadsheet String(array=w107, 3:"" ("format string")) -> (spreadsheet string=w161:string)  [unwired: 1 in]
    n541 = Write to Text File(file (use dialog)=w155, text=w101, error in=w115) -> (refnum out=w157:refnum<file>, error out=w158:errorcluster)  [unwired: 1 in, 1 out]
    n542 = Close File(refnum=w157, error in=w158) -> (error out=w114:errorcluster)  [unwired: 1 out]
    n543 = local write "Serial port data"(w161) -> ()
    n544 = Build Array(w111, w119) -> (w125:i32[][])
    n545 = Build Array(w98, "Valve port" ("VAR2 Name")) -> (w128:string[])
    n546 = Transpose 2D Array(2D array=w125) -> (transposed array=w120:i32[][])
    n547 = Array To Spreadsheet String(array=w128, 3:"" ("format string")) -> (spreadsheet string=w127:string)  [unwired: 1 in]
    n548 = Array To Spreadsheet String(array=w120, 3:"%e" ("format string")) -> (spreadsheet string=w124:string)  [unwired: 1 in]
    n549 = Build Array(w127, w124) -> (w130:string[])
    n550 = Concatenate Strings(w117, w60, "valve_port_vs_time.txt" ("Suffix (valve)")) -> (w122:string)
    n551 = String To Path(string=w122) -> (path=w121:path)
    n552 = Write to Text File(file (use dialog)=w121, text=w130, error in=w114) -> (refnum out=w123:refnum<file>, error out=w132:errorcluster)  [unwired: 1 in, 1 out]
    n553 = Close File(refnum=w123, error in=w132) -> (error out=w113:errorcluster)  [unwired: 1 out]
  }
  "error out" <- w18
